vi "Omniax_mDrive_XYZR_MM_BR_RES_2_NC_GR_pxi_Acc3_preset.vi"() -> ()   [LabVIEW 2010]
uses:
  <vilib>/Utility/file.llb/Read From Spreadsheet File (I64).vi
  <vilib>/Utility/file.llb/Read From Spreadsheet File (string).vi
  <vilib>/Instr/_visa.llb/VISA Configure Serial Port (Instr).vi
  <vilib>/Utility/file.llb/Write To Spreadsheet File (I64).vi
  <vilib>/Utility/file.llb/Write To Spreadsheet File (string).vi
panel:
  out "R Velocity MVdeg/sec":dbl format="%.3f"
  out "R Position MV deg":dbl
  out "Z Velocity MV mm/sec":dbl format="%.3f"
  out "Z Position MV mm":dbl
  out "Y Velocity MV mm/sec":dbl format="%.3f"
  out "Y Position MV mm":dbl
  out "X Velocity MV mm/sec":dbl format="%.3f"
  out "X Position MV mm":dbl
  out "Presets":i32[][](array[numeric])
  in  "stop":bool
  in  "Tab Control 3":enum32{"Status", "Reset"}(tab)
  out "Y in Range":bool
  out "Y Scan":bool
  out "Y in Motion":bool
  out "Y Backlash corr":bool
  out "X  in Range":bool
  out "X Scan":bool
  out "X  in Motion":bool
  out "X Backlash corr":bool
  out "Z in Range":bool
  out "Z Scan":bool
  out "Z in Motion":bool
  out "Z Backlash corr":bool
  out "R in Range":bool
  out "R Scan":bool
  out "R in Motion":bool
  out "R Backlash corr":bool
  out "X Ready":bool
  out "Y Ready":bool
  out "Z Ready":bool
  out "R Ready":bool
  in  "Reset Y Position mm":dbl
  out "Reset Y Motor Steps":i32
  in  "Reset X Position mm":dbl
  out "Reset X Motor Steps":i32
  in  "Reset Z Position mm":dbl
  out "Reset Z Motor Steps":i32
  in  "Reset R Position deg":dbl
  out "Reset R Motor Steps":i32
  in  "Reset":bool
  in  "Tab Control 2":enum32{"mm", "step"}(tab)
  in  "X Scan Length SP mm":dbl
  in  "X Scan Velocity SP mm/sec":dbl
  in  "X Scan set":bool
  in  "Y Scan Length SP mm":dbl
  in  "Y Scan Velocity SP mm/sec":dbl
  in  "Y Scan set":bool
  in  "Z Scan Length SP mm":dbl
  in  "Z Scan Velocity SP mm/sec":dbl
  in  "Z Scan set":bool
  in  "R Scan Length SP deg":dbl
  in  "R Scan Velocity SP deg/sec":dbl
  in  "R Scan set":bool
  in  "X Scan Velocity SP steps/sec":i32=1 min=1 max=102400 step=1
  in  "X Scan Length SP steps":i32 min=-2304000 max=2304000 step=100
  out "X Scan length MV mm":dbl
  out "X Scan velocity MV mm/sec":dbl format="%#_6f"
  in  "Y Scan Velocity SP steps/sec":i32=1 min=1 max=102400 step=1
  in  "Y Scan Length SP steps":i32 min=-2304000 max=2304000 step=100
  out "Y Scan length MV mm":dbl
  out "Y Scan velocity MV mm/sec":dbl format="%#_6f"
  in  "Z Scan Velocity SP steps/sec":i32=1 min=1 max=102400 step=1
  in  "Z Scan Length SP steps":i32 min=-5120000 max=97280000 step=100
  out "Z Scan length MV mm":dbl
  out "Z Scan velocity MV mm/sec":dbl format="%#_6f"
  in  "R Scan Velocity SP steps/sec":i32=1 min=1 max=102400 step=1
  in  "R Scan Length SP steps":i32 min=-6144000 max=0 step=100
  out "R Scan length MV deg":dbl
  out "R Scan velocity MV deg/sec":dbl format="%#_6f"
  out "atan Y/Z":dbl
  in  "Tab Control":enum32{"mm", "preset", "step"}(tab)
  in  "X Position SP mm":dbl
  in  "X Velocity SP mm/sec":dbl
  in  "X Move Set":bool
  in  "Y Move Set":bool
  in  "Y Position SP mm":dbl
  in  "Y Velocity SP mm/sec":dbl
  in  "Z Position SP mm":dbl
  in  "Z Velocity SP mm/sec":dbl
  in  "Z Move Set":bool
  in  "R Position SP deg":dbl
  in  "R Velocity SP deg/sec":dbl
  in  "R Move Set":bool
  in  "Add Button":bool
  in  "String":string
  in  "Delete Button":bool
  in  "Preset positions":i32(ring) items=["ZERO", "Default", "CDOSE", "QMS", "test", "test2", "test3", "yag position", "Sample Long Edge  ", "SPUTTER POS"]
  in  "Set Button":bool
  in  "X Velocity SP step/sec":i32 min=1 max=128000
  in  "Y Velocity SP step/sec":i32 min=1 max=128000
  in  "Z Velocity SP step/sec":i32 min=1 max=204800
  in  "R Velocity SP step/sec":i32 min=1 max=20000
  in  "Y Step SP":i32=-20000 min=-2304000 max=2304000 step=500
  in  "X Step SP":i32=-20000 min=-2304000 max=2304000 step=500
  in  "Z Step SP":i32=-20000 min=0 max=102400000 step=500
  in  "R Step SP":i32=-20000 min=-6144000 max=6144000 step=500
  out "X Step PV":i32 max=2000
  out "Y Step PV":i32 max=2000
  out "Z Step PV":i32 max=2000
  out "R Step PV":i32 max=2000
  in  "Clear ZY":bool
  out "ZY Graph":cluster{"Y":dbl[], "Y":dbl[]}[](graph)
  out "ZR Graph":cluster{"Y":dbl[], "Y":dbl[]}[](graph)
  out "XY Graph":cluster{"Y":dbl[], "Y":dbl[]}[](graph)
  out "X Scan Duration":dbl
  out "Y Scan Duration":dbl
  out "Z Scan Duration":dbl
  out "R Scan Duration":dbl
  out "R Backlash steps/sec":i32
  out "R Backlash":i32
  out "R Holding Current %":i32
  out "R Run Current %":i32
  out "R offset deg":dbl
  out "R deg/rev":dbl
  out "R steps/rev":u32
  out "R velocity PV step/sec":i32
  out "R MINPOS":i32=-94296
  out "R MAXPOS":i32=-34296
  out "R COM PORT":refnum<visa-resource-name>="COM5"
  in  "R Scan OK":bool
  in  "R Go":bool
  out "R Position deg PV":dbl
  out "Z COM PORT":refnum<visa-resource-name>="COM5"
  out "Z Backlash steps/sec":i32
  out "Z Backlash":i32
  out "Z Holding Current %":i32
  out "Z Run Current %":i32
  out "Z offset mm":dbl
  out "Z mm/rev":dbl
  out "Z steps/rev":u32
  out "Z  velocity PV step/sec":i32
  out "Z MINPOS":i32=-94296
  out "Z MAXPOS":i32=-34296
  in  "Z Scan OK":bool
  in  "Z Go":bool
  out "Z Position mm PV":dbl
  out "X Position mm PV":dbl
  out "X velocity PV step/sec":i32
  in  "X Scan OK":bool
  in  "X Go":bool
  out "X Backlash steps/sec":i32
  out "X Backlash":i32
  out "X Holding Current %":i32
  out "X Run Current %":i32
  out "X offset mm":dbl
  out "X mm/rev":dbl
  out "X steps/rev":u32
  out "X MAXPOS":i32=-34296
  out "X MINPOS":i32=-94296
  out "X COM PORT":refnum<visa-resource-name>="COM5"
  out "Y Backlash steps/sec":i32
  out "Y Backlash":i32
  out "Y Holding Current %":i32
  out "Y Run Current %":i32
  in  "Scan Cancel":bool
  out "Y Position mm PV":dbl
  out "Y offset mm":dbl
  out "Y mm/rev":dbl
  out "Y steps/rev":u32
  out "Y velocity PV step/sec":i32
  in  "Y Scan OK":bool
  in  "Scan Go":bool
  in  "Stop":bool
  in  "Y Go":bool
  out "Y MINPOS":i32=-94296
  out "Y MAXPOS":i32=-34296
  out "Y COM PORT":refnum<visa-resource-name>="COM5"
  # "Current position"
  # "Goto position"
  # "MX"
  # "MY"
  # "MZ"
  # "MR"
  # "L"
  # "M"
  # "B"
  # "S"
  # "R"
  # "Preset position"
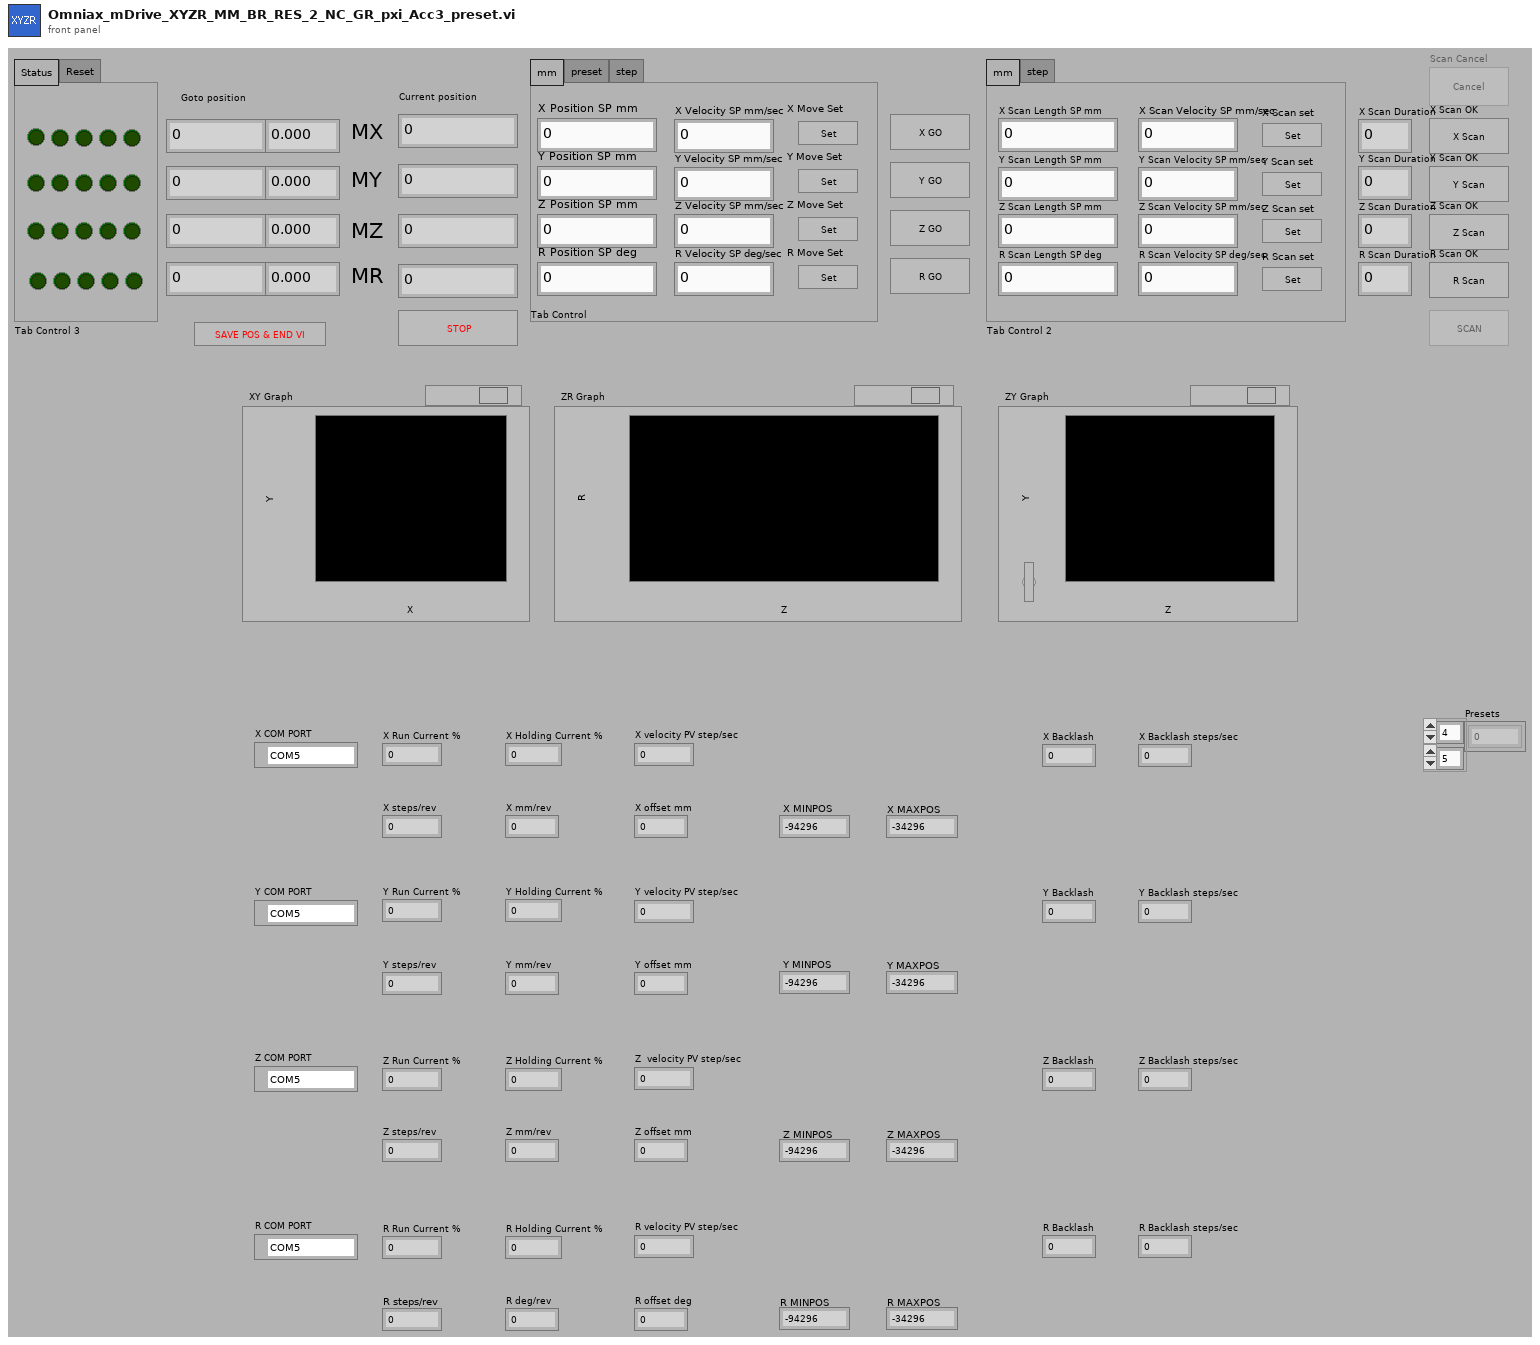
[diagram p1: front panel]
types:
  T1 = enum16{"Stop", "Reset", "Run Current", "Holding Current", "Accel Rate", "Decel Rate", "Move to Relative Position", "Move to Absolute Position", "Echo Mode", "Print Parameter", "Send String", "Microstep Resolution", "Set Current Position", "Max Velocity"}
  T2 = enum8{"Enabled", "Disabled", "Disabled and Grayed Out"}
  T3 = cluster{"first row[0]":i64, "first row[1]":i64, "first row[2]":i64, "first row[3]":i64, "first row[4]":i64, "first row[5]":i64, "first row[6]":i64, "first row[7]":i64, "first row[8]":i64}
  T4 = cluster{"Value[0]":i32, "Value[1]":i32, "Value[2]":i32, "Value[3]":i32, "Value[4]":i32, "Value[5]":i32, "Value[6]":i32, "Value[7]":i32, "Value[8]":i32}
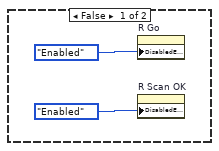
[diagram p5: hidden frame]
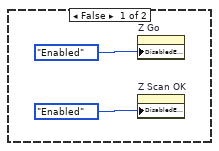
[diagram p8: hidden frame]
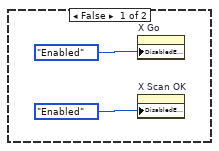
[diagram p11: hidden frame]
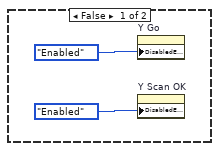
[diagram p14: hidden frame]
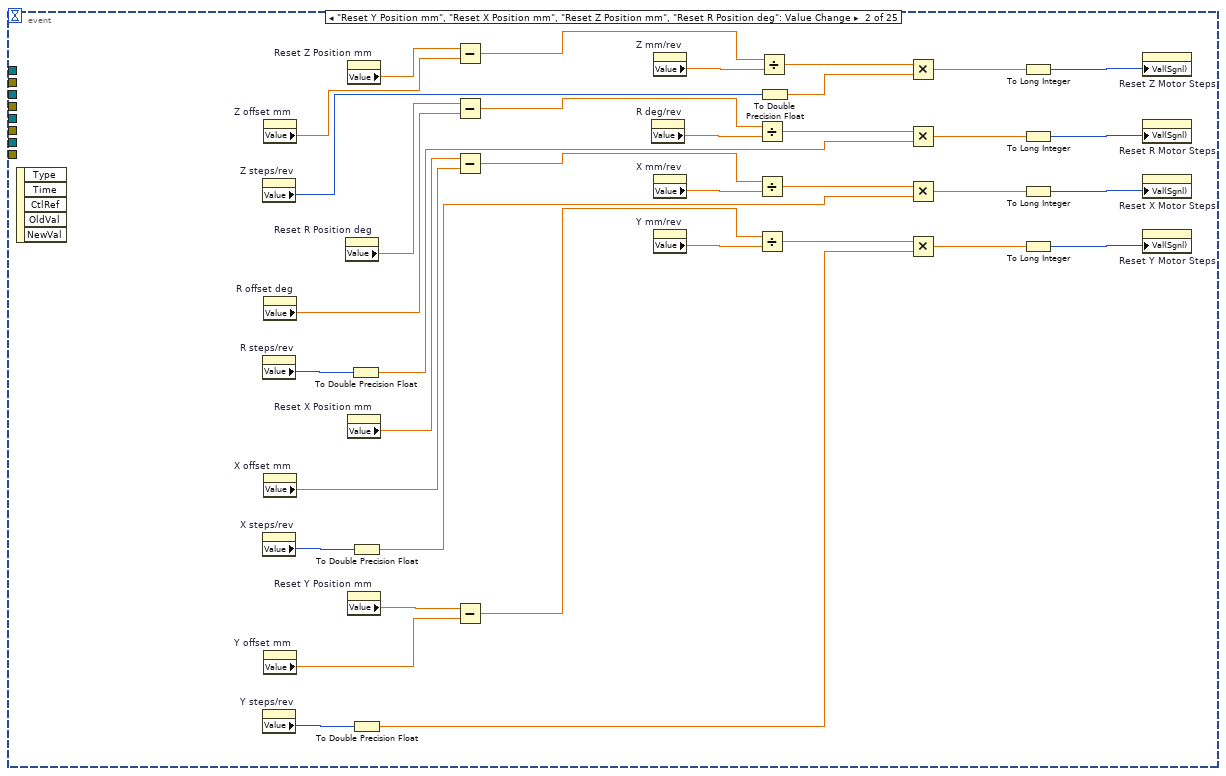
[diagram p17: hidden frame]
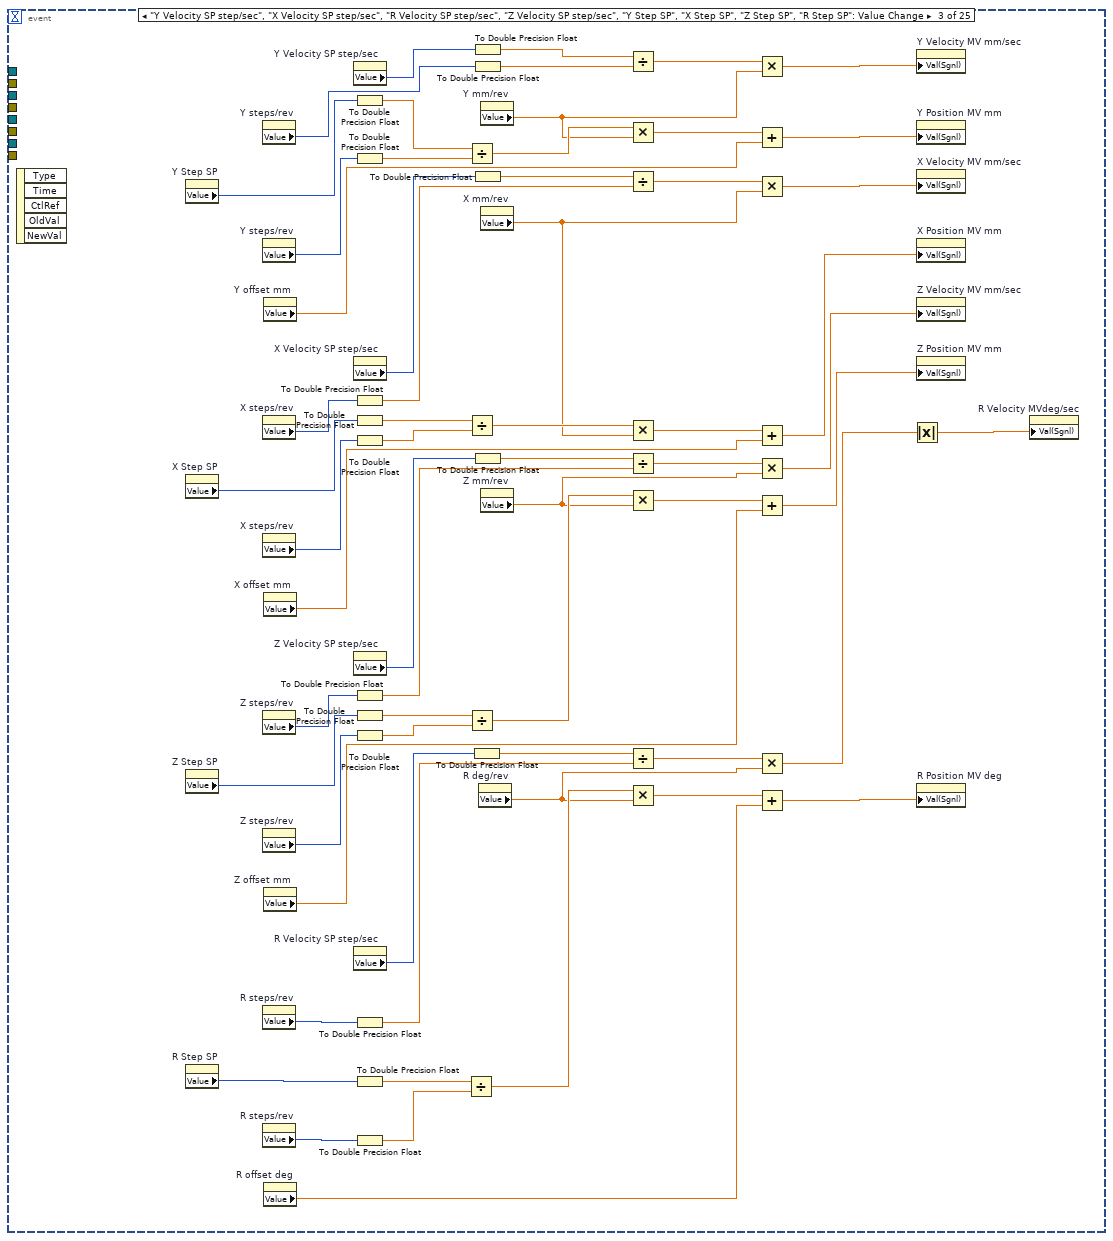
[diagram p18: hidden frame]
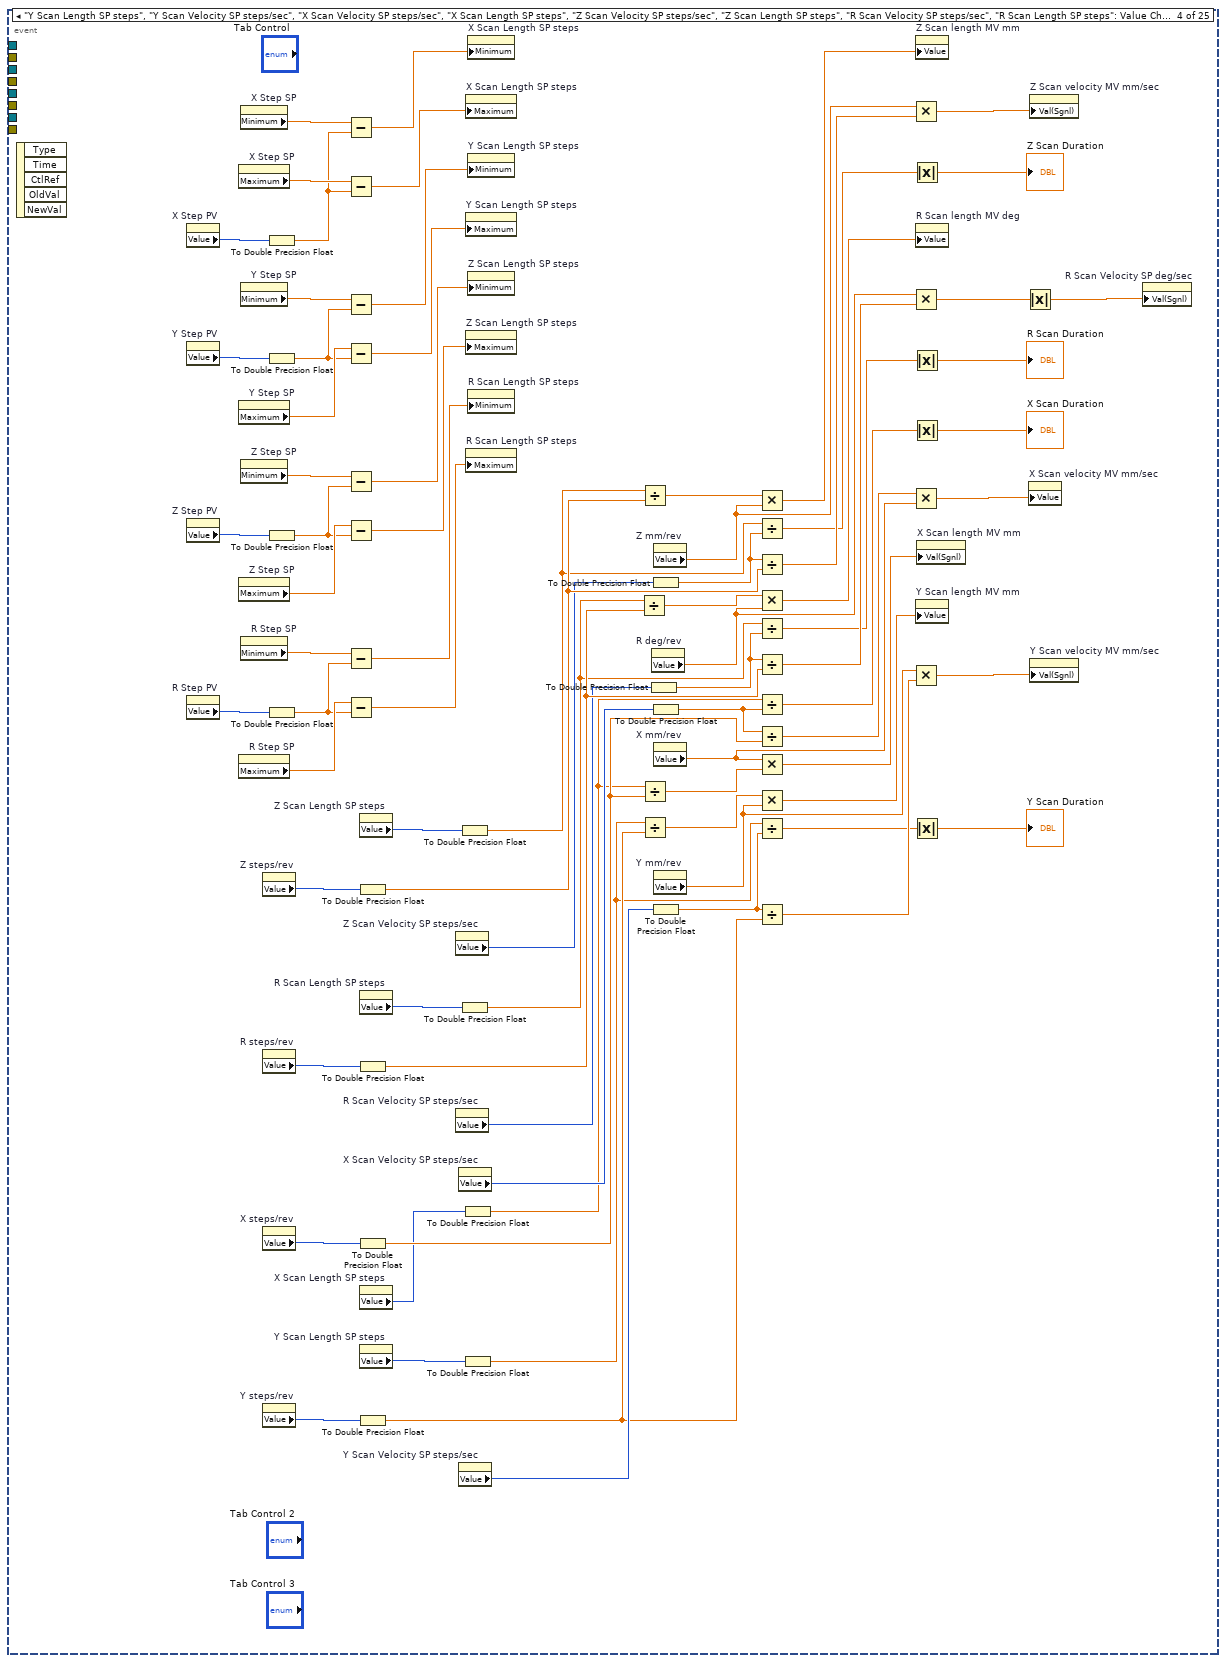
[diagram p19: hidden frame]
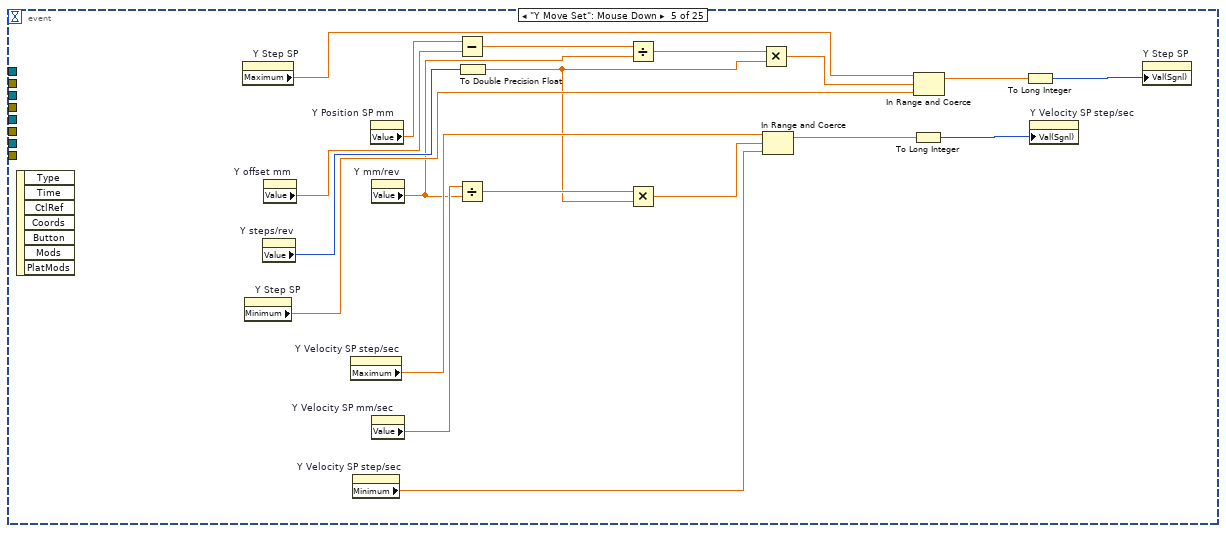
[diagram p20: hidden frame]
diagram:
  w1 = 0 ("dimension size")
  n1 = property on="R Step SP" class="DigNum (strict)"("Maximum"=6144000 ("upper limit")) -> ()  [unwired: 2 in, 2 out]
  n2 = property on="R Step SP" class="DigNum (strict)"("Minimum"=-6144000 ("lower limit")) -> ()  [unwired: 2 in, 2 out]
  n3 = flat-sequence {
    tunnel: [w105] -> w35
    tunnel: [w104] -> w34
    tunnel: [w113] -> w53
    tunnel: [w115] -> w51
    tunnel: w35 -> [w114]
    tunnel: w34 -> [w116]
    tunnel: w53 -> [w120]
    tunnel: [w121] -> w52
    tunnel: w51 -> [w119]
    tunnel: [w122] -> w50
    tunnel: [w133] -> w70
    tunnel: [w135] -> w69
    tunnel: w52 -> [w134]
    tunnel: w50 -> [w129]
    tunnel: w70 -> [w142]
    tunnel: [w141] -> w68
    tunnel: w69 -> [w139]
    tunnel: [w140] -> w67
    tunnel: [w152] -> w66
    tunnel: [w153] -> w65
    tunnel: w68 -> [w151]
    tunnel: w67 -> [w150]
    tunnel: w66 -> [w163]
    tunnel: w65 -> [w162]
    tunnel: [w165] -> w64
    tunnel: [w164] -> w63
    tunnel: [w159] -> w62
    tunnel: [w172] -> w58
    tunnel: [w173] -> w59
    tunnel: w64 -> [w173]
    tunnel: w63 -> [w172]
    tunnel: w62 -> [w170]
    frame #0 {
      w112 = refnum<visa-resource-name> "COM7" ("COM PORT")
      w110 = u16 0 items=["None", "XON/XOFF", "RTS/CTS", "XON/XOFF & RTS/CTS", "DTR/DSR", "XON/XOFF & DTR/DSR"] ("flow control (0:none)")
      w109 = u16 10 items=["1.0"=10, "1.5"=15, "2.0"=20] ("stop bits (10: 1 bit)")
      # "Stop bits"
      n4 = call-poly "VISA Configure Serial Port"("VISA resource name"=w112, "timeout (10sec)"=u32 10000, "baud rate (9600)"=u32 9600, "data bits (8)"=u16 8, "parity (0:none)"=enum16{"None", "Odd", "Even", "Mark", "Space"}."None", "stop bits (10: 1 bit)"=w109, "flow control (0:none)"=w110) -> ("VISA resource name out"=w105:refnum<visa-resource-name>, "error out"=w104:errorcluster)  [unwired: 7 in]
      "R COM PORT" <- w112
    }
    frame #1 {
      n5 = call "mDrive Send Command.vi"("error in (no error)"=w116, "Extra"="EM=2", "Command"=T1."Send String", "VISA resource name"=w114) -> ("error out"=w115:errorcluster, "VISA resource name out"=w113:refnum<visa-resource-name>)  [unwired: 3 in, 1 out]
    }
    frame #2 {
      # "pr=1000000"
      n6 = Number To Decimal String(number=100000) -> (decimal integer string=w124:string)  [unwired: 1 in]
      n7 = call "mDrive Send Command.vi"("error in (no error)"=w119, "Extra"=w124, "Command"=T1."Accel Rate", "VISA resource name"=w120) -> ("error out"=w123:errorcluster, "VISA resource name out"=w128:refnum<visa-resource-name>)  [unwired: 3 in, 1 out]
      n8 = call "mDrive Send Command.vi"("error in (no error)"=w123, "Extra"=w124, "Command"=T1."Decel Rate", "VISA resource name"=w128) -> ("error out"=w122:errorcluster, "VISA resource name out"=w121:refnum<visa-resource-name>)  [unwired: 3 in, 1 out]
    }
    frame #3 {
      # "Run Current %"
      n9 = property on="R Run Current %" class="DigNum (strict)"() -> ("Value"=w131:i32)  [unwired: 2 in, 2 out]
      n10 = Number To Decimal String(number=w131) -> (decimal integer string=w132:string)  [unwired: 1 in]
      n11 = call "mDrive Send Command.vi"("error in (no error)"=w129, "Extra"=w132, "Command"=T1."Run Current", "VISA resource name"=w134) -> ("error out"=w135:errorcluster, "VISA resource name out"=w133:refnum<visa-resource-name>)  [unwired: 3 in, 1 out]
    }
    frame #4 {
      # "Holding Current %"
      n12 = property on="R Holding Current %" class="DigNum (strict)"() -> ("Value"=w137:i32)  [unwired: 2 in, 2 out]
      n13 = Number To Decimal String(number=w137) -> (decimal integer string=w138:string)  [unwired: 1 in]
      n14 = call "mDrive Send Command.vi"("error in (no error)"=w139, "Extra"=w138, "Command"=T1."Holding Current", "VISA resource name"=w142) -> ("error out"=w140:errorcluster, "VISA resource name out"=w141:refnum<visa-resource-name>)  [unwired: 3 in, 1 out]
    }
    frame #5 {
      # "Print Velocity Max"
      # "Velocity Max"
      n15 = property on="R Velocity SP step/sec" class="DigNum (strict)"() -> ("Value"=w149:i32)  [unwired: 2 in, 2 out]
      n16 = Number To Decimal String(number=w149) -> (decimal integer string=w148:string)  [unwired: 1 in]
      n17 = call "mDrive Send Command.vi"("error in (no error)"=w150, "Extra"=w148, "Command"=T1."Max Velocity", "VISA resource name"=w151) -> ("error out"=w146:errorcluster, "VISA resource name out"=w156:refnum<visa-resource-name>)  [unwired: 3 in, 1 out]
      n18 = call "mDrive Send Command.vi"("error in (no error)"=w146, "Extra"="VM", "Command"=T1."Print Parameter", "VISA resource name"=w156) -> ("error out"=w153:errorcluster, "read buffer"=w154:string, "VISA resource name out"=w152:refnum<visa-resource-name>)  [unwired: 3 in]
      n19 = Decimal String To Number(string=w154, offset=0) -> (number=w147:i32)  [unwired: 1 in, 1 out]
      n20 = property on="R velocity PV step/sec" class="DigNum (strict)"("Val(Sgnl)"=w147) -> ()  [unwired: 2 in, 2 out]
    }
    frame #6 {
      # "PRINT POSITION"
      n21 = call "mDrive Send Command.vi"("error in (no error)"=w162, "Extra"="P", "Command"=T1."Print Parameter", "VISA resource name"=w163) -> ("error out"=w164:errorcluster, "read buffer"=w161:string, "VISA resource name out"=w165:refnum<visa-resource-name>)  [unwired: 3 in]
      n22 = Decimal String To Number(string=w161, offset=0) -> (number=w159:i32)  [unwired: 1 in, 1 out]
    }
    frame #7 {
      n23 = property on="R Step SP" class="DigNum (strict)"("Val(Sgnl)"=w170) -> ()  [unwired: 2 in, 2 out]
      n24 = property on="R Step SP" class="DigNum (strict)"() -> ("Maximum"=w169:dbl)  [unwired: 2 in, 2 out]
      n25 = property on="R Step SP" class="DigNum (strict)"() -> ("Minimum"=w168:dbl)  [unwired: 2 in, 2 out]
      n26 = To Long Integer(number=w169) -> (32bit integer=w166:i32)
      "R MAXPOS" <- w166
      n27 = To Long Integer(number=w168) -> (32bit integer=w167:i32)
      "R MINPOS" <- w167
      n28 = In Range and Coerce(upper limit=w166, x=w170, lower limit=w167) -> (In Range?=w171:bool)  [unwired: 1 out]
      n29 = property on="R in Range" class="Bool (strict)"("Val(Sgnl)"=w171) -> ()  [unwired: 2 in, 2 out]
    }
  }
  n30 = flat-sequence {
    frame #0 {
      w179 = -3.0 ("R deg/rev")
      w177 = u32 51200 ("step/rev")
      w181 = 10000 ("Value (Signaling)")
      n31 = To Double Precision Float(number=w181) -> (double precision float=w183:dbl)
      n32 = To Double Precision Float(number=w177) -> (double precision float=w178:dbl)
      n33 = property on="R Velocity SP step/sec" class="DigNum (strict)"("Val(Sgnl)"=w181) -> ()  [unwired: 2 in, 2 out]
      n34 = property on="R Velocity SP step/sec" class="DigNum (strict)"("Minimum"=1.0 ("Data Entry Limits:Minimum")) -> ()  [unwired: 2 in, 2 out]
      n35 = Divide(x=w183, y=w178) -> (x/y=w182:dbl)
      n36 = property on="R Velocity SP step/sec" class="DigNum (strict)"("Maximum"=w183) -> ()  [unwired: 2 in, 2 out]
      n37 = Multiply(x=w182, y=w179) -> (x*y=w180:dbl)
      n38 = Absolute Value(x=w180) -> (abs(x)=w174:dbl)
      n39 = property on="R Velocity SP deg/sec" class="DigNum (strict)"("Val(Sgnl)"=w174) -> ()  [unwired: 2 in, 2 out]
      "R offset deg" <- 0.0 ("R offset deg")
      "R deg/rev" <- w179
      "R steps/rev" <- w177
    }
  }
  n40 = flat-sequence {
    frame #0 {
      w185 = 0.2 ("Z mm/rev")
      w184 = u32 51200 ("step/rev")
      w186 = 204800 ("Value (Signaling)")
      n41 = To Double Precision Float(number=w186) -> (double precision float=w190:dbl)
      n42 = To Double Precision Float(number=w184) -> (double precision float=w189:dbl)
      n43 = property on="Z Velocity SP step/sec" class="DigNum (strict)"("Val(Sgnl)"=w186) -> ()  [unwired: 2 in, 2 out]
      n44 = property on="Z Velocity SP step/sec" class="DigNum (strict)"("Minimum"=1.0 ("Data Entry Limits:Minimum")) -> ()  [unwired: 2 in, 2 out]
      n45 = Divide(x=w190, y=w189) -> (x/y=w187:dbl)
      n46 = property on="Z Velocity SP step/sec" class="DigNum (strict)"("Maximum"=w190) -> ()  [unwired: 2 in, 2 out]
      n47 = Multiply(x=w187, y=w185) -> (x*y=w188:dbl)
      n48 = property on="Z Velocity SP mm/sec" class="DigNum (strict)"("Val(Sgnl)"=w188) -> ()  [unwired: 2 in, 2 out]
      "Z offset mm" <- 0.0 ("Z offset mm")
      "Z mm/rev" <- w185
      "Z steps/rev" <- w184
    }
  }
  n49 = flat-sequence {
    frame #0 {
      n50 = property on="X Backlash corr" class="Bool (strict)"("Val(Sgnl)"=FALSE ("Value (Signaling)")) -> ()  [unwired: 2 in, 2 out]
      n51 = property on="Y Backlash corr" class="Bool (strict)"("Val(Sgnl)"=FALSE ("Value (Signaling)")) -> ()  [unwired: 2 in, 2 out]
      n52 = property on="R Backlash corr" class="Bool (strict)"("Val(Sgnl)"=FALSE ("Value (Signaling)")) -> ()  [unwired: 2 in, 2 out]
      n53 = property on="Z Backlash corr" class="Bool (strict)"("Val(Sgnl)"=FALSE ("Value (Signaling)")) -> ()  [unwired: 2 in, 2 out]
      "Z Backlash steps/sec" <- 25600 ("Z Backlash steps/sec")
      "Z Backlash" <- -12800 ("Z Backlash")
      "X Backlash steps/sec" <- 25600 ("Value (Signaling)")
      "X Backlash" <- 5120 ("Backlash2")
      "Y Backlash" <- -5120 ("Backlash2")
      "Y Backlash steps/sec" <- 25600 ("Value (Signaling)")
      "R Backlash steps/sec" <- 6400 ("R Backlash steps/sec")
      "R Backlash" <- -12800 ("R Backlash")
    }
  }
  n54 = flat-sequence {
    frame #0 {
      "Z Holding Current %" <- 20 ("Z Holding Current %")
      "Z Run Current %" <- 40 ("Z Run Current %")
      "X Run Current %" <- 40 ("Run Current %")
      "X Holding Current %" <- 20 ("Holding Current %")
      "Y Run Current %" <- 40 ("Run Current %")
      "Y Holding Current %" <- 20 ("Holding Current %")
      "R Holding Current %" <- 20 ("R Holding Current %")
      "R Run Current %" <- 75 ("R Run Current %")
    }
  }
  n55 = flat-sequence {
    frame #0 {
      n56 = property on="Y Scan" class="Bool (strict)"("Val(Sgnl)"=FALSE ("Value (Signaling)")) -> ()  [unwired: 2 in, 2 out]
      n57 = property on="X Scan Velocity SP mm/sec" class="DigNum (strict)"("Val(Sgnl)"=0.1 ("Value (Signaling)")) -> ()  [unwired: 2 in, 2 out]
      n58 = property on="Z Scan" class="Bool (strict)"("Val(Sgnl)"=FALSE ("Value (Signaling)")) -> ()  [unwired: 2 in, 2 out]
      n59 = property on="X Scan" class="Bool (strict)"("Val(Sgnl)"=FALSE ("Value (Signaling)")) -> ()  [unwired: 2 in, 2 out]
      n60 = property on="Z Scan Velocity SP mm/sec" class="DigNum (strict)"("Val(Sgnl)"=0.1 ("Value (Signaling)")) -> ()  [unwired: 2 in, 2 out]
      n61 = property on="R Velocity SP deg/sec" class="DigNum (strict)"("Val(Sgnl)"=0.1 ("Value (Signaling)")) -> ()  [unwired: 2 in, 2 out]
      n62 = property on="R Scan" class="Bool (strict)"("Val(Sgnl)"=FALSE ("Value (Signaling)")) -> ()  [unwired: 2 in, 2 out]
      n63 = property on="Y Scan Velocity SP mm/sec" class="DigNum (strict)"("Val(Sgnl)"=0.1 ("Value (Signaling)")) -> ()  [unwired: 2 in, 2 out]
      n64 = property on="Scan Go" class="Bool"("DisabledEnum"=T2."Disabled and Grayed Out" ("Disabled")) -> ()  [unwired: 2 in, 2 out]
      n65 = property on="Scan Cancel" class="Bool"("DisabledEnum"=T2."Disabled and Grayed Out" ("Disabled")) -> ()  [unwired: 2 in, 2 out]
    }
  }
  n66 = flat-sequence {
    frame #0 {
      w225 = 0.2 ("MM/rev")
      w228 = u32 51200 ("step/rev")
      w223 = 128000 ("Value (Signaling)")
      # "a=1000000"
      n67 = property on="X Velocity SP step/sec" class="DigNum (strict)"("Minimum"=1.0 ("Data Entry Limits:Minimum")) -> ()  [unwired: 2 in, 2 out]
      n68 = To Double Precision Float(number=w223) -> (double precision float=w229:dbl)
      n69 = To Double Precision Float(number=w228) -> (double precision float=w227:dbl)
      n70 = property on="X Velocity SP step/sec" class="DigNum (strict)"("Val(Sgnl)"=w223) -> ()  [unwired: 2 in, 2 out]
      n71 = Divide(x=w229, y=w227) -> (x/y=w224:dbl)
      n72 = property on="X Velocity SP step/sec" class="DigNum (strict)"("Maximum"=w229) -> ()  [unwired: 2 in, 2 out]
      n73 = Multiply(x=w224, y=w225) -> (x*y=w226:dbl)
      n74 = property on="X Velocity SP mm/sec" class="DigNum (strict)"("Val(Sgnl)"=w226) -> ()  [unwired: 2 in, 2 out]
      "X offset mm" <- 0.0 ("offset")
      "X steps/rev" <- w228
      "X mm/rev" <- w225
    }
  }
  n75 = flat-sequence {
    frame #0 {
      w234 = 0.2 ("MM/rev")
      w237 = u32 51200 ("step/rev")
      w232 = 128000 ("Value (Signaling)")
      n76 = To Double Precision Float(number=w232) -> (double precision float=w238:dbl)
      n77 = To Double Precision Float(number=w237) -> (double precision float=w236:dbl)
      n78 = property on="Y Velocity SP step/sec" class="DigNum (strict)"("Val(Sgnl)"=w232) -> ()  [unwired: 2 in, 2 out]
      n79 = property on="Y Velocity SP step/sec" class="DigNum (strict)"("Minimum"=1.0 ("Data Entry Limits:Minimum")) -> ()  [unwired: 2 in, 2 out]
      n80 = Divide(x=w238, y=w236) -> (x/y=w233:dbl)
      n81 = property on="Y Velocity SP step/sec" class="DigNum (strict)"("Maximum"=w238) -> ()  [unwired: 2 in, 2 out]
      n82 = Multiply(x=w233, y=w234) -> (x*y=w235:dbl)
      n83 = property on="Y Velocity SP mm/sec" class="DigNum (strict)"("Val(Sgnl)"=w235) -> ()  [unwired: 2 in, 2 out]
      "Y offset mm" <- 0.0 ("offset")
      "Y steps/rev" <- w237
      "Y mm/rev" <- w234
    }
  }
  n84 = flat-sequence {
    tunnel: [w241] -> w39
    tunnel: [w242] -> w38
    tunnel: [w252] -> w45
    tunnel: [w251] -> w43
    tunnel: w39 -> [w253]
    tunnel: w38 -> [w250]
    tunnel: w45 -> [w263]
    tunnel: [w258] -> w44
    tunnel: w43 -> [w262]
    tunnel: [w262] -> w42
    tunnel: [w267] -> w79
    tunnel: [w269] -> w78
    tunnel: w44 -> [w268]
    tunnel: w42 -> [w270]
    tunnel: w79 -> [w277]
    tunnel: [w276] -> w77
    tunnel: w78 -> [w274]
    tunnel: [w275] -> w76
    tunnel: [w287] -> w75
    tunnel: [w288] -> w74
    tunnel: w77 -> [w286]
    tunnel: w76 -> [w285]
    tunnel: w75 -> [w298]
    tunnel: w74 -> [w297]
    tunnel: [w300] -> w73
    tunnel: [w299] -> w72
    tunnel: [w294] -> w71
    tunnel: [w307] -> w60
    tunnel: [w308] -> w61
    tunnel: w73 -> [w308]
    tunnel: w72 -> [w307]
    tunnel: w71 -> [w305]
    frame #0 {
      w249 = refnum<visa-resource-name> "COM6" ("COM PORT")
      w247 = u16 0 items=["None", "XON/XOFF", "RTS/CTS", "XON/XOFF & RTS/CTS", "DTR/DSR", "XON/XOFF & DTR/DSR"] ("flow control (0:none)")
      w246 = u16 10 items=["1.0"=10, "1.5"=15, "2.0"=20] ("stop bits (10: 1 bit)")
      # "Stop bits"
      n85 = call-poly "VISA Configure Serial Port"("VISA resource name"=w249, "timeout (10sec)"=u32 10000, "baud rate (9600)"=u32 9600, "data bits (8)"=u16 8, "parity (0:none)"=enum16{"None", "Odd", "Even", "Mark", "Space"}."None", "stop bits (10: 1 bit)"=w246, "flow control (0:none)"=w247) -> ("VISA resource name out"=w241:refnum<visa-resource-name>, "error out"=w242:errorcluster)  [unwired: 7 in]
      "Z COM PORT" <- w249
    }
    frame #1 {
      n86 = call "mDrive Send Command.vi"("error in (no error)"=w250, "Extra"="EM=2", "Command"=T1."Send String", "VISA resource name"=w253) -> ("error out"=w251:errorcluster, "VISA resource name out"=w252:refnum<visa-resource-name>)  [unwired: 3 in, 1 out]
    }
    frame #2 {
      n87 = Number To Decimal String(number=1000000) -> (decimal integer string=w256:string)  [unwired: 1 in]
      n88 = call "mDrive Send Command.vi"("Extra"=w256, "Command"=T1."Accel Rate", "VISA resource name"=w263) -> ("VISA resource name out"=w261:refnum<visa-resource-name>)  [unwired: 4 in, 2 out]
      n89 = call "mDrive Send Command.vi"("Extra"=w256, "Command"=T1."Decel Rate", "VISA resource name"=w261) -> ("VISA resource name out"=w258:refnum<visa-resource-name>)  [unwired: 4 in, 2 out]
    }
    frame #3 {
      # "Run Current %"
      n90 = property on="Z Run Current %" class="DigNum (strict)"() -> ("Value"=w265:i32)  [unwired: 2 in, 2 out]
      n91 = Number To Decimal String(number=w265) -> (decimal integer string=w266:string)  [unwired: 1 in]
      n92 = call "mDrive Send Command.vi"("error in (no error)"=w270, "Extra"=w266, "Command"=T1."Run Current", "VISA resource name"=w268) -> ("error out"=w269:errorcluster, "VISA resource name out"=w267:refnum<visa-resource-name>)  [unwired: 3 in, 1 out]
    }
    frame #4 {
      # "Holding Current %"
      n93 = property on="Z Run Current %" class="DigNum (strict)"() -> ("Value"=w272:i32)  [unwired: 2 in, 2 out]
      n94 = Number To Decimal String(number=w272) -> (decimal integer string=w273:string)  [unwired: 1 in]
      n95 = call "mDrive Send Command.vi"("error in (no error)"=w274, "Extra"=w273, "Command"=T1."Holding Current", "VISA resource name"=w277) -> ("error out"=w275:errorcluster, "VISA resource name out"=w276:refnum<visa-resource-name>)  [unwired: 3 in, 1 out]
    }
    frame #5 {
      # "Velocity Max"
      n96 = property on="Z Velocity SP step/sec" class="DigNum (strict)"() -> ("Value"=w284:i32)  [unwired: 2 in, 2 out]
      n97 = Number To Decimal String(number=w284) -> (decimal integer string=w283:string)  [unwired: 1 in]
      n98 = call "mDrive Send Command.vi"("error in (no error)"=w285, "Extra"=w283, "Command"=T1."Max Velocity", "VISA resource name"=w286) -> ("error out"=w281:errorcluster, "VISA resource name out"=w291:refnum<visa-resource-name>)  [unwired: 3 in, 1 out]
      n99 = call "mDrive Send Command.vi"("error in (no error)"=w281, "Extra"="VM", "Command"=T1."Print Parameter", "VISA resource name"=w291) -> ("error out"=w288:errorcluster, "read buffer"=w289:string, "VISA resource name out"=w287:refnum<visa-resource-name>)  [unwired: 3 in]
      n100 = Decimal String To Number(string=w289, offset=0) -> (number=w282:i32)  [unwired: 1 in, 1 out]
      n101 = property on="Z  velocity PV step/sec" class="DigNum (strict)"("Val(Sgnl)"=w282) -> ()  [unwired: 2 in, 2 out]
    }
    frame #6 {
      # "PRINT POSITION"
      n102 = call "mDrive Send Command.vi"("error in (no error)"=w297, "Extra"="P", "Command"=T1."Print Parameter", "VISA resource name"=w298) -> ("error out"=w299:errorcluster, "read buffer"=w296:string, "VISA resource name out"=w300:refnum<visa-resource-name>)  [unwired: 3 in]
      n103 = Decimal String To Number(string=w296, offset=0) -> (number=w294:i32)  [unwired: 1 in, 1 out]
    }
    frame #7 {
      n104 = property on="Z Step SP" class="DigNum (strict)"("Val(Sgnl)"=w305) -> ()  [unwired: 2 in, 2 out]
      n105 = property on="Z Step SP" class="DigNum (strict)"() -> ("Maximum"=w302:dbl)  [unwired: 2 in, 2 out]
      n106 = property on="Z Step SP" class="DigNum (strict)"() -> ("Minimum"=w304:dbl)  [unwired: 2 in, 2 out]
      n107 = To Long Integer(number=w302) -> (32bit integer=w303:i32)
      "Z MAXPOS" <- w303
      n108 = To Long Integer(number=w304) -> (32bit integer=w301:i32)
      "Z MINPOS" <- w301
      n109 = In Range and Coerce(upper limit=w303, x=w305, lower limit=w301) -> (In Range?=w306:bool)  [unwired: 1 out]
      n110 = property on="Z in Range" class="Bool (strict)"("Val(Sgnl)"=w306) -> ()  [unwired: 2 in, 2 out]
    }
  }
  n111 = flat-sequence {
    tunnel: [w310] -> w33
    tunnel: [w309] -> w32
    tunnel: [w320] -> w49
    tunnel: [w318] -> w47
    tunnel: w33 -> [w321]
    tunnel: w32 -> [w319]
    tunnel: w49 -> [w327]
    tunnel: [w328] -> w48
    tunnel: w47 -> [w324]
    tunnel: [w326] -> w46
    tunnel: [w337] -> w99
    tunnel: [w339] -> w97
    tunnel: w48 -> [w338]
    tunnel: w46 -> [w340]
    tunnel: w99 -> [w347]
    tunnel: [w346] -> w98
    tunnel: w97 -> [w344]
    tunnel: [w345] -> w96
    tunnel: [w357] -> w101
    tunnel: [w358] -> w100
    tunnel: w98 -> [w356]
    tunnel: w96 -> [w355]
    tunnel: w101 -> [w368]
    tunnel: w100 -> [w367]
    tunnel: [w370] -> w85
    tunnel: [w369] -> w84
    tunnel: [w364] -> w83
    tunnel: [w375] -> w102
    tunnel: [w376] -> w103
    tunnel: w85 -> [w376]
    tunnel: w84 -> [w375]
    tunnel: w83 -> [w371]
    frame #0 {
      w317 = refnum<visa-resource-name> "COM5" ("COM PORT")
      w315 = u16 0 items=["None", "XON/XOFF", "RTS/CTS", "XON/XOFF & RTS/CTS", "DTR/DSR", "XON/XOFF & DTR/DSR"] ("flow control (0:none)")
      w314 = u16 10 items=["1.0"=10, "1.5"=15, "2.0"=20] ("stop bits (10: 1 bit)")
      # "Stop bits"
      n112 = call-poly "VISA Configure Serial Port"("VISA resource name"=w317, "timeout (10sec)"=u32 10000, "baud rate (9600)"=u32 9600, "data bits (8)"=u16 8, "parity (0:none)"=enum16{"None", "Odd", "Even", "Mark", "Space"}."None", "stop bits (10: 1 bit)"=w314, "flow control (0:none)"=w315) -> ("VISA resource name out"=w310:refnum<visa-resource-name>, "error out"=w309:errorcluster)  [unwired: 7 in]
      "Y COM PORT" <- w317
    }
    frame #1 {
      n113 = call "mDrive Send Command.vi"("error in (no error)"=w319, "Extra"="EM=2", "Command"=T1."Send String", "VISA resource name"=w321) -> ("error out"=w318:errorcluster, "VISA resource name out"=w320:refnum<visa-resource-name>)  [unwired: 3 in, 1 out]
    }
    frame #2 {
      n114 = Number To Decimal String(number=1000000) -> (decimal integer string=w329:string)  [unwired: 1 in]
      n115 = call "mDrive Send Command.vi"("error in (no error)"=w324, "Extra"=w329, "Command"=T1."Accel Rate", "VISA resource name"=w327) -> ("error out"=w325:errorcluster, "VISA resource name out"=w333:refnum<visa-resource-name>)  [unwired: 3 in, 1 out]
      n116 = call "mDrive Send Command.vi"("error in (no error)"=w325, "Extra"=w329, "Command"=T1."Decel Rate", "VISA resource name"=w333) -> ("error out"=w326:errorcluster, "VISA resource name out"=w328:refnum<visa-resource-name>)  [unwired: 3 in, 1 out]
    }
    frame #3 {
      # "Run Current %"
      n117 = property on="Y Run Current %" class="DigNum (strict)"() -> ("Value"=w335:i32)  [unwired: 2 in, 2 out]
      n118 = Number To Decimal String(number=w335) -> (decimal integer string=w336:string)  [unwired: 1 in]
      n119 = call "mDrive Send Command.vi"("error in (no error)"=w340, "Extra"=w336, "Command"=T1."Run Current", "VISA resource name"=w338) -> ("error out"=w339:errorcluster, "VISA resource name out"=w337:refnum<visa-resource-name>)  [unwired: 3 in, 1 out]
    }
    frame #4 {
      # "Holding Current %"
      n120 = property on="Y Holding Current %" class="DigNum (strict)"() -> ("Value"=w342:i32)  [unwired: 2 in, 2 out]
      n121 = Number To Decimal String(number=w342) -> (decimal integer string=w343:string)  [unwired: 1 in]
      n122 = call "mDrive Send Command.vi"("error in (no error)"=w344, "Extra"=w343, "Command"=T1."Holding Current", "VISA resource name"=w347) -> ("error out"=w345:errorcluster, "VISA resource name out"=w346:refnum<visa-resource-name>)  [unwired: 3 in, 1 out]
    }
    frame #5 {
      # "Velocity Max"
      n123 = property on="Y Velocity SP step/sec" class="DigNum (strict)"() -> ("Value"=w354:i32)  [unwired: 2 in, 2 out]
      n124 = Number To Decimal String(number=w354) -> (decimal integer string=w353:string)  [unwired: 1 in]
      n125 = call "mDrive Send Command.vi"("error in (no error)"=w355, "Extra"=w353, "Command"=T1."Max Velocity", "VISA resource name"=w356) -> ("error out"=w351:errorcluster, "VISA resource name out"=w361:refnum<visa-resource-name>)  [unwired: 3 in, 1 out]
      n126 = call "mDrive Send Command.vi"("error in (no error)"=w351, "Extra"="VM", "Command"=T1."Print Parameter", "VISA resource name"=w361) -> ("error out"=w358:errorcluster, "read buffer"=w359:string, "VISA resource name out"=w357:refnum<visa-resource-name>)  [unwired: 3 in]
      n127 = Decimal String To Number(string=w359, offset=0) -> (number=w352:i32)  [unwired: 1 in, 1 out]
      n128 = property on="Y scan velocity MV step/sec" class="DigNum (strict)"("Val(Sgnl)"=w352) -> ()  [unwired: 2 in, 2 out]
    }
    frame #6 {
      # "PRINT POSITION"
      n129 = call "mDrive Send Command.vi"("error in (no error)"=w367, "Extra"="P", "Command"=T1."Print Parameter", "VISA resource name"=w368) -> ("error out"=w369:errorcluster, "read buffer"=w366:string, "VISA resource name out"=w370:refnum<visa-resource-name>)  [unwired: 3 in]
      n130 = Decimal String To Number(string=w366, offset=0) -> (number=w364:i32)  [unwired: 1 in, 1 out]
    }
    frame #7 {
      w373 = -2304000 ("lower limit")
      w374 = 2304000 ("upper limit")
      n131 = property on="Y Step SP" class="DigNum (strict)"("Val(Sgnl)"=w371) -> ()  [unwired: 2 in, 2 out]
      n132 = In Range and Coerce(upper limit=w374, x=w371, lower limit=w373) -> (In Range?=w372:bool)  [unwired: 1 out]
      n133 = property on="Y Step SP" class="DigNum (strict)"("Maximum"=w374) -> ()  [unwired: 2 in, 2 out]
      n134 = property on="Y Step SP" class="DigNum (strict)"("Minimum"=w373) -> ()  [unwired: 2 in, 2 out]
      n135 = property on="Y in Range" class="Bool (strict)"("Val(Sgnl)"=w372) -> ()  [unwired: 2 in, 2 out]
      "Y MINPOS" <- w373
      "Y MAXPOS" <- w374
    }
  }
  n136 = property on="Z Step SP" class="DigNum (strict)"("Minimum"=0 ("lower limit")) -> ()  [unwired: 2 in, 2 out]
  n137 = flat-sequence {
    tunnel: [w378] -> w37
    tunnel: [w377] -> w36
    tunnel: [w388] -> w57
    tunnel: [w386] -> w55
    tunnel: w37 -> [w389]
    tunnel: w36 -> [w387]
    tunnel: w57 -> [w393]
    tunnel: [w392] -> w56
    tunnel: w55 -> [w394]
    tunnel: [w396] -> w54
    tunnel: [w405] -> w95
    tunnel: [w407] -> w94
    tunnel: w56 -> [w406]
    tunnel: w54 -> [w408]
    tunnel: w95 -> [w415]
    tunnel: [w414] -> w93
    tunnel: w94 -> [w412]
    tunnel: [w413] -> w92
    tunnel: [w425] -> w91
    tunnel: [w426] -> w90
    tunnel: w93 -> [w424]
    tunnel: w92 -> [w423]
    tunnel: w91 -> [w436]
    tunnel: w90 -> [w435]
    tunnel: [w438] -> w82
    tunnel: [w437] -> w81
    tunnel: [w432] -> w80
    tunnel: [w443] -> w88
    tunnel: [w444] -> w89
    tunnel: w82 -> [w444]
    tunnel: w81 -> [w443]
    tunnel: w80 -> [w439]
    frame #0 {
      w385 = refnum<visa-resource-name> "COM4" ("COM PORT")
      w383 = u16 0 items=["None", "XON/XOFF", "RTS/CTS", "XON/XOFF & RTS/CTS", "DTR/DSR", "XON/XOFF & DTR/DSR"] ("flow control (0:none)")
      w382 = u16 10 items=["1.0"=10, "1.5"=15, "2.0"=20] ("stop bits (10: 1 bit)")
      # "Stop bits"
      n138 = call-poly "VISA Configure Serial Port"("VISA resource name"=w385, "timeout (10sec)"=u32 10000, "baud rate (9600)"=u32 9600, "data bits (8)"=u16 8, "parity (0:none)"=enum16{"None", "Odd", "Even", "Mark", "Space"}."None", "stop bits (10: 1 bit)"=w382, "flow control (0:none)"=w383) -> ("VISA resource name out"=w378:refnum<visa-resource-name>, "error out"=w377:errorcluster)  [unwired: 7 in]
      "X COM PORT" <- w385
    }
    frame #1 {
      n139 = call "mDrive Send Command.vi"("error in (no error)"=w387, "Extra"="EM=2", "Command"=T1."Send String", "VISA resource name"=w389) -> ("error out"=w386:errorcluster, "VISA resource name out"=w388:refnum<visa-resource-name>)  [unwired: 3 in, 1 out]
    }
    frame #2 {
      n140 = Number To Decimal String(number=1000000) -> (decimal integer string=w397:string)  [unwired: 1 in]
      n141 = call "mDrive Send Command.vi"("error in (no error)"=w394, "Extra"=w397, "Command"=T1."Accel Rate", "VISA resource name"=w393) -> ("error out"=w395:errorcluster, "VISA resource name out"=w401:refnum<visa-resource-name>)  [unwired: 3 in, 1 out]
      n142 = call "mDrive Send Command.vi"("error in (no error)"=w395, "Extra"=w397, "Command"=T1."Decel Rate", "VISA resource name"=w401) -> ("error out"=w396:errorcluster, "VISA resource name out"=w392:refnum<visa-resource-name>)  [unwired: 3 in, 1 out]
    }
    frame #3 {
      # "Run Current %"
      n143 = property on="X Run Current %" class="DigNum (strict)"() -> ("Value"=w403:i32)  [unwired: 2 in, 2 out]
      n144 = Number To Decimal String(number=w403) -> (decimal integer string=w404:string)  [unwired: 1 in]
      n145 = call "mDrive Send Command.vi"("error in (no error)"=w408, "Extra"=w404, "Command"=T1."Run Current", "VISA resource name"=w406) -> ("error out"=w407:errorcluster, "VISA resource name out"=w405:refnum<visa-resource-name>)  [unwired: 3 in, 1 out]
    }
    frame #4 {
      # "Holding Current %"
      n146 = property on="X Holding Current %" class="DigNum (strict)"() -> ("Value"=w410:i32)  [unwired: 2 in, 2 out]
      n147 = Number To Decimal String(number=w410) -> (decimal integer string=w411:string)  [unwired: 1 in]
      n148 = call "mDrive Send Command.vi"("error in (no error)"=w412, "Extra"=w411, "Command"=T1."Holding Current", "VISA resource name"=w415) -> ("error out"=w413:errorcluster, "VISA resource name out"=w414:refnum<visa-resource-name>)  [unwired: 3 in, 1 out]
    }
    frame #5 {
      # "Velocity Max"
      n149 = property on="X Velocity SP step/sec" class="DigNum (strict)"() -> ("Value"=w422:i32)  [unwired: 2 in, 2 out]
      n150 = Number To Decimal String(number=w422) -> (decimal integer string=w421:string)  [unwired: 1 in]
      n151 = call "mDrive Send Command.vi"("error in (no error)"=w423, "Extra"=w421, "Command"=T1."Max Velocity", "VISA resource name"=w424) -> ("error out"=w419:errorcluster, "VISA resource name out"=w429:refnum<visa-resource-name>)  [unwired: 3 in, 1 out]
      n152 = call "mDrive Send Command.vi"("error in (no error)"=w419, "Extra"="VM", "Command"=T1."Print Parameter", "VISA resource name"=w429) -> ("error out"=w426:errorcluster, "read buffer"=w427:string, "VISA resource name out"=w425:refnum<visa-resource-name>)  [unwired: 3 in]
      n153 = Decimal String To Number(string=w427, offset=0) -> (number=w420:i32)  [unwired: 1 in, 1 out]
      n154 = property on="X velocity PV step/sec" class="DigNum (strict)"("Val(Sgnl)"=w420) -> ()  [unwired: 2 in, 2 out]
    }
    frame #6 {
      # "PRINT POSITION"
      n155 = call "mDrive Send Command.vi"("error in (no error)"=w435, "Extra"="P", "Command"=T1."Print Parameter", "VISA resource name"=w436) -> ("error out"=w437:errorcluster, "read buffer"=w434:string, "VISA resource name out"=w438:refnum<visa-resource-name>)  [unwired: 3 in]
      n156 = Decimal String To Number(string=w434, offset=0) -> (number=w432:i32)  [unwired: 1 in, 1 out]
    }
    frame #7 {
      w441 = -2304000 ("lower limit")
      w442 = 2304000 ("upper limit")
      n157 = property on="X Step SP" class="DigNum (strict)"("Val(Sgnl)"=w439) -> ()  [unwired: 2 in, 2 out]
      n158 = In Range and Coerce(upper limit=w442, x=w439, lower limit=w441) -> (In Range?=w440:bool)  [unwired: 1 out]
      n159 = property on="X Step SP" class="DigNum (strict)"("Maximum"=w442) -> ()  [unwired: 2 in, 2 out]
      n160 = property on="X Step SP" class="DigNum (strict)"("Minimum"=w441) -> ()  [unwired: 2 in, 2 out]
      n161 = property on="X  in Range" class="Bool (strict)"("Val(Sgnl)"=w440) -> ()  [unwired: 2 in, 2 out]
      "X MINPOS" <- w441
      "X MAXPOS" <- w442
    }
  }
  n162 = property on="Z Step SP" class="DigNum (strict)"("Maximum"=102400000 ("upper limit")) -> ()  [unwired: 2 in, 2 out]
  n163 = call-poly <vilib>:"Read From Spreadsheet File.vi"("file path (dialog if empty)"=path "C:/Documents and Settings/b_ogasawara/Desktop/lv1/LV codes/IMS/POS.TXT") -> ("first row"=w19:i64[])  [unwired: 6 in, 4 out]
  n164 = call-poly <vilib>:"Read From Spreadsheet File.vi"("file path (dialog if empty)"=path "C:/Documents and Settings/b_ogasawara/Desktop/lv1/LV codes/IMS/PRESET.TXT") -> ("all rows"=w7:string[][])  [unwired: 6 in, 4 out]
  n165 = Array To Cluster(array=w19) -> (cluster=w18:T3)
  n166 = Transpose 2D Array(2D array=w7) -> (transposed array=w8:string[][])
  n167 = Unbundle(w18) -> ("first row[0]"=w16:i64, "first row[1]"=w15:i64, "first row[2]"=w14:i64, "first row[3]"=w13:i64)  [unwired: 5 out]
  n168 = Delete From Array(array=w8, index (row)=0) -> (deleted portion=w9:string[], array with subset deleted=w11:string[][])  [unwired: 2 in]
  n169 = property on="Reset X Motor Steps" class="DigNum (strict)"("Val(Sgnl)"=w16) -> ()  [unwired: 2 in, 2 out]
  n170 = property on="Reset Y Motor Steps" class="DigNum (strict)"("Val(Sgnl)"=w15) -> ()  [unwired: 2 in, 2 out]
  n171 = property on="Reset Z Motor Steps" class="DigNum (strict)"("Val(Sgnl)"=w14) -> ()  [unwired: 2 in, 2 out]
  n172 = property on="Reset R Motor Steps" class="DigNum (strict)"("Val(Sgnl)"=w13) -> ()  [unwired: 2 in, 2 out]
  n173 = Transpose 2D Array(2D array=w11) -> (transposed array=w12:string[][])
  n174 = property on="Preset positions" class="Ring (strict)"("Strings []"=w9) -> ()  [unwired: 2 in, 2 out]
  n175 = Decimal String To Number(string=w12) -> (number=w10:i32[][])  [unwired: 2 in, 1 out]
  n176 = Initialize Array(w1, w1, 4 ("dimension size")) -> (w4:i32[][])
  n177 = Build Array (concatenate)(w4, w10) -> (→"Presets":i32[][])
  n178 = while {
    tunnel: w103 -> [w463]
    tunnel: w102 -> [w466]
    tunnel: [w467] -> w26
    tunnel: [w465] -> w27
    tunnel: w89 -> [w462]
    tunnel: w88 -> [w461]
    tunnel: [w460] -> w87
    tunnel: [w459] -> w86
    tunnel: w61 -> [w458]
    tunnel: w60 -> [w457]
    tunnel: [w456] -> w29
    tunnel: [w455] -> w28
    tunnel: w59 -> [w454]
    tunnel: w58 -> [w453]
    tunnel: [w452] -> w25
    tunnel: [w451] -> w24
    stop <- "stop" stop-if-true
    n179 = property on="Preset positions" class="Ring (strict)"() -> ("Strings []"=w447:string[])  [unwired: 2 in, 2 out]
    n180 = event shown="[0] Timeout" {
      selector: _ -> [_ _ _ _ _ _ _ _ _ _ _ _ _ _ _ _ _ _ _ _ _ _ _ _ _]
      dyn-events: _ -> [_ _ _ _ _ _ _ _ _ _ _ _ _ _ _ _ _ _ _ _ _ _ _ _ _]
      timeout: 100 -> [_ _ _ _ _ _ _ _ _ _ _ _ _ _ _ _ _ _ _ _ _ _ _ _ _]
      tunnel: w466 -> [w568 _ _ _ _ _ _ _ _ _ _ _ w1409 _ _ _ _ w1658 _ _ w1753 w1769 w1813 w1890 w2134]
      tunnel: [w567 _ _ _ _ _ _ _ _ _ _ _ w1415 _ _ _ _ w1656 _ _ w1753 w1767 w1815 w1879 w2132] -> w467
      tunnel: w463 -> [w506 _ _ _ _ _ _ _ _ _ _ _ w1410 _ _ _ _ w1657 _ _ w1754 w1770 w1814 w1892 w2135]
      tunnel: [w566 _ _ _ _ _ _ _ _ _ _ _ w1416 _ _ _ _ w1653 _ _ w1754 w1768 w1816 w1880 w2133] -> w465
      tunnel: w462 -> [w505 _ _ _ _ _ _ _ _ _ _ _ _ _ _ w1567 w1622 _ _ _ _ w1764 w1806 w1896 w2131]
      tunnel: w461 -> [w543 _ _ _ _ _ _ _ _ _ _ _ _ _ _ w1566 w1621 _ _ _ _ w1763 w1805 w1894 w2130]
      tunnel: [w542 _ _ _ _ _ _ _ _ _ _ _ _ _ _ w1565 w1620 _ _ _ _ w1766 w1804 w1872 w2129] -> w460
      tunnel: [w541 _ _ _ _ _ _ _ _ _ _ _ _ _ _ w1564 w1619 _ _ _ _ w1765 w1803 w1870 w2128] -> w459
      tunnel: w458 -> [w515 _ _ _ _ _ _ _ _ _ _ _ _ w1461 _ _ _ _ w1688 _ _ w1762 w1800 w1888 w2127]
      tunnel: w457 -> [w518 _ _ _ _ _ _ _ _ _ _ _ _ w1460 _ _ _ _ w1687 _ _ w1761 w1799 w1886 w2126]
      tunnel: [w517 _ _ _ _ _ _ _ _ _ _ _ _ w1458 _ _ _ _ w1685 _ _ w1760 w1798 w1878 w2123] -> w456
      tunnel: [w516 _ _ _ _ _ _ _ _ _ _ _ _ w1459 _ _ _ _ w1686 _ _ w1759 w1797 w1877 w2122] -> w455
      tunnel: w454 -> [w514 _ _ _ _ _ _ _ _ _ _ _ _ _ w1514 _ _ _ _ w1722 _ w1758 w1794 w1883 w2125]
      tunnel: w453 -> [w513 _ _ _ _ _ _ _ _ _ _ _ _ _ w1513 _ _ _ _ w1721 _ w1757 w1793 w1881 w2124]
      tunnel: [w512 _ _ _ _ _ _ _ _ _ _ _ _ _ w1511 _ _ _ _ w1720 _ w1756 w1792 w1875 w2121] -> w452
      tunnel: [w511 _ _ _ _ _ _ _ _ _ _ _ _ _ w1512 _ _ _ _ w1719 _ w1755 w1791 w1874 w2120] -> w451
      event Timeout {
        n181 = event-data() -> ()  [unwired: 1 in, 2 out]
        n182 = flat-sequence {
          tunnel: [w864] -> w554
          tunnel: [w841] -> w553
          tunnel: [w853] -> w552
          tunnel: [w832] -> w551
          tunnel: w505 -> [w831]
          tunnel: w543 -> [w830]
          tunnel: w554 -> [w870]
          tunnel: [w870] -> w550
          tunnel: w553 -> [w869]
          tunnel: [w869] -> w549
          tunnel: w552 -> [w868]
          tunnel: [w868] -> w548
          tunnel: w551 -> [w865]
          tunnel: [w865] -> w547
          tunnel: w550 -> [w877]
          tunnel: [w878] -> w546
          tunnel: w549 -> [w880]
          tunnel: [w879] -> w545
          tunnel: w548 -> [w876]
          tunnel: [w875] -> w544
          tunnel: w547 -> [w875]
          tunnel: w546 -> [w890]
          tunnel: w545 -> [w891]
          tunnel: w544 -> [w893]
          tunnel: [w889] -> w541
          tunnel: [w888] -> w542
          frame #0 {
            w836 = 0.05 ("Delay Time (s)")
            n183 = property on="X Step SP" class="DigNum (strict)"() -> ("Maximum"=w855:dbl)  [unwired: 2 in, 2 out]
            n184 = property on="X Step SP" class="DigNum (strict)"() -> ("Minimum"=w857:dbl)  [unwired: 2 in, 2 out]
            n185 = property on="X steps/rev" class="DigNum (strict)"() -> ("Value"=w851:u32)  [unwired: 2 in, 2 out]
            n186 = property on="X offset mm" class="DigNum (strict)"() -> ("Value"=w847:dbl)  [unwired: 2 in, 2 out]
            n187 = To Long Integer(number=w855) -> (32bit integer=w854:i32)
            n188 = To Long Integer(number=w857) -> (32bit integer=w856:i32)
            n189 = To Double Precision Float(number=w851) -> (double precision float=w852:dbl)
            n190 = call "mDrive Send Command.vi"("error in (no error)"=w830, "Extra"="P", "Command"=T1."Print Parameter", "VISA resource name"=w831) -> ("error out"=w859:errorcluster, "read buffer"=w863:string, "VISA resource name out"=w861:refnum<visa-resource-name>)  [unwired: 3 in]
            n191 = call "Time Delay12"("error in (no error)"=w859, "Delay Time (s)"=w836) -> ("error out"=w858:errorcluster)  [unwired: 9 in]
            n192 = Decimal String To Number(string=w863, offset=0) -> (number=w843:i32)  [unwired: 1 in, 1 out]
            n193 = To Long Integer(number=w843) -> (32bit integer=w845:i32)
            n194 = property on="X Step PV" class="DigNum (strict)"("Val(Sgnl)"=w845) -> ()  [unwired: 2 in, 2 out]
            n195 = call "mDrive Send Command.vi"("error in (no error)"=w858, "Extra"="MV", "Command"=T1."Print Parameter", "VISA resource name"=w861) -> ("error out"=w860:errorcluster, "read buffer"=w829:string, "VISA resource name out"=w864:refnum<visa-resource-name>)  [unwired: 3 in]
            n196 = call "Time Delay11"("error in (no error)"=w860, "Delay Time (s)"=w836) -> ("error out"=w841:errorcluster)  [unwired: 9 in]
            n197 = In Range and Coerce(upper limit=w854, x=w845, lower limit=w856) -> (In Range?=w853:bool)  [unwired: 1 out]
            n198 = To Double Precision Float(number=w845) -> (double precision float=w846:dbl)
            n199 = Decimal String To Number(string=w829, offset=0 ("offset (0)")) -> (number=w835:i32)  [unwired: 1 in, 1 out]
            n200 = Not Equal?(x=w829, y="") -> (x != y?=w827:bool)
            n201 = property on="X  in Range" class="Bool (strict)"("Val(Sgnl)"=w853) -> ()  [unwired: 2 in, 2 out]
            n202 = property on="X Ready" class="Bool (strict)"("Val(Sgnl)"=w827) -> ()  [unwired: 2 in, 2 out]
            n203 = Divide(x=w846, y=w852) -> (x/y=w850:dbl)
            n204 = Number To Boolean Array(number=w835) -> (Boolean array=w834:bool[])
            n205 = property on="X mm/rev" class="DigNum (strict)"() -> ("Value"=w849:dbl)  [unwired: 2 in, 2 out]
            n206 = Index Array(array=w834, index=0) -> (element=w832:bool)
            n207 = Multiply(x=w850, y=w849) -> (x*y=w848:dbl)
            n208 = property on="X  in Motion" class="Bool (strict)"("Val(Sgnl)"=w832) -> ()  [unwired: 2 in, 2 out]
            n209 = Add(x=w848, y=w847) -> (x+y=w844:dbl)
            n210 = property on="X Position mm PV" class="DigNum (strict)"("Val(Sgnl)"=w844) -> ()  [unwired: 2 in, 2 out]
          }
          frame #1 {
            n211 = property on="X Scan" class="Bool (strict)"() -> ("Value"=w866:bool)  [unwired: 2 in, 2 out]
            n212 = Or(x=w865, y=w866) -> (x .or. y?=w867:bool)
            n213 = case shown="True" w867 {
              frame False {
                n214 = property on="X Go" class="Bool"("DisabledEnum"=T2."Enabled" ("Disabled")) -> ()  [unwired: 2 in, 2 out]
                n215 = property on="X Scan OK" class="Bool"("DisabledEnum"=T2."Enabled" ("Disabled")) -> ()  [unwired: 2 in, 2 out]
              }
              frame True {
                n216 = property on="X Go" class="Bool"("DisabledEnum"=T2."Disabled and Grayed Out" ("Disabled")) -> ()  [unwired: 2 in, 2 out]
                n217 = property on="X Scan OK" class="Bool"("DisabledEnum"=T2."Disabled and Grayed Out" ("Disabled")) -> ()  [unwired: 2 in, 2 out]
              }
            }
          }
          frame #2 {
            n218 = case shown="False" w876 {
              tunnel: w877 -> [w883 w887]
              tunnel: [w884 w887] -> w878
              tunnel: [w885 w886] -> w879
              tunnel: w880 -> [w882 w886]
              frame False {
                n219 = call "mDrive Send Command.vi"("error in (no error)"=w882, "Command"=T1."Stop", "VISA resource name"=w883) -> ("error out"=w885:errorcluster, "VISA resource name out"=w884:refnum<visa-resource-name>)  [unwired: 4 in, 1 out]
              }
              frame True {
              }
            }
          }
          frame #3 {
            n220 = property on="X Backlash corr" class="Bool (strict)"() -> ("Value"=w894:bool)  [unwired: 2 in, 2 out]
            n221 = Implies(1:w893, 2:w894) -> (0:w892:bool)
            n222 = case shown="False" w892 {
              tunnel: w891 -> [w901 w954]
              tunnel: w890 -> [w900 w955]
              tunnel: [w899 w954] -> w889
              tunnel: [w898 w955] -> w888
              frame False {
                # "Backlash"
                n223 = flat-sequence {
                  tunnel: [w916] -> w913
                  tunnel: [w918] -> w912
                  tunnel: [w917] -> w911
                  tunnel: w901 -> [w915]
                  tunnel: w900 -> [w914]
                  tunnel: w913 -> [w926]
                  tunnel: [w926] -> w910
                  tunnel: w912 -> [w925]
                  tunnel: w911 -> [w924]
                  tunnel: [w923] -> w909
                  tunnel: [w922] -> w908
                  tunnel: [w921] -> w897
                  tunnel: w910 -> [w936]
                  tunnel: w909 -> [w935]
                  tunnel: w908 -> [w933]
                  tunnel: [w934] -> w907
                  tunnel: [w933] -> w906
                  tunnel: [w932] -> w903
                  tunnel: [w931] -> w902
                  tunnel: w897 -> [w931]
                  tunnel: w907 -> [w947]
                  tunnel: w906 -> [w940]
                  tunnel: [w947] -> w905
                  tunnel: [w946] -> w904
                  tunnel: w903 -> [w946]
                  tunnel: w902 -> [w942]
                  tunnel: [w941] -> w895
                  tunnel: w905 -> [w951]
                  tunnel: w904 -> [w950]
                  tunnel: [w949] -> w899
                  tunnel: [w948] -> w896
                  tunnel: w895 -> [w948]
                  tunnel: [w953] -> w898
                  tunnel: w896 -> [w953]
                  frame #0 {
                    n224 = property on="X Backlash steps/sec" class="DigNum (strict)"() -> ("Value"=w916:i32)  [unwired: 2 in, 2 out]
                    n225 = Number To Decimal String(number=w916) -> (decimal integer string=w919:string)  [unwired: 1 in]
                    n226 = call "mDrive Send Command.vi"("error in (no error)"=w915, "Extra"=w919, "Command"=T1."Max Velocity", "VISA resource name"=w914) -> ("error out"=w917:errorcluster, "VISA resource name out"=w918:refnum<visa-resource-name>)  [unwired: 3 in, 1 out]
                  }
                  frame #1 {
                    n227 = property on="X Backlash" class="DigNum (strict)"() -> ("Value"=w921:i32)  [unwired: 2 in, 2 out]
                    n228 = Number To Decimal String(number=w921) -> (decimal integer string=w927:string)  [unwired: 1 in]
                    n229 = call "mDrive Send Command.vi"("error in (no error)"=w924, "Extra"=w927, "Command"=T1."Move to Relative Position", "VISA resource name"=w925) -> ("error out"=w923:errorcluster, "VISA resource name out"=w922:refnum<visa-resource-name>)  [unwired: 3 in, 1 out]
                  }
                  frame #2 {
                    n230 = To Double Precision Float(number=w931) -> (double precision float=w929:dbl)
                    n231 = To Double Precision Float(number=w936) -> (double precision float=w938:dbl)
                    n232 = Absolute Value(x=w929) -> (abs(x)=w930:dbl)
                    n233 = Divide(x=w930, y=w938) -> (x/y=w939:dbl)
                    n234 = Add(x=w939, y=0.3) -> (x+y=w932:dbl)
                    n235 = call "Time Delay13"("error in (no error)"=w935, "Delay Time (s)"=w932) -> ("error out"=w934:errorcluster)  [unwired: 9 in]
                  }
                  frame #3 {
                    n236 = Negate(x=w942) -> (-x=w943:i32)
                    n237 = Number To Decimal String(number=w943) -> (decimal integer string=w944:string)  [unwired: 1 in]
                    n238 = call "mDrive Send Command.vi"("Extra"=w944, "Command"=T1."Move to Relative Position", "VISA resource name"=w940) -> ("VISA resource name out"=w941:refnum<visa-resource-name>)  [unwired: 4 in, 2 out]
                  }
                  frame #4 {
                    n239 = call "Time Delay14"("error in (no error)"=w951, "Delay Time (s)"=w950) -> ("error out"=w949:errorcluster)  [unwired: 9 in]
                  }
                  frame #5 {
                    n240 = property on="X Backlash corr" class="Bool (strict)"("Val(Sgnl)"=FALSE ("Value (Signaling)")) -> ()  [unwired: 2 in, 2 out]
                  }
                }
              }
              frame True {
              }
            }
          }
        }
        n241 = flat-sequence {
          tunnel: w568 -> [w988]
          tunnel: w506 -> [w987]
          tunnel: [w993] -> w565
          tunnel: [w968] -> w563
          tunnel: [w980] -> w561
          tunnel: [w959] -> w559
          tunnel: w565 -> [w999]
          tunnel: [w999] -> w564
          tunnel: w563 -> [w998]
          tunnel: [w998] -> w562
          tunnel: w561 -> [w997]
          tunnel: [w997] -> w560
          tunnel: w559 -> [w994]
          tunnel: [w994] -> w555
          tunnel: w564 -> [w1006]
          tunnel: [w1007] -> w558
          tunnel: w562 -> [w1009]
          tunnel: [w1008] -> w557
          tunnel: w560 -> [w1005]
          tunnel: [w1004] -> w556
          tunnel: w555 -> [w1004]
          tunnel: w558 -> [w1019]
          tunnel: w557 -> [w1020]
          tunnel: w556 -> [w1022]
          tunnel: [w1018] -> w567
          tunnel: [w1017] -> w566
          frame #0 {
            w963 = 0.05 ("Delay Time (s)")
            n242 = property on="Y Step SP" class="DigNum (strict)"() -> ("Maximum"=w982:dbl)  [unwired: 2 in, 2 out]
            n243 = property on="Y Step SP" class="DigNum (strict)"() -> ("Minimum"=w984:dbl)  [unwired: 2 in, 2 out]
            n244 = property on="Y steps/rev" class="DigNum (strict)"() -> ("Value"=w978:u32)  [unwired: 2 in, 2 out]
            n245 = property on="Y offset mm" class="DigNum (strict)"() -> ("Value"=w974:dbl)  [unwired: 2 in, 2 out]
            n246 = To Long Integer(number=w982) -> (32bit integer=w981:i32)
            n247 = To Long Integer(number=w984) -> (32bit integer=w983:i32)
            n248 = To Double Precision Float(number=w978) -> (double precision float=w979:dbl)
            n249 = call "mDrive Send Command.vi"("error in (no error)"=w988, "Extra"="P", "Command"=T1."Print Parameter", "VISA resource name"=w987) -> ("error out"=w986:errorcluster, "read buffer"=w992:string, "VISA resource name out"=w990:refnum<visa-resource-name>)  [unwired: 3 in]
            n250 = call "Time Delay4"("error in (no error)"=w986, "Delay Time (s)"=w963) -> ("error out"=w985:errorcluster)  [unwired: 9 in]
            n251 = Decimal String To Number(string=w992, offset=0) -> (number=w970:i32)  [unwired: 1 in, 1 out]
            n252 = To Long Integer(number=w970) -> (32bit integer=w972:i32)
            n253 = property on="Y Step PV" class="DigNum (strict)"("Val(Sgnl)"=w972) -> ()  [unwired: 2 in, 2 out]
            n254 = call "mDrive Send Command.vi"("error in (no error)"=w985, "Extra"="MV", "Command"=T1."Print Parameter", "VISA resource name"=w990) -> ("error out"=w989:errorcluster, "read buffer"=w956:string, "VISA resource name out"=w993:refnum<visa-resource-name>)  [unwired: 3 in]
            n255 = call "Time Delay3"("error in (no error)"=w989, "Delay Time (s)"=w963) -> ("error out"=w968:errorcluster)  [unwired: 9 in]
            n256 = In Range and Coerce(upper limit=w981, x=w972, lower limit=w983) -> (In Range?=w980:bool)  [unwired: 1 out]
            n257 = To Double Precision Float(number=w972) -> (double precision float=w973:dbl)
            n258 = Decimal String To Number(string=w956, offset=0 ("offset (0)")) -> (number=w962:i32)  [unwired: 1 in, 1 out]
            n259 = Not Equal?(x=w956, y="") -> (x != y?=w957:bool)
            n260 = property on="Y in Range" class="Bool (strict)"("Val(Sgnl)"=w980) -> ()  [unwired: 2 in, 2 out]
            n261 = property on="Y Ready" class="Bool (strict)"("Val(Sgnl)"=w957) -> ()  [unwired: 2 in, 2 out]
            n262 = Divide(x=w973, y=w979) -> (x/y=w977:dbl)
            n263 = Number To Boolean Array(number=w962) -> (Boolean array=w961:bool[])
            n264 = property on="Y mm/rev" class="DigNum (strict)"() -> ("Value"=w976:dbl)  [unwired: 2 in, 2 out]
            n265 = Index Array(array=w961, index=0) -> (element=w959:bool)
            n266 = Multiply(x=w977, y=w976) -> (x*y=w975:dbl)
            n267 = property on="Y in Motion" class="Bool (strict)"("Val(Sgnl)"=w959) -> ()  [unwired: 2 in, 2 out]
            n268 = Add(x=w975, y=w974) -> (x+y=w971:dbl)
            n269 = property on="Y Position mm PV" class="DigNum (strict)"("Val(Sgnl)"=w971) -> ()  [unwired: 2 in, 2 out]
          }
          frame #1 {
            n270 = property on="Y Scan" class="Bool (strict)"() -> ("Value"=w995:bool)  [unwired: 2 in, 2 out]
            n271 = Or(x=w994, y=w995) -> (x .or. y?=w996:bool)
            n272 = case shown="True" w996 {
              frame False {
                n273 = property on="Y Go" class="Bool"("DisabledEnum"=T2."Enabled" ("Disabled")) -> ()  [unwired: 2 in, 2 out]
                n274 = property on="Y Scan OK" class="Bool"("DisabledEnum"=T2."Enabled" ("Disabled")) -> ()  [unwired: 2 in, 2 out]
              }
              frame True {
                n275 = property on="Y Go" class="Bool"("DisabledEnum"=T2."Disabled and Grayed Out" ("Disabled")) -> ()  [unwired: 2 in, 2 out]
                n276 = property on="Y Scan OK" class="Bool"("DisabledEnum"=T2."Disabled and Grayed Out" ("Disabled")) -> ()  [unwired: 2 in, 2 out]
              }
            }
          }
          frame #2 {
            n277 = case shown="False" w1005 {
              tunnel: w1006 -> [w1012 w1016]
              tunnel: [w1013 w1016] -> w1007
              tunnel: [w1014 w1015] -> w1008
              tunnel: w1009 -> [w1011 w1015]
              frame False {
                n278 = call "mDrive Send Command.vi"("error in (no error)"=w1011, "Command"=T1."Stop", "VISA resource name"=w1012) -> ("error out"=w1014:errorcluster, "VISA resource name out"=w1013:refnum<visa-resource-name>)  [unwired: 4 in, 1 out]
              }
              frame True {
              }
            }
          }
          frame #3 {
            n279 = property on="Y Backlash corr" class="Bool (strict)"() -> ("Value"=w1023:bool)  [unwired: 2 in, 2 out]
            n280 = Implies(1:w1022, 2:w1023) -> (0:w1021:bool)
            n281 = case shown="False" w1021 {
              tunnel: w1020 -> [w1030 w1083]
              tunnel: w1019 -> [w1029 w1084]
              tunnel: [w1028 w1083] -> w1018
              tunnel: [w1027 w1084] -> w1017
              frame False {
                # "Backlash"
                n282 = flat-sequence {
                  tunnel: [w1045] -> w1042
                  tunnel: [w1047] -> w1041
                  tunnel: [w1046] -> w1040
                  tunnel: w1030 -> [w1044]
                  tunnel: w1029 -> [w1043]
                  tunnel: w1042 -> [w1055]
                  tunnel: [w1055] -> w1039
                  tunnel: w1041 -> [w1054]
                  tunnel: w1040 -> [w1053]
                  tunnel: [w1052] -> w1038
                  tunnel: [w1051] -> w1037
                  tunnel: [w1050] -> w1026
                  tunnel: w1039 -> [w1065]
                  tunnel: w1038 -> [w1064]
                  tunnel: w1037 -> [w1062]
                  tunnel: [w1063] -> w1036
                  tunnel: [w1062] -> w1035
                  tunnel: [w1061] -> w1032
                  tunnel: [w1060] -> w1031
                  tunnel: w1026 -> [w1060]
                  tunnel: w1036 -> [w1076]
                  tunnel: w1035 -> [w1069]
                  tunnel: [w1076] -> w1034
                  tunnel: [w1075] -> w1033
                  tunnel: w1032 -> [w1075]
                  tunnel: w1031 -> [w1071]
                  tunnel: [w1070] -> w1024
                  tunnel: w1034 -> [w1080]
                  tunnel: w1033 -> [w1079]
                  tunnel: [w1078] -> w1028
                  tunnel: [w1077] -> w1025
                  tunnel: w1024 -> [w1077]
                  tunnel: [w1082] -> w1027
                  tunnel: w1025 -> [w1082]
                  frame #0 {
                    n283 = property on="Y Backlash steps/sec" class="DigNum (strict)"() -> ("Value"=w1045:i32)  [unwired: 2 in, 2 out]
                    n284 = Number To Decimal String(number=w1045) -> (decimal integer string=w1048:string)  [unwired: 1 in]
                    n285 = call "mDrive Send Command.vi"("error in (no error)"=w1044, "Extra"=w1048, "Command"=T1."Max Velocity", "VISA resource name"=w1043) -> ("error out"=w1046:errorcluster, "VISA resource name out"=w1047:refnum<visa-resource-name>)  [unwired: 3 in, 1 out]
                  }
                  frame #1 {
                    n286 = property on="Y Backlash" class="DigNum (strict)"() -> ("Value"=w1050:i32)  [unwired: 2 in, 2 out]
                    n287 = Number To Decimal String(number=w1050) -> (decimal integer string=w1056:string)  [unwired: 1 in]
                    n288 = call "mDrive Send Command.vi"("error in (no error)"=w1053, "Extra"=w1056, "Command"=T1."Move to Relative Position", "VISA resource name"=w1054) -> ("error out"=w1052:errorcluster, "VISA resource name out"=w1051:refnum<visa-resource-name>)  [unwired: 3 in, 1 out]
                  }
                  frame #2 {
                    n289 = To Double Precision Float(number=w1060) -> (double precision float=w1058:dbl)
                    n290 = To Double Precision Float(number=w1065) -> (double precision float=w1067:dbl)
                    n291 = Absolute Value(x=w1058) -> (abs(x)=w1059:dbl)
                    n292 = Divide(x=w1059, y=w1067) -> (x/y=w1068:dbl)
                    n293 = Add(x=w1068, y=0.3) -> (x+y=w1061:dbl)
                    n294 = call "Time Delay8"("error in (no error)"=w1064, "Delay Time (s)"=w1061) -> ("error out"=w1063:errorcluster)  [unwired: 9 in]
                  }
                  frame #3 {
                    n295 = Negate(x=w1071) -> (-x=w1072:i32)
                    n296 = Number To Decimal String(number=w1072) -> (decimal integer string=w1073:string)  [unwired: 1 in]
                    n297 = call "mDrive Send Command.vi"("Extra"=w1073, "Command"=T1."Move to Relative Position", "VISA resource name"=w1069) -> ("VISA resource name out"=w1070:refnum<visa-resource-name>)  [unwired: 4 in, 2 out]
                  }
                  frame #4 {
                    n298 = call "Time Delay2"("error in (no error)"=w1080, "Delay Time (s)"=w1079) -> ("error out"=w1078:errorcluster)  [unwired: 9 in]
                  }
                  frame #5 {
                    n299 = property on="Y Backlash corr" class="Bool (strict)"("Val(Sgnl)"=FALSE ("Value (Signaling)")) -> ()  [unwired: 2 in, 2 out]
                  }
                }
              }
              frame True {
              }
            }
          }
        }
        n300 = flat-sequence {
          tunnel: [w735] -> w540
          tunnel: [w712] -> w539
          tunnel: [w724] -> w538
          tunnel: [w703] -> w537
          tunnel: w515 -> [w702]
          tunnel: w518 -> [w701]
          tunnel: w540 -> [w741]
          tunnel: [w741] -> w536
          tunnel: w539 -> [w740]
          tunnel: [w740] -> w535
          tunnel: w538 -> [w739]
          tunnel: [w739] -> w534
          tunnel: w537 -> [w736]
          tunnel: [w736] -> w533
          tunnel: w536 -> [w748]
          tunnel: [w749] -> w532
          tunnel: w535 -> [w751]
          tunnel: [w750] -> w531
          tunnel: w534 -> [w747]
          tunnel: [w746] -> w530
          tunnel: w533 -> [w746]
          tunnel: w532 -> [w761]
          tunnel: w531 -> [w762]
          tunnel: w530 -> [w764]
          tunnel: [w760] -> w516
          tunnel: [w759] -> w517
          frame #0 {
            w707 = 0.05 ("Delay Time (s)")
            n301 = property on="Z Step SP" class="DigNum (strict)"() -> ("Maximum"=w726:dbl)  [unwired: 2 in, 2 out]
            n302 = property on="Z Step SP" class="DigNum (strict)"() -> ("Minimum"=w728:dbl)  [unwired: 2 in, 2 out]
            n303 = property on="Z steps/rev" class="DigNum (strict)"() -> ("Value"=w722:u32)  [unwired: 2 in, 2 out]
            n304 = property on="Z offset mm" class="DigNum (strict)"() -> ("Value"=w718:dbl)  [unwired: 2 in, 2 out]
            n305 = To Long Integer(number=w726) -> (32bit integer=w725:i32)
            n306 = To Long Integer(number=w728) -> (32bit integer=w727:i32)
            n307 = To Double Precision Float(number=w722) -> (double precision float=w723:dbl)
            n308 = call "mDrive Send Command.vi"("error in (no error)"=w701, "Extra"="P", "Command"=T1."Print Parameter", "VISA resource name"=w702) -> ("error out"=w730:errorcluster, "read buffer"=w734:string, "VISA resource name out"=w732:refnum<visa-resource-name>)  [unwired: 3 in]
            n309 = call "Time Delay17"("error in (no error)"=w730, "Delay Time (s)"=w707) -> ("error out"=w729:errorcluster)  [unwired: 9 in]
            n310 = Decimal String To Number(string=w734, offset=0) -> (number=w714:i32)  [unwired: 1 in, 1 out]
            n311 = To Long Integer(number=w714) -> (32bit integer=w716:i32)
            n312 = property on="Z Step PV" class="DigNum (strict)"("Val(Sgnl)"=w716) -> ()  [unwired: 2 in, 2 out]
            n313 = call "mDrive Send Command.vi"("error in (no error)"=w729, "Extra"="MV", "Command"=T1."Print Parameter", "VISA resource name"=w732) -> ("error out"=w731:errorcluster, "read buffer"=w698:string, "VISA resource name out"=w735:refnum<visa-resource-name>)  [unwired: 3 in]
            n314 = call "Time Delay16"("error in (no error)"=w731, "Delay Time (s)"=w707) -> ("error out"=w712:errorcluster)  [unwired: 9 in]
            n315 = In Range and Coerce(upper limit=w725, x=w716, lower limit=w727) -> (In Range?=w724:bool)  [unwired: 1 out]
            n316 = To Double Precision Float(number=w716) -> (double precision float=w717:dbl)
            n317 = Decimal String To Number(string=w698, offset=0 ("offset (0)")) -> (number=w706:i32)  [unwired: 1 in, 1 out]
            n318 = Not Equal?(x=w698, y="") -> (x != y?=w699:bool)
            n319 = property on="Z in Range" class="Bool (strict)"("Val(Sgnl)"=w724) -> ()  [unwired: 2 in, 2 out]
            n320 = property on="Z Ready" class="Bool (strict)"("Val(Sgnl)"=w699) -> ()  [unwired: 2 in, 2 out]
            n321 = Divide(x=w717, y=w723) -> (x/y=w721:dbl)
            n322 = Number To Boolean Array(number=w706) -> (Boolean array=w705:bool[])
            n323 = property on="Z mm/rev" class="DigNum (strict)"() -> ("Value"=w720:dbl)  [unwired: 2 in, 2 out]
            n324 = Index Array(array=w705, index=0) -> (element=w703:bool)
            n325 = Multiply(x=w721, y=w720) -> (x*y=w719:dbl)
            n326 = property on="Z in Motion" class="Bool (strict)"("Val(Sgnl)"=w703) -> ()  [unwired: 2 in, 2 out]
            n327 = Add(x=w719, y=w718) -> (x+y=w715:dbl)
            n328 = property on="Z Position mm PV" class="DigNum (strict)"("Val(Sgnl)"=w715) -> ()  [unwired: 2 in, 2 out]
          }
          frame #1 {
            n329 = property on="Z Scan" class="Bool (strict)"() -> ("Value"=w737:bool)  [unwired: 2 in, 2 out]
            n330 = Or(x=w736, y=w737) -> (x .or. y?=w738:bool)
            n331 = case shown="True" w738 {
              frame False {
                n332 = property on="Z Go" class="Bool"("DisabledEnum"=T2."Enabled" ("Disabled")) -> ()  [unwired: 2 in, 2 out]
                n333 = property on="Z Scan OK" class="Bool"("DisabledEnum"=T2."Enabled" ("Disabled")) -> ()  [unwired: 2 in, 2 out]
              }
              frame True {
                n334 = property on="Z Go" class="Bool"("DisabledEnum"=T2."Disabled and Grayed Out" ("Disabled")) -> ()  [unwired: 2 in, 2 out]
                n335 = property on="Z Scan OK" class="Bool"("DisabledEnum"=T2."Disabled and Grayed Out" ("Disabled")) -> ()  [unwired: 2 in, 2 out]
              }
            }
          }
          frame #2 {
            n336 = case shown="False" w747 {
              tunnel: w748 -> [w754 w758]
              tunnel: [w755 w758] -> w749
              tunnel: [w756 w757] -> w750
              tunnel: w751 -> [w753 w757]
              frame False {
                n337 = call "mDrive Send Command.vi"("error in (no error)"=w753, "Command"=T1."Stop", "VISA resource name"=w754) -> ("error out"=w756:errorcluster, "VISA resource name out"=w755:refnum<visa-resource-name>)  [unwired: 4 in, 1 out]
              }
              frame True {
              }
            }
          }
          frame #3 {
            n338 = property on="Z Backlash corr" class="Bool (strict)"() -> ("Value"=w765:bool)  [unwired: 2 in, 2 out]
            n339 = Implies(1:w764, 2:w765) -> (0:w763:bool)
            n340 = case shown="False" w763 {
              tunnel: w762 -> [w772 w825]
              tunnel: w761 -> [w771 w826]
              tunnel: [w770 w825] -> w760
              tunnel: [w769 w826] -> w759
              frame False {
                # "Backlash"
                n341 = flat-sequence {
                  tunnel: [w787] -> w784
                  tunnel: [w789] -> w783
                  tunnel: [w788] -> w782
                  tunnel: w772 -> [w786]
                  tunnel: w771 -> [w785]
                  tunnel: w784 -> [w797]
                  tunnel: [w797] -> w781
                  tunnel: w783 -> [w796]
                  tunnel: w782 -> [w795]
                  tunnel: [w794] -> w780
                  tunnel: [w793] -> w779
                  tunnel: [w792] -> w768
                  tunnel: w781 -> [w807]
                  tunnel: w780 -> [w806]
                  tunnel: w779 -> [w804]
                  tunnel: [w805] -> w778
                  tunnel: [w804] -> w777
                  tunnel: [w803] -> w774
                  tunnel: [w802] -> w773
                  tunnel: w768 -> [w802]
                  tunnel: w778 -> [w818]
                  tunnel: w777 -> [w811]
                  tunnel: [w818] -> w776
                  tunnel: [w817] -> w775
                  tunnel: w774 -> [w817]
                  tunnel: w773 -> [w813]
                  tunnel: [w812] -> w766
                  tunnel: w776 -> [w822]
                  tunnel: w775 -> [w821]
                  tunnel: [w820] -> w770
                  tunnel: [w819] -> w767
                  tunnel: w766 -> [w819]
                  tunnel: [w824] -> w769
                  tunnel: w767 -> [w824]
                  frame #0 {
                    n342 = property on="Z Backlash steps/sec" class="DigNum (strict)"() -> ("Value"=w787:i32)  [unwired: 2 in, 2 out]
                    n343 = Number To Decimal String(number=w787) -> (decimal integer string=w790:string)  [unwired: 1 in]
                    n344 = call "mDrive Send Command.vi"("error in (no error)"=w786, "Extra"=w790, "Command"=T1."Max Velocity", "VISA resource name"=w785) -> ("error out"=w788:errorcluster, "VISA resource name out"=w789:refnum<visa-resource-name>)  [unwired: 3 in, 1 out]
                  }
                  frame #1 {
                    n345 = property on="Z Backlash" class="DigNum (strict)"() -> ("Value"=w792:i32)  [unwired: 2 in, 2 out]
                    n346 = Number To Decimal String(number=w792) -> (decimal integer string=w798:string)  [unwired: 1 in]
                    n347 = call "mDrive Send Command.vi"("error in (no error)"=w795, "Extra"=w798, "Command"=T1."Move to Relative Position", "VISA resource name"=w796) -> ("error out"=w794:errorcluster, "VISA resource name out"=w793:refnum<visa-resource-name>)  [unwired: 3 in, 1 out]
                  }
                  frame #2 {
                    n348 = To Double Precision Float(number=w802) -> (double precision float=w800:dbl)
                    n349 = To Double Precision Float(number=w807) -> (double precision float=w809:dbl)
                    n350 = Absolute Value(x=w800) -> (abs(x)=w801:dbl)
                    n351 = Divide(x=w801, y=w809) -> (x/y=w810:dbl)
                    n352 = Add(x=w810, y=0.5) -> (x+y=w803:dbl)
                    n353 = call "Time Delay18"("error in (no error)"=w806, "Delay Time (s)"=w803) -> ("error out"=w805:errorcluster)  [unwired: 9 in]
                  }
                  frame #3 {
                    n354 = Negate(x=w813) -> (-x=w814:i32)
                    n355 = Number To Decimal String(number=w814) -> (decimal integer string=w815:string)  [unwired: 1 in]
                    n356 = call "mDrive Send Command.vi"("Extra"=w815, "Command"=T1."Move to Relative Position", "VISA resource name"=w811) -> ("VISA resource name out"=w812:refnum<visa-resource-name>)  [unwired: 4 in, 2 out]
                  }
                  frame #4 {
                    n357 = call "Time Delay19"("error in (no error)"=w822, "Delay Time (s)"=w821) -> ("error out"=w820:errorcluster)  [unwired: 9 in]
                  }
                  frame #5 {
                    n358 = property on="Z Backlash corr" class="Bool (strict)"("Val(Sgnl)"=FALSE ("Value (Signaling)")) -> ()  [unwired: 2 in, 2 out]
                  }
                }
              }
              frame True {
              }
            }
          }
        }
        n359 = flat-sequence {
          tunnel: [w606] -> w529
          tunnel: [w583] -> w528
          tunnel: [w595] -> w527
          tunnel: [w574] -> w526
          tunnel: w514 -> [w573]
          tunnel: w513 -> [w572]
          tunnel: w529 -> [w612]
          tunnel: [w612] -> w525
          tunnel: w528 -> [w611]
          tunnel: [w611] -> w524
          tunnel: w527 -> [w610]
          tunnel: [w610] -> w523
          tunnel: w526 -> [w607]
          tunnel: [w607] -> w522
          tunnel: w525 -> [w619]
          tunnel: [w620] -> w521
          tunnel: w524 -> [w622]
          tunnel: [w621] -> w520
          tunnel: w523 -> [w618]
          tunnel: [w617] -> w519
          tunnel: w522 -> [w617]
          tunnel: w521 -> [w632]
          tunnel: w520 -> [w633]
          tunnel: w519 -> [w635]
          tunnel: [w631] -> w511
          tunnel: [w630] -> w512
          frame #0 {
            w578 = 0.05 ("Delay Time (s)")
            n360 = property on="R Step SP" class="DigNum (strict)"() -> ("Maximum"=w597:dbl)  [unwired: 2 in, 2 out]
            n361 = property on="R Step SP" class="DigNum (strict)"() -> ("Minimum"=w599:dbl)  [unwired: 2 in, 2 out]
            n362 = property on="R steps/rev" class="DigNum (strict)"() -> ("Value"=w593:u32)  [unwired: 2 in, 2 out]
            n363 = property on="R offset deg" class="DigNum (strict)"() -> ("Value"=w589:dbl)  [unwired: 2 in, 2 out]
            n364 = To Long Integer(number=w597) -> (32bit integer=w596:i32)
            n365 = To Long Integer(number=w599) -> (32bit integer=w598:i32)
            n366 = To Double Precision Float(number=w593) -> (double precision float=w594:dbl)
            n367 = call "mDrive Send Command.vi"("error in (no error)"=w572, "Extra"="P", "Command"=T1."Print Parameter", "VISA resource name"=w573) -> ("error out"=w601:errorcluster, "read buffer"=w605:string, "VISA resource name out"=w603:refnum<visa-resource-name>)  [unwired: 3 in]
            n368 = call "Time Delay21"("error in (no error)"=w601, "Delay Time (s)"=w578) -> ("error out"=w600:errorcluster)  [unwired: 9 in]
            n369 = Decimal String To Number(string=w605, offset=0) -> (number=w585:i32)  [unwired: 1 in, 1 out]
            n370 = To Long Integer(number=w585) -> (32bit integer=w587:i32)
            n371 = property on="R Step PV" class="DigNum (strict)"("Val(Sgnl)"=w587) -> ()  [unwired: 2 in, 2 out]
            n372 = call "mDrive Send Command.vi"("error in (no error)"=w600, "Extra"="MV", "Command"=T1."Print Parameter", "VISA resource name"=w603) -> ("error out"=w602:errorcluster, "read buffer"=w569:string, "VISA resource name out"=w606:refnum<visa-resource-name>)  [unwired: 3 in]
            n373 = call "Time Delay20"("error in (no error)"=w602, "Delay Time (s)"=w578) -> ("error out"=w583:errorcluster)  [unwired: 9 in]
            n374 = In Range and Coerce(upper limit=w596, x=w587, lower limit=w598) -> (In Range?=w595:bool)  [unwired: 1 out]
            n375 = To Double Precision Float(number=w587) -> (double precision float=w588:dbl)
            n376 = Decimal String To Number(string=w569, offset=0 ("offset (0)")) -> (number=w577:i32)  [unwired: 1 in, 1 out]
            n377 = Not Equal?(x=w569, y="") -> (x != y?=w570:bool)
            n378 = property on="R in Range" class="Bool (strict)"("Val(Sgnl)"=w595) -> ()  [unwired: 2 in, 2 out]
            n379 = property on="R Ready" class="Bool (strict)"("Val(Sgnl)"=w570) -> ()  [unwired: 2 in, 2 out]
            n380 = Divide(x=w588, y=w594) -> (x/y=w592:dbl)
            n381 = Number To Boolean Array(number=w577) -> (Boolean array=w576:bool[])
            n382 = property on="R deg/rev" class="DigNum (strict)"() -> ("Value"=w591:dbl)  [unwired: 2 in, 2 out]
            n383 = Index Array(array=w576, index=0) -> (element=w574:bool)
            n384 = Multiply(x=w592, y=w591) -> (x*y=w590:dbl)
            n385 = property on="R in Motion" class="Bool (strict)"("Val(Sgnl)"=w574) -> ()  [unwired: 2 in, 2 out]
            n386 = Add(x=w590, y=w589) -> (x+y=w586:dbl)
            n387 = property on="R Position deg PV" class="DigNum (strict)"("Val(Sgnl)"=w586) -> ()  [unwired: 2 in, 2 out]
          }
          frame #1 {
            n388 = property on="R Scan" class="Bool (strict)"() -> ("Value"=w608:bool)  [unwired: 2 in, 2 out]
            n389 = Or(x=w607, y=w608) -> (x .or. y?=w609:bool)
            n390 = case shown="True" w609 {
              frame False {
                n391 = property on="R Go" class="Bool"("DisabledEnum"=T2."Enabled" ("Disabled")) -> ()  [unwired: 2 in, 2 out]
                n392 = property on="R Scan OK" class="Bool"("DisabledEnum"=T2."Enabled" ("Disabled")) -> ()  [unwired: 2 in, 2 out]
              }
              frame True {
                n393 = property on="R Go" class="Bool"("DisabledEnum"=T2."Disabled and Grayed Out" ("Disabled")) -> ()  [unwired: 2 in, 2 out]
                n394 = property on="R Scan OK" class="Bool"("DisabledEnum"=T2."Disabled and Grayed Out" ("Disabled")) -> ()  [unwired: 2 in, 2 out]
              }
            }
          }
          frame #2 {
            n395 = case shown="False" w618 {
              tunnel: w619 -> [w625 w629]
              tunnel: [w626 w629] -> w620
              tunnel: [w627 w628] -> w621
              tunnel: w622 -> [w624 w628]
              frame False {
                n396 = call "mDrive Send Command.vi"("error in (no error)"=w624, "Command"=T1."Stop", "VISA resource name"=w625) -> ("error out"=w627:errorcluster, "VISA resource name out"=w626:refnum<visa-resource-name>)  [unwired: 4 in, 1 out]
              }
              frame True {
              }
            }
          }
          frame #3 {
            n397 = property on="R Backlash corr" class="Bool (strict)"() -> ("Value"=w636:bool)  [unwired: 2 in, 2 out]
            n398 = Implies(1:w635, 2:w636) -> (0:w634:bool)
            n399 = case shown="False" w634 {
              tunnel: w633 -> [w643 w696]
              tunnel: w632 -> [w642 w697]
              tunnel: [w641 w696] -> w631
              tunnel: [w640 w697] -> w630
              frame False {
                # "Backlash"
                n400 = flat-sequence {
                  tunnel: [w658] -> w655
                  tunnel: [w660] -> w654
                  tunnel: [w659] -> w653
                  tunnel: w643 -> [w657]
                  tunnel: w642 -> [w656]
                  tunnel: w655 -> [w668]
                  tunnel: [w668] -> w652
                  tunnel: w654 -> [w667]
                  tunnel: w653 -> [w666]
                  tunnel: [w665] -> w651
                  tunnel: [w664] -> w650
                  tunnel: [w663] -> w639
                  tunnel: w652 -> [w678]
                  tunnel: w651 -> [w677]
                  tunnel: w650 -> [w675]
                  tunnel: [w676] -> w649
                  tunnel: [w675] -> w648
                  tunnel: [w674] -> w645
                  tunnel: [w673] -> w644
                  tunnel: w639 -> [w673]
                  tunnel: w649 -> [w689]
                  tunnel: w648 -> [w682]
                  tunnel: [w689] -> w647
                  tunnel: [w688] -> w646
                  tunnel: w645 -> [w688]
                  tunnel: w644 -> [w684]
                  tunnel: [w683] -> w637
                  tunnel: w647 -> [w693]
                  tunnel: w646 -> [w692]
                  tunnel: [w691] -> w641
                  tunnel: [w690] -> w638
                  tunnel: w637 -> [w690]
                  tunnel: [w695] -> w640
                  tunnel: w638 -> [w695]
                  frame #0 {
                    n401 = property on="R Backlash steps/sec" class="DigNum (strict)"() -> ("Value"=w658:i32)  [unwired: 2 in, 2 out]
                    n402 = Number To Decimal String(number=w658) -> (decimal integer string=w661:string)  [unwired: 1 in]
                    n403 = call "mDrive Send Command.vi"("error in (no error)"=w657, "Extra"=w661, "Command"=T1."Max Velocity", "VISA resource name"=w656) -> ("error out"=w659:errorcluster, "VISA resource name out"=w660:refnum<visa-resource-name>)  [unwired: 3 in, 1 out]
                  }
                  frame #1 {
                    n404 = property on="R Backlash" class="DigNum (strict)"() -> ("Value"=w663:i32)  [unwired: 2 in, 2 out]
                    n405 = Number To Decimal String(number=w663) -> (decimal integer string=w669:string)  [unwired: 1 in]
                    n406 = call "mDrive Send Command.vi"("error in (no error)"=w666, "Extra"=w669, "Command"=T1."Move to Relative Position", "VISA resource name"=w667) -> ("error out"=w665:errorcluster, "VISA resource name out"=w664:refnum<visa-resource-name>)  [unwired: 3 in, 1 out]
                  }
                  frame #2 {
                    n407 = To Double Precision Float(number=w673) -> (double precision float=w671:dbl)
                    n408 = To Double Precision Float(number=w678) -> (double precision float=w680:dbl)
                    n409 = Absolute Value(x=w671) -> (abs(x)=w672:dbl)
                    n410 = Divide(x=w672, y=w680) -> (x/y=w681:dbl)
                    n411 = Add(x=w681, y=0.3) -> (x+y=w674:dbl)
                    n412 = call "Time Delay22"("error in (no error)"=w677, "Delay Time (s)"=w674) -> ("error out"=w676:errorcluster)  [unwired: 9 in]
                  }
                  frame #3 {
                    n413 = Negate(x=w684) -> (-x=w685:i32)
                    n414 = Number To Decimal String(number=w685) -> (decimal integer string=w686:string)  [unwired: 1 in]
                    n415 = call "mDrive Send Command.vi"("Extra"=w686, "Command"=T1."Move to Relative Position", "VISA resource name"=w682) -> ("VISA resource name out"=w683:refnum<visa-resource-name>)  [unwired: 4 in, 2 out]
                  }
                  frame #4 {
                    n416 = call "Time Delay23"("error in (no error)"=w693, "Delay Time (s)"=w692) -> ("error out"=w691:errorcluster)  [unwired: 9 in]
                  }
                  frame #5 {
                    n417 = property on="R Backlash corr" class="Bool (strict)"("Val(Sgnl)"=FALSE ("Value (Signaling)")) -> ()  [unwired: 2 in, 2 out]
                  }
                }
              }
              frame True {
              }
            }
          }
        }
        n418 = property on="X Position mm PV" class="DigNum (strict)"() -> ("Value"=w507:dbl)  [unwired: 2 in, 2 out]
        n419 = property on="Y Position mm PV" class="DigNum (strict)"() -> ("Value"=w500:dbl)  [unwired: 2 in, 2 out]
        n420 = property on="Z Position mm PV" class="DigNum (strict)"() -> ("Value"=w501:dbl)  [unwired: 2 in, 2 out]
        n421 = property on="R Position deg PV" class="DigNum (strict)"() -> ("Value"=w508:dbl)  [unwired: 2 in, 2 out]
        n422 = property on="Y Scan Length SP steps" class="DigNum (strict)"() -> ("Value"=w492:i32)  [unwired: 2 in, 2 out]
        n423 = property on="Z Scan Length SP steps" class="DigNum (strict)"() -> ("Value"=w493:i32)  [unwired: 2 in, 2 out]
        n424 = Divide(x=w492, y=w493) -> (x/y=w494:dbl)
        n425 = call "Build XY Graph"("Reset"=TRUE, "Y Input"=w500, "X Input"=w507) -> ("XY Graph"=→"XY Graph":cluster{"Y":dbl[], "Y":dbl[]}[])  [unwired: 7 in, 1 out]
        n426 = call "Build XY Graph2"("Reset"=TRUE, "Y Input"=w508, "X Input"=w501) -> ("XY Graph"=→"ZR Graph":cluster{"Y":dbl[], "Y":dbl[]}[])  [unwired: 7 in, 1 out]
        n427 = property on="Clear ZY" class="Bool (strict)"() -> ("Value"=w491:bool)  [unwired: 2 in, 2 out]
        n428 = call "Build XY Graph3"("Reset"=w491, "Y Input"=w500, "X Input"=w501) -> ("XY Graph"=→"ZY Graph":cluster{"Y":dbl[], "Y":dbl[]}[])  [unwired: 7 in, 1 out]
        n429 = Inverse Tangent(1:w494) -> (0:w495:dbl)
        n430 = Divide(x=w495, y=6.283185307179586) -> (x/y=w496:dbl)
        n431 = Multiply(x=360.0, y=w496) -> (x*y=w499:dbl)
        n432 = property on="atan Y/Z" class="DigNum (strict)"("Val(Sgnl)"=w499) -> ()  [unwired: 2 in, 2 out]
      }
      event "Reset Y Position mm", "Reset X Position mm", "Reset Z Position mm", "Reset R Position deg": Value Change {
        n433 = event-data() -> ()  [unwired: 1 in, 5 out]
        n434 = property on="Z steps/rev" class="DigNum (strict)"() -> ("Value"=w1096:u32)  [unwired: 2 in, 2 out]
        n435 = property on="R steps/rev" class="DigNum (strict)"() -> ("Value"=w1087:u32)  [unwired: 2 in, 2 out]
        n436 = property on="X steps/rev" class="DigNum (strict)"() -> ("Value"=w1105:u32)  [unwired: 2 in, 2 out]
        n437 = property on="Y steps/rev" class="DigNum (strict)"() -> ("Value"=w1114:u32)  [unwired: 2 in, 2 out]
        n438 = property on="Z offset mm" class="DigNum (strict)"() -> ("Value"=w1094:dbl)  [unwired: 2 in, 2 out]
        n439 = property on="R offset deg" class="DigNum (strict)"() -> ("Value"=w1085:dbl)  [unwired: 2 in, 2 out]
        n440 = property on="X offset mm" class="DigNum (strict)"() -> ("Value"=w1103:dbl)  [unwired: 2 in, 2 out]
        n441 = property on="Y offset mm" class="DigNum (strict)"() -> ("Value"=w1112:dbl)  [unwired: 2 in, 2 out]
        n442 = property on="Reset R Position deg" class="DigNum (strict)"() -> ("Value"=w1093:dbl)  [unwired: 2 in, 2 out]
        n443 = property on="Reset Z Position mm" class="DigNum (strict)"() -> ("Value"=w1102:dbl)  [unwired: 2 in, 2 out]
        n444 = property on="Reset X Position mm" class="DigNum (strict)"() -> ("Value"=w1111:dbl)  [unwired: 2 in, 2 out]
        n445 = property on="Reset Y Position mm" class="DigNum (strict)"() -> ("Value"=w1120:dbl)  [unwired: 2 in, 2 out]
        n446 = To Double Precision Float(number=w1087) -> (double precision float=w1090:dbl)
        n447 = To Double Precision Float(number=w1105) -> (double precision float=w1108:dbl)
        n448 = To Double Precision Float(number=w1114) -> (double precision float=w1117:dbl)
        n449 = Subtract(x=w1102, y=w1094) -> (x-y=w1101:dbl)
        n450 = Subtract(x=w1093, y=w1085) -> (x-y=w1092:dbl)
        n451 = Subtract(x=w1111, y=w1103) -> (x-y=w1110:dbl)
        n452 = Subtract(x=w1120, y=w1112) -> (x-y=w1119:dbl)
        n453 = property on="R deg/rev" class="DigNum (strict)"() -> ("Value"=w1086:dbl)  [unwired: 2 in, 2 out]
        n454 = property on="Z mm/rev" class="DigNum (strict)"() -> ("Value"=w1095:dbl)  [unwired: 2 in, 2 out]
        n455 = property on="X mm/rev" class="DigNum (strict)"() -> ("Value"=w1104:dbl)  [unwired: 2 in, 2 out]
        n456 = property on="Y mm/rev" class="DigNum (strict)"() -> ("Value"=w1113:dbl)  [unwired: 2 in, 2 out]
        n457 = Divide(x=w1092, y=w1086) -> (x/y=w1091:dbl)
        n458 = Divide(x=w1110, y=w1104) -> (x/y=w1109:dbl)
        n459 = Divide(x=w1119, y=w1113) -> (x/y=w1118:dbl)
        n460 = Divide(x=w1101, y=w1095) -> (x/y=w1100:dbl)
        n461 = To Double Precision Float(number=w1096) -> (double precision float=w1099:dbl)
        n462 = Multiply(x=w1100, y=w1099) -> (x*y=w1098:dbl)
        n463 = Multiply(x=w1091, y=w1090) -> (x*y=w1089:dbl)
        n464 = Multiply(x=w1109, y=w1108) -> (x*y=w1107:dbl)
        n465 = Multiply(x=w1118, y=w1117) -> (x*y=w1116:dbl)
        n466 = To Long Integer(number=w1098) -> (32bit integer=w1097:i32)
        n467 = To Long Integer(number=w1089) -> (32bit integer=w1088:i32)
        n468 = To Long Integer(number=w1107) -> (32bit integer=w1106:i32)
        n469 = To Long Integer(number=w1116) -> (32bit integer=w1115:i32)
        n470 = property on="Reset Z Motor Steps" class="DigNum (strict)"("Val(Sgnl)"=w1097) -> ()  [unwired: 2 in, 2 out]
        n471 = property on="Reset R Motor Steps" class="DigNum (strict)"("Val(Sgnl)"=w1088) -> ()  [unwired: 2 in, 2 out]
        n472 = property on="Reset X Motor Steps" class="DigNum (strict)"("Val(Sgnl)"=w1106) -> ()  [unwired: 2 in, 2 out]
        n473 = property on="Reset Y Motor Steps" class="DigNum (strict)"("Val(Sgnl)"=w1115) -> ()  [unwired: 2 in, 2 out]
      }
      event "Y Velocity SP step/sec", "X Velocity SP step/sec", "R Velocity SP step/sec", "Z Velocity SP step/sec", "Y Step SP", "X Step SP", "Z Step SP", "R Step SP": Value Change {
        n474 = event-data() -> ()  [unwired: 1 in, 5 out]
        n475 = property on="Y Step SP" class="DigNum (strict)"() -> ("Value"=w1153:i32)  [unwired: 2 in, 2 out]
        n476 = property on="X Step SP" class="DigNum (strict)"() -> ("Value"=w1145:i32)  [unwired: 2 in, 2 out]
        n477 = property on="Z Step SP" class="DigNum (strict)"() -> ("Value"=w1137:i32)  [unwired: 2 in, 2 out]
        n478 = property on="R Step SP" class="DigNum (strict)"() -> ("Value"=w1129:i32)  [unwired: 2 in, 2 out]
        n479 = property on="Y steps/rev" class="DigNum (strict)"() -> ("Value"=w1176:u32)  [unwired: 2 in, 2 out]
        n480 = property on="Y steps/rev" class="DigNum (strict)"() -> ("Value"=w1151:u32)  [unwired: 2 in, 2 out]
        n481 = property on="X steps/rev" class="DigNum (strict)"() -> ("Value"=w1170:u32)  [unwired: 2 in, 2 out]
        n482 = property on="X steps/rev" class="DigNum (strict)"() -> ("Value"=w1143:u32)  [unwired: 2 in, 2 out]
        n483 = property on="Z steps/rev" class="DigNum (strict)"() -> ("Value"=w1164:u32)  [unwired: 2 in, 2 out]
        n484 = property on="Z steps/rev" class="DigNum (strict)"() -> ("Value"=w1135:u32)  [unwired: 2 in, 2 out]
        n485 = property on="R steps/rev" class="DigNum (strict)"() -> ("Value"=w1158:u32)  [unwired: 2 in, 2 out]
        n486 = property on="R steps/rev" class="DigNum (strict)"() -> ("Value"=w1127:u32)  [unwired: 2 in, 2 out]
        n487 = property on="Y offset mm" class="DigNum (strict)"() -> ("Value"=w1150:dbl)  [unwired: 2 in, 2 out]
        n488 = property on="X offset mm" class="DigNum (strict)"() -> ("Value"=w1142:dbl)  [unwired: 2 in, 2 out]
        n489 = property on="Z offset mm" class="DigNum (strict)"() -> ("Value"=w1134:dbl)  [unwired: 2 in, 2 out]
        n490 = property on="R offset deg" class="DigNum (strict)"() -> ("Value"=w1126:dbl)  [unwired: 2 in, 2 out]
        n491 = property on="Y Velocity SP step/sec" class="DigNum (strict)"() -> ("Value"=w1178:i32)  [unwired: 2 in, 2 out]
        n492 = property on="X Velocity SP step/sec" class="DigNum (strict)"() -> ("Value"=w1172:i32)  [unwired: 2 in, 2 out]
        n493 = property on="Z Velocity SP step/sec" class="DigNum (strict)"() -> ("Value"=w1166:i32)  [unwired: 2 in, 2 out]
        n494 = property on="R Velocity SP step/sec" class="DigNum (strict)"() -> ("Value"=w1160:i32)  [unwired: 2 in, 2 out]
        n495 = To Double Precision Float(number=w1153) -> (double precision float=w1154:dbl)
        n496 = To Double Precision Float(number=w1151) -> (double precision float=w1157:dbl)
        n497 = To Double Precision Float(number=w1170) -> (double precision float=w1175:dbl)
        n498 = To Double Precision Float(number=w1145) -> (double precision float=w1146:dbl)
        n499 = To Double Precision Float(number=w1143) -> (double precision float=w1149:dbl)
        n500 = To Double Precision Float(number=w1164) -> (double precision float=w1169:dbl)
        n501 = To Double Precision Float(number=w1137) -> (double precision float=w1138:dbl)
        n502 = To Double Precision Float(number=w1135) -> (double precision float=w1141:dbl)
        n503 = To Double Precision Float(number=w1158) -> (double precision float=w1163:dbl)
        n504 = To Double Precision Float(number=w1129) -> (double precision float=w1130:dbl)
        n505 = To Double Precision Float(number=w1127) -> (double precision float=w1133:dbl)
        n506 = Divide(x=w1130, y=w1133) -> (x/y=w1132:dbl)
        n507 = Divide(x=w1154, y=w1157) -> (x/y=w1156:dbl)
        n508 = Divide(x=w1146, y=w1149) -> (x/y=w1148:dbl)
        n509 = Divide(x=w1138, y=w1141) -> (x/y=w1140:dbl)
        n510 = To Double Precision Float(number=w1160) -> (double precision float=w1161:dbl)
        n511 = To Double Precision Float(number=w1178) -> (double precision float=w1179:dbl)
        n512 = To Double Precision Float(number=w1176) -> (double precision float=w1181:dbl)
        n513 = To Double Precision Float(number=w1172) -> (double precision float=w1173:dbl)
        n514 = To Double Precision Float(number=w1166) -> (double precision float=w1167:dbl)
        n515 = property on="R deg/rev" class="DigNum (strict)"() -> ("Value"=w1125:dbl)  [unwired: 2 in, 2 out]
        n516 = property on="Y mm/rev" class="DigNum (strict)"() -> ("Value"=w1122:dbl)  [unwired: 2 in, 2 out]
        n517 = property on="X mm/rev" class="DigNum (strict)"() -> ("Value"=w1123:dbl)  [unwired: 2 in, 2 out]
        n518 = property on="Z mm/rev" class="DigNum (strict)"() -> ("Value"=w1124:dbl)  [unwired: 2 in, 2 out]
        n519 = Divide(x=w1179, y=w1181) -> (x/y=w1180:dbl)
        n520 = Multiply(x=w1156, y=w1122) -> (x*y=w1155:dbl)
        n521 = Divide(x=w1173, y=w1175) -> (x/y=w1174:dbl)
        n522 = Multiply(x=w1148, y=w1123) -> (x*y=w1147:dbl)
        n523 = Divide(x=w1167, y=w1169) -> (x/y=w1168:dbl)
        n524 = Multiply(x=w1140, y=w1124) -> (x*y=w1139:dbl)
        n525 = Divide(x=w1161, y=w1163) -> (x/y=w1162:dbl)
        n526 = Multiply(x=w1132, y=w1125) -> (x*y=w1131:dbl)
        n527 = Multiply(x=w1180, y=w1122) -> (x*y=w1177:dbl)
        n528 = Add(x=w1155, y=w1150) -> (x+y=w1152:dbl)
        n529 = Multiply(x=w1174, y=w1123) -> (x*y=w1171:dbl)
        n530 = Add(x=w1147, y=w1142) -> (x+y=w1144:dbl)
        n531 = Multiply(x=w1168, y=w1124) -> (x*y=w1165:dbl)
        n532 = Add(x=w1139, y=w1134) -> (x+y=w1136:dbl)
        n533 = Multiply(x=w1162, y=w1125) -> (x*y=w1159:dbl)
        n534 = Add(x=w1131, y=w1126) -> (x+y=w1128:dbl)
        n535 = Absolute Value(x=w1159) -> (abs(x)=w1121:dbl)
        n536 = property on="Y Velocity MV mm/sec" class="DigNum (strict)"("Val(Sgnl)"=w1177) -> ()  [unwired: 2 in, 2 out]
        n537 = property on="Y Position MV mm" class="DigNum (strict)"("Val(Sgnl)"=w1152) -> ()  [unwired: 2 in, 2 out]
        n538 = property on="X Velocity MV mm/sec" class="DigNum (strict)"("Val(Sgnl)"=w1171) -> ()  [unwired: 2 in, 2 out]
        n539 = property on="X Position MV mm" class="DigNum (strict)"("Val(Sgnl)"=w1144) -> ()  [unwired: 2 in, 2 out]
        n540 = property on="Z Velocity MV mm/sec" class="DigNum (strict)"("Val(Sgnl)"=w1165) -> ()  [unwired: 2 in, 2 out]
        n541 = property on="Z Position MV mm" class="DigNum (strict)"("Val(Sgnl)"=w1136) -> ()  [unwired: 2 in, 2 out]
        n542 = property on="R Position MV deg" class="DigNum (strict)"("Val(Sgnl)"=w1128) -> ()  [unwired: 2 in, 2 out]
        n543 = property on="R Velocity MVdeg/sec" class="DigNum (strict)"("Val(Sgnl)"=w1121) -> ()  [unwired: 2 in, 2 out]
      }
      event "Y Scan Length SP steps", "Y Scan Velocity SP steps/sec", "X Scan Velocity SP steps/sec", "X Scan Length SP steps", "Z Scan Velocity SP steps/sec", "Z Scan Length SP steps", "R Scan Velocity SP steps/sec", "R Scan Length SP steps": Value Change {
        n544 = event-data() -> ()  [unwired: 1 in, 5 out]
        n545 = property on="X Step PV" class="DigNum (strict)"() -> ("Value"=w1250:i32)  [unwired: 2 in, 2 out]
        n546 = property on="Y Step PV" class="DigNum (strict)"() -> ("Value"=w1236:i32)  [unwired: 2 in, 2 out]
        n547 = property on="Z Step PV" class="DigNum (strict)"() -> ("Value"=w1223:i32)  [unwired: 2 in, 2 out]
        n548 = property on="R Step PV" class="DigNum (strict)"() -> ("Value"=w1209:i32)  [unwired: 2 in, 2 out]
        n549 = property on="X Step SP" class="DigNum (strict)"() -> ("Maximum"=w1256:dbl)  [unwired: 2 in, 2 out]
        n550 = property on="Y Step SP" class="DigNum (strict)"() -> ("Maximum"=w1242:dbl)  [unwired: 2 in, 2 out]
        n551 = property on="Z Step SP" class="DigNum (strict)"() -> ("Maximum"=w1229:dbl)  [unwired: 2 in, 2 out]
        n552 = property on="R Step SP" class="DigNum (strict)"() -> ("Maximum"=w1217:dbl)  [unwired: 2 in, 2 out]
        n553 = property on="X Step SP" class="DigNum (strict)"() -> ("Minimum"=w1257:dbl)  [unwired: 2 in, 2 out]
        n554 = property on="Y Step SP" class="DigNum (strict)"() -> ("Minimum"=w1243:dbl)  [unwired: 2 in, 2 out]
        n555 = property on="Z Step SP" class="DigNum (strict)"() -> ("Minimum"=w1230:dbl)  [unwired: 2 in, 2 out]
        n556 = property on="R Step SP" class="DigNum (strict)"() -> ("Minimum"=w1214:dbl)  [unwired: 2 in, 2 out]
        n557 = property on="Z steps/rev" class="DigNum (strict)"() -> ("Value"=w1225:u32)  [unwired: 2 in, 2 out]
        n558 = property on="R steps/rev" class="DigNum (strict)"() -> ("Value"=w1211:u32)  [unwired: 2 in, 2 out]
        n559 = property on="X steps/rev" class="DigNum (strict)"() -> ("Value"=w1252:u32)  [unwired: 2 in, 2 out]
        n560 = property on="Y steps/rev" class="DigNum (strict)"() -> ("Value"=w1238:u32)  [unwired: 2 in, 2 out]
        n561 = To Double Precision Float(number=w1250) -> (double precision float=w1203:dbl)
        n562 = To Double Precision Float(number=w1236) -> (double precision float=w1202:dbl)
        n563 = To Double Precision Float(number=w1223) -> (double precision float=w1201:dbl)
        n564 = To Double Precision Float(number=w1209) -> (double precision float=w1200:dbl)
        n565 = Subtract(x=w1257, y=w1203) -> (x-y=w1258:dbl)
        n566 = Subtract(x=w1256, y=w1203) -> (x-y=w1255:dbl)
        n567 = Subtract(x=w1243, y=w1202) -> (x-y=w1244:dbl)
        n568 = Subtract(x=w1242, y=w1202) -> (x-y=w1241:dbl)
        n569 = Subtract(x=w1230, y=w1201) -> (x-y=w1231:dbl)
        n570 = Subtract(x=w1229, y=w1201) -> (x-y=w1228:dbl)
        n571 = Subtract(x=w1214, y=w1200) -> (x-y=w1215:dbl)
        n572 = Subtract(x=w1217, y=w1200) -> (x-y=w1216:dbl)
        n573 = To Double Precision Float(number=w1225) -> (double precision float=w1222:dbl)
        n574 = To Double Precision Float(number=w1211) -> (double precision float=w1208:dbl)
        n575 = To Double Precision Float(number=w1252) -> (double precision float=w1249:dbl)
        n576 = To Double Precision Float(number=w1238) -> (double precision float=w1193:dbl)
        n577 = property on="Z Scan Length SP steps" class="DigNum (strict)"() -> ("Value"=w1226:i32)  [unwired: 2 in, 2 out]
        n578 = property on="R Scan Length SP steps" class="DigNum (strict)"() -> ("Value"=w1212:i32)  [unwired: 2 in, 2 out]
        n579 = property on="X Scan Length SP steps" class="DigNum (strict)"() -> ("Value"=w1248:i32)  [unwired: 2 in, 2 out]
        n580 = property on="Y Scan Length SP steps" class="DigNum (strict)"() -> ("Value"=w1239:i32)  [unwired: 2 in, 2 out]
        n581 = property on="Z Scan Velocity SP steps/sec" class="DigNum (strict)"() -> ("Value"=w1221:i32)  [unwired: 2 in, 2 out]
        n582 = property on="R Scan Velocity SP steps/sec" class="DigNum (strict)"() -> ("Value"=w1207:i32)  [unwired: 2 in, 2 out]
        n583 = property on="X Scan Velocity SP steps/sec" class="DigNum (strict)"() -> ("Value"=w1253:i32)  [unwired: 2 in, 2 out]
        n584 = property on="Y Scan Velocity SP steps/sec" class="DigNum (strict)"() -> ("Value"=w1235:i32)  [unwired: 2 in, 2 out]
        n585 = To Double Precision Float(number=w1226) -> (double precision float=w1199:dbl)
        n586 = To Double Precision Float(number=w1212) -> (double precision float=w1197:dbl)
        n587 = To Double Precision Float(number=w1248) -> (double precision float=w1188:dbl)
        n588 = To Double Precision Float(number=w1239) -> (double precision float=w1192:dbl)
        n589 = property on="X Scan Length SP steps" class="DigNum (strict)"("Maximum"=w1255) -> ()  [unwired: 2 in, 2 out]
        n590 = property on="Y Scan Length SP steps" class="DigNum (strict)"("Maximum"=w1241) -> ()  [unwired: 2 in, 2 out]
        n591 = property on="Z Scan Length SP steps" class="DigNum (strict)"("Maximum"=w1228) -> ()  [unwired: 2 in, 2 out]
        n592 = property on="R Scan Length SP steps" class="DigNum (strict)"("Maximum"=w1216) -> ()  [unwired: 2 in, 2 out]
        n593 = property on="X Scan Length SP steps" class="DigNum (strict)"("Minimum"=w1258) -> ()  [unwired: 2 in, 2 out]
        n594 = property on="Y Scan Length SP steps" class="DigNum (strict)"("Minimum"=w1244) -> ()  [unwired: 2 in, 2 out]
        n595 = property on="Z Scan Length SP steps" class="DigNum (strict)"("Minimum"=w1231) -> ()  [unwired: 2 in, 2 out]
        n596 = property on="R Scan Length SP steps" class="DigNum (strict)"("Minimum"=w1215) -> ()  [unwired: 2 in, 2 out]
        n597 = Divide(x=w1197, y=w1208) -> (x/y=w1213:dbl)
        n598 = Divide(x=w1199, y=w1222) -> (x/y=w1227:dbl)
        n599 = Divide(x=w1188, y=w1249) -> (x/y=w1247:dbl)
        n600 = Divide(x=w1192, y=w1193) -> (x/y=w1240:dbl)
        n601 = To Double Precision Float(number=w1207) -> (double precision float=w1196:dbl)
        n602 = To Double Precision Float(number=w1221) -> (double precision float=w1198:dbl)
        n603 = To Double Precision Float(number=w1253) -> (double precision float=w1187:dbl)
        n604 = To Double Precision Float(number=w1235) -> (double precision float=w1191:dbl)
        n605 = property on="R deg/rev" class="DigNum (strict)"() -> ("Value"=w1210:dbl)  [unwired: 2 in, 2 out]
        n606 = property on="Z mm/rev" class="DigNum (strict)"() -> ("Value"=w1224:dbl)  [unwired: 2 in, 2 out]
        n607 = property on="X mm/rev" class="DigNum (strict)"() -> ("Value"=w1251:dbl)  [unwired: 2 in, 2 out]
        n608 = property on="Y mm/rev" class="DigNum (strict)"() -> ("Value"=w1237:dbl)  [unwired: 2 in, 2 out]
        n609 = Multiply(x=w1227, y=w1224) -> (x*y=w1219:dbl)
        n610 = Divide(x=w1199, y=w1198) -> (x/y=w1194:dbl)
        n611 = Divide(x=w1198, y=w1222) -> (x/y=w1220:dbl)
        n612 = Multiply(x=w1213, y=w1210) -> (x*y=w1205:dbl)
        n613 = Divide(x=w1197, y=w1196) -> (x/y=w1195:dbl)
        n614 = Divide(x=w1196, y=w1208) -> (x/y=w1206:dbl)
        n615 = Divide(x=w1188, y=w1187) -> (x/y=w1189:dbl)
        n616 = Divide(x=w1187, y=w1249) -> (x/y=w1254:dbl)
        n617 = Multiply(x=w1251, y=w1247) -> (x*y=w1245:dbl)
        n618 = Multiply(x=w1240, y=w1237) -> (x*y=w1233:dbl)
        n619 = Divide(x=w1192, y=w1191) -> (x/y=w1190:dbl)
        n620 = Divide(x=w1191, y=w1193) -> (x/y=w1234:dbl)
        n621 = Multiply(x=w1224, y=w1220) -> (x*y=w1218:dbl)
        n622 = Multiply(x=w1210, y=w1206) -> (x*y=w1204:dbl)
        n623 = Multiply(x=w1254, y=w1251) -> (x*y=w1246:dbl)
        n624 = Multiply(x=w1237, y=w1234) -> (x*y=w1232:dbl)
        n625 = Absolute Value(x=w1194) -> (abs(x)=→"Z Scan Duration":dbl)
        n626 = Absolute Value(x=w1195) -> (abs(x)=→"R Scan Duration":dbl)
        n627 = Absolute Value(x=w1189) -> (abs(x)=→"X Scan Duration":dbl)
        n628 = Absolute Value(x=w1190) -> (abs(x)=→"Y Scan Duration":dbl)
        n629 = property on="Z Scan length MV mm" class="DigNum (strict)"("Value"=w1219) -> ()  [unwired: 2 in, 2 out]
        n630 = property on="R Scan length MV deg" class="DigNum (strict)"("Value"=w1205) -> ()  [unwired: 2 in, 2 out]
        n631 = property on="Y Scan length MV mm" class="DigNum (strict)"("Value"=w1233) -> ()  [unwired: 2 in, 2 out]
        n632 = property on="X Scan length MV mm" class="DigNum (strict)"("Val(Sgnl)"=w1245) -> ()  [unwired: 2 in, 2 out]
        n633 = Absolute Value(x=w1204) -> (abs(x)=w1186:dbl)
        n634 = property on="X Scan velocity MV mm/sec" class="DigNum (strict)"("Value"=w1246) -> ()  [unwired: 2 in, 2 out]
        n635 = property on="Z Scan velocity MV mm/sec" class="DigNum (strict)"("Val(Sgnl)"=w1218) -> ()  [unwired: 2 in, 2 out]
        n636 = property on="Y Scan velocity MV mm/sec" class="DigNum (strict)"("Val(Sgnl)"=w1232) -> ()  [unwired: 2 in, 2 out]
        n637 = property on="R Scan Velocity SP deg/sec" class="DigNum (strict)"("Val(Sgnl)"=w1186) -> ()  [unwired: 2 in, 2 out]
      }
      event "Y Move Set": Mouse Down {
        n638 = event-data() -> ()  [unwired: 1 in, 7 out]
        n639 = property on="Y Step SP" class="DigNum (strict)"() -> ("Maximum"=w1269:dbl)  [unwired: 2 in, 2 out]
        n640 = property on="Y Step SP" class="DigNum (strict)"() -> ("Minimum"=w1268:dbl)  [unwired: 2 in, 2 out]
        n641 = property on="Y steps/rev" class="DigNum (strict)"() -> ("Value"=w1275:u32)  [unwired: 2 in, 2 out]
        n642 = property on="Y offset mm" class="DigNum (strict)"() -> ("Value"=w1273:dbl)  [unwired: 2 in, 2 out]
        n643 = property on="Y Velocity SP step/sec" class="DigNum (strict)"() -> ("Maximum"=w1262:dbl)  [unwired: 2 in, 2 out]
        n644 = property on="Y Velocity SP step/sec" class="DigNum (strict)"() -> ("Minimum"=w1261:dbl)  [unwired: 2 in, 2 out]
        n645 = property on="Y Position SP mm" class="DigNum (strict)"() -> ("Value"=w1272:dbl)  [unwired: 2 in, 2 out]
        n646 = property on="Y mm/rev" class="DigNum (strict)"() -> ("Value"=w1259:dbl)  [unwired: 2 in, 2 out]
        n647 = property on="Y Velocity SP mm/sec" class="DigNum (strict)"() -> ("Value"=w1266:dbl)  [unwired: 2 in, 2 out]
        n648 = Subtract(x=w1272, y=w1273) -> (x-y=w1276:dbl)
        n649 = Divide(x=w1266, y=w1259) -> (x/y=w1267:dbl)
        n650 = To Double Precision Float(number=w1275) -> (double precision float=w1260:dbl)
        n651 = Divide(x=w1276, y=w1259) -> (x/y=w1277:dbl)
        n652 = Multiply(x=w1267, y=w1260) -> (x*y=w1264:dbl)
        n653 = Multiply(x=w1277, y=w1260) -> (x*y=w1271:dbl)
        n654 = In Range and Coerce(upper limit=w1262, x=w1264, lower limit=w1261) -> (coerced(x)=w1263:dbl)  [unwired: 1 out]
        n655 = To Long Integer(number=w1263) -> (32bit integer=w1265:i32)
        n656 = In Range and Coerce(upper limit=w1269, x=w1271, lower limit=w1268) -> (coerced(x)=w1270:dbl)  [unwired: 1 out]
        n657 = To Long Integer(number=w1270) -> (32bit integer=w1274:i32)
        n658 = property on="Y Velocity SP step/sec" class="DigNum (strict)"("Val(Sgnl)"=w1265) -> ()  [unwired: 2 in, 2 out]
        n659 = property on="Y Step SP" class="DigNum (strict)"("Val(Sgnl)"=w1274) -> ()  [unwired: 2 in, 2 out]
      }
      event "X Move Set": Mouse Down {
        n660 = event-data() -> ()  [unwired: 1 in, 7 out]
        n661 = property on="X Step SP" class="DigNum (strict)"() -> ("Maximum"=w1288:dbl)  [unwired: 2 in, 2 out]
        n662 = property on="X Step SP" class="DigNum (strict)"() -> ("Minimum"=w1287:dbl)  [unwired: 2 in, 2 out]
        n663 = property on="X steps/rev" class="DigNum (strict)"() -> ("Value"=w1294:u32)  [unwired: 2 in, 2 out]
        n664 = property on="X offset mm" class="DigNum (strict)"() -> ("Value"=w1292:dbl)  [unwired: 2 in, 2 out]
        n665 = property on="X Velocity SP step/sec" class="DigNum (strict)"() -> ("Maximum"=w1281:dbl)  [unwired: 2 in, 2 out]
        n666 = property on="X Velocity SP step/sec" class="DigNum (strict)"() -> ("Minimum"=w1280:dbl)  [unwired: 2 in, 2 out]
        n667 = property on="X Position SP mm" class="DigNum (strict)"() -> ("Value"=w1291:dbl)  [unwired: 2 in, 2 out]
        n668 = property on="X mm/rev" class="DigNum (strict)"() -> ("Value"=w1278:dbl)  [unwired: 2 in, 2 out]
        n669 = property on="X Velocity SP mm/sec" class="DigNum (strict)"() -> ("Value"=w1285:dbl)  [unwired: 2 in, 2 out]
        n670 = Subtract(x=w1291, y=w1292) -> (x-y=w1295:dbl)
        n671 = Divide(x=w1285, y=w1278) -> (x/y=w1286:dbl)
        n672 = To Double Precision Float(number=w1294) -> (double precision float=w1279:dbl)
        n673 = Divide(x=w1295, y=w1278) -> (x/y=w1296:dbl)
        n674 = Multiply(x=w1286, y=w1279) -> (x*y=w1283:dbl)
        n675 = Multiply(x=w1296, y=w1279) -> (x*y=w1290:dbl)
        n676 = In Range and Coerce(upper limit=w1281, x=w1283, lower limit=w1280) -> (coerced(x)=w1282:dbl)  [unwired: 1 out]
        n677 = To Long Integer(number=w1282) -> (32bit integer=w1284:i32)
        n678 = In Range and Coerce(upper limit=w1288, x=w1290, lower limit=w1287) -> (coerced(x)=w1289:dbl)  [unwired: 1 out]
        n679 = To Long Integer(number=w1289) -> (32bit integer=w1293:i32)
        n680 = property on="X Velocity SP step/sec" class="DigNum (strict)"("Val(Sgnl)"=w1284) -> ()  [unwired: 2 in, 2 out]
        n681 = property on="X Step SP" class="DigNum (strict)"("Val(Sgnl)"=w1293) -> ()  [unwired: 2 in, 2 out]
      }
      event "Z Move Set": Mouse Down {
        n682 = event-data() -> ()  [unwired: 1 in, 7 out]
        n683 = property on="Z Step SP" class="DigNum (strict)"() -> ("Maximum"=w1305:dbl)  [unwired: 2 in, 2 out]
        n684 = property on="Z Step SP" class="DigNum (strict)"() -> ("Minimum"=w1304:dbl)  [unwired: 2 in, 2 out]
        n685 = property on="Z steps/rev" class="DigNum (strict)"() -> ("Value"=w1311:u32)  [unwired: 2 in, 2 out]
        n686 = property on="Z offset mm" class="DigNum (strict)"() -> ("Value"=w1309:dbl)  [unwired: 2 in, 2 out]
        n687 = property on="Z Velocity SP step/sec" class="DigNum (strict)"() -> ("Maximum"=w1298:dbl)  [unwired: 2 in, 2 out]
        n688 = property on="Z Velocity SP step/sec" class="DigNum (strict)"() -> ("Minimum"=w1297:dbl)  [unwired: 2 in, 2 out]
        n689 = property on="Z Position SP mm" class="DigNum (strict)"() -> ("Value"=w1308:dbl)  [unwired: 2 in, 2 out]
        n690 = property on="Z mm/rev" class="DigNum (strict)"() -> ("Value"=w1314:dbl)  [unwired: 2 in, 2 out]
        n691 = property on="Z Velocity SP mm/sec" class="DigNum (strict)"() -> ("Value"=w1302:dbl)  [unwired: 2 in, 2 out]
        n692 = Subtract(x=w1308, y=w1309) -> (x-y=w1312:dbl)
        n693 = Divide(x=w1302, y=w1314) -> (x/y=w1303:dbl)
        n694 = To Double Precision Float(number=w1311) -> (double precision float=w1315:dbl)
        n695 = Divide(x=w1312, y=w1314) -> (x/y=w1313:dbl)
        n696 = Multiply(x=w1303, y=w1315) -> (x*y=w1300:dbl)
        n697 = Multiply(x=w1313, y=w1315) -> (x*y=w1307:dbl)
        n698 = In Range and Coerce(upper limit=w1298, x=w1300, lower limit=w1297) -> (coerced(x)=w1299:dbl)  [unwired: 1 out]
        n699 = To Long Integer(number=w1299) -> (32bit integer=w1301:i32)
        n700 = In Range and Coerce(upper limit=w1305, x=w1307, lower limit=w1304) -> (coerced(x)=w1306:dbl)  [unwired: 1 out]
        n701 = To Long Integer(number=w1306) -> (32bit integer=w1310:i32)
        n702 = property on="Z Velocity SP step/sec" class="DigNum (strict)"("Val(Sgnl)"=w1301) -> ()  [unwired: 2 in, 2 out]
        n703 = property on="Z Step SP" class="DigNum (strict)"("Val(Sgnl)"=w1310) -> ()  [unwired: 2 in, 2 out]
      }
      event "R Move Set": Mouse Down {
        n704 = event-data() -> ()  [unwired: 1 in, 7 out]
        n705 = property on="R Step SP" class="DigNum (strict)"() -> ("Maximum"=w1327:dbl)  [unwired: 2 in, 2 out]
        n706 = property on="R Step SP" class="DigNum (strict)"() -> ("Minimum"=w1326:dbl)  [unwired: 2 in, 2 out]
        n707 = property on="R steps/rev" class="DigNum (strict)"() -> ("Value"=w1333:u32)  [unwired: 2 in, 2 out]
        n708 = property on="R offset deg" class="DigNum (strict)"() -> ("Value"=w1331:dbl)  [unwired: 2 in, 2 out]
        n709 = property on="R Velocity SP step/sec" class="DigNum (strict)"() -> ("Maximum"=w1320:dbl)  [unwired: 2 in, 2 out]
        n710 = property on="R Velocity SP step/sec" class="DigNum (strict)"() -> ("Minimum"=w1319:dbl)  [unwired: 2 in, 2 out]
        n711 = To Double Precision Float(number=w1333) -> (double precision float=w1318:dbl)
        n712 = property on="R Position SP deg" class="DigNum (strict)"() -> ("Value"=w1330:dbl)  [unwired: 2 in, 2 out]
        n713 = property on="R deg/rev" class="DigNum (strict)"() -> ("Value"=w1317:dbl)  [unwired: 2 in, 2 out]
        n714 = property on="R Velocity SP deg/sec" class="DigNum (strict)"() -> ("Value"=w1324:dbl)  [unwired: 2 in, 2 out]
        n715 = Subtract(x=w1330, y=w1331) -> (x-y=w1334:dbl)
        n716 = Divide(x=w1324, y=w1317) -> (x/y=w1325:dbl)
        n717 = Divide(x=w1334, y=w1317) -> (x/y=w1335:dbl)
        n718 = Multiply(x=w1325, y=w1318) -> (x*y=w1322:dbl)
        n719 = Multiply(x=w1335, y=w1318) -> (x*y=w1329:dbl)
        n720 = Absolute Value(x=w1322) -> (abs(x)=w1316:dbl)
        n721 = In Range and Coerce(upper limit=w1327, x=w1329, lower limit=w1326) -> (coerced(x)=w1328:dbl)  [unwired: 1 out]
        n722 = In Range and Coerce(upper limit=w1320, x=w1316, lower limit=w1319) -> (coerced(x)=w1321:dbl)  [unwired: 1 out]
        n723 = To Long Integer(number=w1328) -> (32bit integer=w1332:i32)
        n724 = To Long Integer(number=w1321) -> (32bit integer=w1323:i32)
        n725 = property on="R Step SP" class="DigNum (strict)"("Val(Sgnl)"=w1332) -> ()  [unwired: 2 in, 2 out]
        n726 = property on="R Velocity SP step/sec" class="DigNum (strict)"("Val(Sgnl)"=w1323) -> ()  [unwired: 2 in, 2 out]
      }
      event "Y Scan set": Mouse Down {
        n727 = event-data() -> ()  [unwired: 1 in, 7 out]
        n728 = property on="Y Step SP" class="DigNum (strict)"() -> ("Maximum"=w1345:dbl)  [unwired: 2 in, 2 out]
        n729 = property on="Y Step SP" class="DigNum (strict)"() -> ("Minimum"=w1346:dbl)  [unwired: 2 in, 2 out]
        n730 = property on="Y steps/rev" class="DigNum (strict)"() -> ("Value"=w1351:u32)  [unwired: 2 in, 2 out]
        n731 = To Double Precision Float(number=w1351) -> (double precision float=w1337:dbl)
        n732 = property on="Y Scan Length SP mm" class="DigNum (strict)"() -> ("Value"=w1349:dbl)  [unwired: 2 in, 2 out]
        n733 = property on="Y mm/rev" class="DigNum (strict)"() -> ("Value"=w1336:dbl)  [unwired: 2 in, 2 out]
        n734 = property on="Y Scan Velocity SP steps/sec" class="DigNum (strict)"() -> ("Maximum"=w1339:dbl)  [unwired: 2 in, 2 out]
        n735 = property on="Y Scan Velocity SP steps/sec" class="DigNum (strict)"() -> ("Minimum"=w1338:dbl)  [unwired: 2 in, 2 out]
        n736 = Divide(x=w1349, y=w1336) -> (x/y=w1352:dbl)
        n737 = property on="Y Scan Velocity SP mm/sec" class="DigNum (strict)"() -> ("Value"=w1343:dbl)  [unwired: 2 in, 2 out]
        n738 = Multiply(x=w1352, y=w1337) -> (x*y=w1348:dbl)
        n739 = Divide(x=w1343, y=w1336) -> (x/y=w1344:dbl)
        n740 = Multiply(x=w1344, y=w1337) -> (x*y=w1341:dbl)
        n741 = In Range and Coerce(upper limit=w1345, x=w1348, lower limit=w1346) -> (coerced(x)=w1347:dbl)  [unwired: 1 out]
        n742 = To Long Integer(number=w1347) -> (32bit integer=w1350:i32)
        n743 = In Range and Coerce(upper limit=w1339, x=w1341, lower limit=w1338) -> (coerced(x)=w1340:dbl)  [unwired: 1 out]
        n744 = To Long Integer(number=w1340) -> (32bit integer=w1342:i32)
        n745 = property on="Y Scan Length SP steps" class="DigNum (strict)"("Val(Sgnl)"=w1350) -> ()  [unwired: 2 in, 2 out]
        n746 = property on="Y Scan Velocity SP steps/sec" class="DigNum (strict)"("Val(Sgnl)"=w1342) -> ()  [unwired: 2 in, 2 out]
      }
      event "X Scan set": Mouse Down {
        n747 = event-data() -> ()  [unwired: 1 in, 7 out]
        n748 = property on="X Step SP" class="DigNum (strict)"() -> ("Maximum"=w1362:dbl)  [unwired: 2 in, 2 out]
        n749 = property on="X Step SP" class="DigNum (strict)"() -> ("Minimum"=w1363:dbl)  [unwired: 2 in, 2 out]
        n750 = property on="X steps/rev" class="DigNum (strict)"() -> ("Value"=w1368:u32)  [unwired: 2 in, 2 out]
        n751 = To Double Precision Float(number=w1368) -> (double precision float=w1354:dbl)
        n752 = property on="X Scan Length SP mm" class="DigNum (strict)"() -> ("Value"=w1366:dbl)  [unwired: 2 in, 2 out]
        n753 = property on="X mm/rev" class="DigNum (strict)"() -> ("Value"=w1353:dbl)  [unwired: 2 in, 2 out]
        n754 = property on="X Scan Velocity SP steps/sec" class="DigNum (strict)"() -> ("Maximum"=w1356:dbl)  [unwired: 2 in, 2 out]
        n755 = property on="X Scan Velocity SP steps/sec" class="DigNum (strict)"() -> ("Minimum"=w1355:dbl)  [unwired: 2 in, 2 out]
        n756 = Divide(x=w1366, y=w1353) -> (x/y=w1369:dbl)
        n757 = property on="X Scan Velocity SP mm/sec" class="DigNum (strict)"() -> ("Value"=w1360:dbl)  [unwired: 2 in, 2 out]
        n758 = Multiply(x=w1369, y=w1354) -> (x*y=w1365:dbl)
        n759 = Divide(x=w1360, y=w1353) -> (x/y=w1361:dbl)
        n760 = Multiply(x=w1361, y=w1354) -> (x*y=w1358:dbl)
        n761 = In Range and Coerce(upper limit=w1362, x=w1365, lower limit=w1363) -> (coerced(x)=w1364:dbl)  [unwired: 1 out]
        n762 = To Long Integer(number=w1364) -> (32bit integer=w1367:i32)
        n763 = In Range and Coerce(upper limit=w1356, x=w1358, lower limit=w1355) -> (coerced(x)=w1357:dbl)  [unwired: 1 out]
        n764 = To Long Integer(number=w1357) -> (32bit integer=w1359:i32)
        n765 = property on="X Scan Length SP steps" class="DigNum (strict)"("Val(Sgnl)"=w1367) -> ()  [unwired: 2 in, 2 out]
        n766 = property on="X Scan Velocity SP steps/sec" class="DigNum (strict)"("Val(Sgnl)"=w1359) -> ()  [unwired: 2 in, 2 out]
      }
      event "Z Scan set": Mouse Down {
        n767 = event-data() -> ()  [unwired: 1 in, 7 out]
        n768 = property on="Z Step SP" class="DigNum (strict)"() -> ("Maximum"=w1379:dbl)  [unwired: 2 in, 2 out]
        n769 = property on="Z Step SP" class="DigNum (strict)"() -> ("Minimum"=w1380:dbl)  [unwired: 2 in, 2 out]
        n770 = property on="Z steps/rev" class="DigNum (strict)"() -> ("Value"=w1385:u32)  [unwired: 2 in, 2 out]
        n771 = To Double Precision Float(number=w1385) -> (double precision float=w1371:dbl)
        n772 = property on="Z Scan Length SP mm" class="DigNum (strict)"() -> ("Value"=w1383:dbl)  [unwired: 2 in, 2 out]
        n773 = property on="Z mm/rev" class="DigNum (strict)"() -> ("Value"=w1370:dbl)  [unwired: 2 in, 2 out]
        n774 = property on="Z Scan Velocity SP steps/sec" class="DigNum (strict)"() -> ("Maximum"=w1373:dbl)  [unwired: 2 in, 2 out]
        n775 = property on="Z Scan Velocity SP steps/sec" class="DigNum (strict)"() -> ("Minimum"=w1372:dbl)  [unwired: 2 in, 2 out]
        n776 = property on="Z Scan Velocity SP mm/sec" class="DigNum (strict)"() -> ("Value"=w1377:dbl)  [unwired: 2 in, 2 out]
        n777 = Divide(x=w1383, y=w1370) -> (x/y=w1386:dbl)
        n778 = Multiply(x=w1386, y=w1371) -> (x*y=w1382:dbl)
        n779 = Divide(x=w1377, y=w1370) -> (x/y=w1378:dbl)
        n780 = Multiply(x=w1378, y=w1371) -> (x*y=w1375:dbl)
        n781 = In Range and Coerce(upper limit=w1379, x=w1382, lower limit=w1380) -> (coerced(x)=w1381:dbl)  [unwired: 1 out]
        n782 = To Long Integer(number=w1381) -> (32bit integer=w1384:i32)
        n783 = In Range and Coerce(upper limit=w1373, x=w1375, lower limit=w1372) -> (coerced(x)=w1374:dbl)  [unwired: 1 out]
        n784 = To Long Integer(number=w1374) -> (32bit integer=w1376:i32)
        n785 = property on="Z Scan Length SP steps" class="DigNum (strict)"("Val(Sgnl)"=w1384) -> ()  [unwired: 2 in, 2 out]
        n786 = property on="Z Scan Velocity SP steps/sec" class="DigNum (strict)"("Val(Sgnl)"=w1376) -> ()  [unwired: 2 in, 2 out]
      }
      event "R Scan set": Mouse Down {
        n787 = event-data() -> ()  [unwired: 1 in, 7 out]
        n788 = property on="R Step SP" class="DigNum (strict)"() -> ("Maximum"=w1397:dbl)  [unwired: 2 in, 2 out]
        n789 = property on="R Step SP" class="DigNum (strict)"() -> ("Minimum"=w1398:dbl)  [unwired: 2 in, 2 out]
        n790 = property on="R steps/rev" class="DigNum (strict)"() -> ("Value"=w1403:u32)  [unwired: 2 in, 2 out]
        n791 = property on="R Velocity SP step/sec" class="DigNum (strict)"() -> ("Maximum"=w1391:dbl)  [unwired: 2 in, 2 out]
        n792 = To Double Precision Float(number=w1403) -> (double precision float=w1389:dbl)
        n793 = property on="R Scan Length SP deg" class="DigNum (strict)"() -> ("Value"=w1401:dbl)  [unwired: 2 in, 2 out]
        n794 = property on="R deg/rev" class="DigNum (strict)"() -> ("Value"=w1388:dbl)  [unwired: 2 in, 2 out]
        n795 = property on="R Scan Velocity SP steps/sec" class="DigNum (strict)"() -> ("Minimum"=w1390:dbl)  [unwired: 2 in, 2 out]
        n796 = property on="R Scan Velocity SP deg/sec" class="DigNum (strict)"() -> ("Value"=w1395:dbl)  [unwired: 2 in, 2 out]
        n797 = Divide(x=w1401, y=w1388) -> (x/y=w1404:dbl)
        n798 = Multiply(x=w1404, y=w1389) -> (x*y=w1400:dbl)
        n799 = Divide(x=w1395, y=w1388) -> (x/y=w1396:dbl)
        n800 = Multiply(x=w1396, y=w1389) -> (x*y=w1393:dbl)
        n801 = In Range and Coerce(upper limit=w1397, x=w1400, lower limit=w1398) -> (coerced(x)=w1399:dbl)  [unwired: 1 out]
        n802 = To Long Integer(number=w1399) -> (32bit integer=w1402:i32)
        n803 = Absolute Value(x=w1393) -> (abs(x)=w1387:dbl)
        n804 = In Range and Coerce(upper limit=w1391, x=w1387, lower limit=w1390) -> (coerced(x)=w1392:dbl)  [unwired: 1 out]
        n805 = property on="R Scan Length SP steps" class="DigNum (strict)"("Val(Sgnl)"=w1402) -> ()  [unwired: 2 in, 2 out]
        n806 = To Long Integer(number=w1392) -> (32bit integer=w1394:i32)
        n807 = property on="R Scan Velocity SP steps/sec" class="DigNum (strict)"("Val(Sgnl)"=w1394) -> ()  [unwired: 2 in, 2 out]
      }
      event "Y Go": Mouse Up {
        n808 = event-data() -> ()  [unwired: 1 in, 7 out]
        n809 = flat-sequence {
          tunnel: w1409 -> [w1419]
          tunnel: w1410 -> [w1420]
          tunnel: [w1420] -> w1406
          tunnel: [w1419] -> w1405
          tunnel: [w1423] -> w1408
          tunnel: [w1422] -> w1407
          tunnel: w1406 -> [w1425]
          tunnel: w1405 -> [w1424]
          tunnel: [w1443] -> w1412
          tunnel: [w1442] -> w1411
          tunnel: w1408 -> [w1441]
          tunnel: w1407 -> [w1440]
          tunnel: [w1450] -> w1414
          tunnel: [w1449] -> w1413
          tunnel: w1412 -> [w1448]
          tunnel: w1411 -> [w1447]
          tunnel: [w1456] -> w1415
          tunnel: [w1457] -> w1416
          tunnel: w1414 -> [w1457]
          tunnel: w1413 -> [w1455]
          frame #0 {
            n810 = property on="Scan Go" class="Bool"("DisabledEnum"=T2."Disabled and Grayed Out" ("Disabled")) -> ()  [unwired: 2 in, 2 out]
            n811 = property on="Y Go" class="Bool"("DisabledEnum"=T2."Disabled and Grayed Out" ("Disabled")) -> ()  [unwired: 2 in, 2 out]
          }
          frame #1 {
            n812 = property on="Y Step SP" class="DigNum (strict)"() -> ("Value"=w1433:i32)  [unwired: 2 in, 2 out]
            n813 = property on="Y Step PV" class="DigNum (strict)"() -> ("Value"=w1432:i32)  [unwired: 2 in, 2 out]
            n814 = property on="Y Backlash" class="DigNum (strict)"() -> ("Value"=w1421:i32)  [unwired: 2 in, 2 out]
            n815 = Subtract(x=w1433, y=w1432) -> (x-y=w1431:i32)
            n816 = Sign(1:w1421) -> (0:w1429:i32)
            n817 = Sign(1:w1431) -> (0:w1430:i32)
            n818 = Multiply(x=w1430, y=w1429) -> (x*y=w1428:i32)
            n819 = Equal?(x=w1428, y=1) -> (x = y?=w1426:bool)
            n820 = case shown="False" w1426 {
              tunnel: w1425 -> [w1436 w1438]
              tunnel: w1424 -> [w1435 w1437]
              tunnel: [w1435 w1437] -> w1423
              tunnel: [w1436 w1438] -> w1422
              frame False {
                n821 = property on="Y Backlash corr" class="Bool (strict)"("Val(Sgnl)"=FALSE ("Value (Signaling)")) -> ()  [unwired: 2 in, 2 out]
              }
              frame True {
                n822 = property on="Y Backlash corr" class="Bool (strict)"("Val(Sgnl)"=TRUE ("Value (Signaling)")) -> ()  [unwired: 2 in, 2 out]
              }
            }
          }
          frame #2 {
            # "Velocity Setting"
            n823 = property on="Y Velocity SP step/sec" class="DigNum (strict)"() -> ("Value"=w1444:i32)  [unwired: 2 in, 2 out]
            n824 = Number To Decimal String(number=w1444) -> (decimal integer string=w1445:string)  [unwired: 1 in]
            n825 = call "mDrive Send Command.vi"("error in (no error)"=w1441, "Extra"=w1445, "Command"=T1."Max Velocity", "VISA resource name"=w1440) -> ("error out"=w1442:errorcluster, "VISA resource name out"=w1443:refnum<visa-resource-name>)  [unwired: 3 in, 1 out]
          }
          frame #3 {
            # "Move to Abs Position"
            n826 = property on="Y Step SP" class="DigNum (strict)"() -> ("Value"=w1453:i32)  [unwired: 2 in, 2 out]
            n827 = Number To Decimal String(number=w1453) -> (decimal integer string=w1452:string)  [unwired: 1 in]
            n828 = call "mDrive Send Command.vi"("error in (no error)"=w1447, "Extra"=w1452, "Command"=T1."Move to Absolute Position", "VISA resource name"=w1448) -> ("error out"=w1449:errorcluster, "VISA resource name out"=w1450:refnum<visa-resource-name>)  [unwired: 3 in, 1 out]
          }
          frame #4 {
            n829 = call "Time Delay"("error in (no error)"=w1455, "Delay Time (s)"=0.1) -> ("error out"=w1456:errorcluster)  [unwired: 9 in]
          }
        }
      }
      event "Z Go": Mouse Up {
        n830 = event-data() -> ()  [unwired: 1 in, 7 out]
        n831 = flat-sequence {
          tunnel: w1460 -> [w1472]
          tunnel: w1461 -> [w1473]
          tunnel: [w1473] -> w1463
          tunnel: [w1472] -> w1462
          tunnel: [w1476] -> w1465
          tunnel: [w1475] -> w1464
          tunnel: w1463 -> [w1478]
          tunnel: w1462 -> [w1477]
          tunnel: [w1496] -> w1467
          tunnel: [w1495] -> w1466
          tunnel: w1465 -> [w1494]
          tunnel: w1464 -> [w1493]
          tunnel: [w1503] -> w1469
          tunnel: [w1502] -> w1468
          tunnel: w1467 -> [w1501]
          tunnel: w1466 -> [w1500]
          tunnel: [w1509] -> w1459
          tunnel: [w1510] -> w1458
          tunnel: w1469 -> [w1510]
          tunnel: w1468 -> [w1508]
          frame #0 {
            n832 = property on="Scan Go" class="Bool"("DisabledEnum"=T2."Disabled and Grayed Out" ("Disabled")) -> ()  [unwired: 2 in, 2 out]
            n833 = property on="Z Go" class="Bool"("DisabledEnum"=T2."Disabled and Grayed Out" ("Disabled")) -> ()  [unwired: 2 in, 2 out]
          }
          frame #1 {
            n834 = property on="Z Step SP" class="DigNum (strict)"() -> ("Value"=w1486:i32)  [unwired: 2 in, 2 out]
            n835 = property on="Z Step PV" class="DigNum (strict)"() -> ("Value"=w1485:i32)  [unwired: 2 in, 2 out]
            n836 = property on="Z Backlash" class="DigNum (strict)"() -> ("Value"=w1474:i32)  [unwired: 2 in, 2 out]
            n837 = Subtract(x=w1486, y=w1485) -> (x-y=w1484:i32)
            n838 = Sign(1:w1474) -> (0:w1482:i32)
            n839 = Sign(1:w1484) -> (0:w1483:i32)
            n840 = Multiply(x=w1483, y=w1482) -> (x*y=w1481:i32)
            n841 = Equal?(x=w1481, y=1) -> (x = y?=w1479:bool)
            n842 = case shown="True" w1479 {
              tunnel: w1478 -> [w1489 w1491]
              tunnel: w1477 -> [w1488 w1490]
              tunnel: [w1488 w1490] -> w1476
              tunnel: [w1489 w1491] -> w1475
              frame False {
                n843 = property on="Z Backlash corr" class="Bool (strict)"("Val(Sgnl)"=FALSE ("Value (Signaling)")) -> ()  [unwired: 2 in, 2 out]
              }
              frame True {
                n844 = property on="Z Backlash corr" class="Bool (strict)"("Val(Sgnl)"=TRUE ("Value (Signaling)")) -> ()  [unwired: 2 in, 2 out]
              }
            }
          }
          frame #2 {
            # "Velocity Setting"
            n845 = property on="Z Velocity SP step/sec" class="DigNum (strict)"() -> ("Value"=w1497:i32)  [unwired: 2 in, 2 out]
            n846 = Number To Decimal String(number=w1497) -> (decimal integer string=w1498:string)  [unwired: 1 in]
            n847 = call "mDrive Send Command.vi"("error in (no error)"=w1494, "Extra"=w1498, "Command"=T1."Max Velocity", "VISA resource name"=w1493) -> ("error out"=w1495:errorcluster, "VISA resource name out"=w1496:refnum<visa-resource-name>)  [unwired: 3 in, 1 out]
          }
          frame #3 {
            # "Move to Abs Position"
            n848 = property on="Z Step SP" class="DigNum (strict)"() -> ("Value"=w1506:i32)  [unwired: 2 in, 2 out]
            n849 = Number To Decimal String(number=w1506) -> (decimal integer string=w1505:string)  [unwired: 1 in]
            n850 = call "mDrive Send Command.vi"("error in (no error)"=w1500, "Extra"=w1505, "Command"=T1."Move to Absolute Position", "VISA resource name"=w1501) -> ("error out"=w1502:errorcluster, "VISA resource name out"=w1503:refnum<visa-resource-name>)  [unwired: 3 in, 1 out]
          }
          frame #4 {
            n851 = call "Time Delay28"("error in (no error)"=w1508, "Delay Time (s)"=0.1) -> ("error out"=w1509:errorcluster)  [unwired: 9 in]
          }
        }
      }
      event "R Go": Mouse Up {
        n852 = event-data() -> ()  [unwired: 1 in, 7 out]
        n853 = flat-sequence {
          tunnel: w1513 -> [w1525]
          tunnel: w1514 -> [w1526]
          tunnel: [w1526] -> w1516
          tunnel: [w1525] -> w1515
          tunnel: [w1529] -> w1518
          tunnel: [w1528] -> w1517
          tunnel: w1516 -> [w1531]
          tunnel: w1515 -> [w1530]
          tunnel: [w1549] -> w1520
          tunnel: [w1548] -> w1519
          tunnel: w1518 -> [w1547]
          tunnel: w1517 -> [w1546]
          tunnel: [w1556] -> w1522
          tunnel: [w1555] -> w1521
          tunnel: w1520 -> [w1554]
          tunnel: w1519 -> [w1553]
          tunnel: [w1562] -> w1512
          tunnel: [w1563] -> w1511
          tunnel: w1522 -> [w1563]
          tunnel: w1521 -> [w1561]
          frame #0 {
            n854 = property on="Scan Go" class="Bool"("DisabledEnum"=T2."Disabled and Grayed Out" ("Disabled")) -> ()  [unwired: 2 in, 2 out]
            n855 = property on="R Go" class="Bool"("DisabledEnum"=T2."Disabled and Grayed Out" ("Disabled")) -> ()  [unwired: 2 in, 2 out]
          }
          frame #1 {
            n856 = property on="R Step SP" class="DigNum (strict)"() -> ("Value"=w1539:i32)  [unwired: 2 in, 2 out]
            n857 = property on="R Step PV" class="DigNum (strict)"() -> ("Value"=w1538:i32)  [unwired: 2 in, 2 out]
            n858 = property on="R Backlash" class="DigNum (strict)"() -> ("Value"=w1527:i32)  [unwired: 2 in, 2 out]
            n859 = Subtract(x=w1539, y=w1538) -> (x-y=w1537:i32)
            n860 = Sign(1:w1527) -> (0:w1535:i32)
            n861 = Sign(1:w1537) -> (0:w1536:i32)
            n862 = Multiply(x=w1536, y=w1535) -> (x*y=w1534:i32)
            n863 = Equal?(x=w1534, y=1) -> (x = y?=w1532:bool)
            n864 = case shown="True" w1532 {
              tunnel: w1531 -> [w1542 w1544]
              tunnel: w1530 -> [w1541 w1543]
              tunnel: [w1541 w1543] -> w1529
              tunnel: [w1542 w1544] -> w1528
              frame False {
                n865 = property on="R Backlash corr" class="Bool (strict)"("Val(Sgnl)"=FALSE ("Value (Signaling)")) -> ()  [unwired: 2 in, 2 out]
              }
              frame True {
                n866 = property on="R Backlash corr" class="Bool (strict)"("Val(Sgnl)"=TRUE ("Value (Signaling)")) -> ()  [unwired: 2 in, 2 out]
              }
            }
          }
          frame #2 {
            # "Velocity Setting"
            n867 = property on="R Velocity SP step/sec" class="DigNum (strict)"() -> ("Value"=w1550:i32)  [unwired: 2 in, 2 out]
            n868 = Number To Decimal String(number=w1550) -> (decimal integer string=w1551:string)  [unwired: 1 in]
            n869 = call "mDrive Send Command.vi"("error in (no error)"=w1547, "Extra"=w1551, "Command"=T1."Max Velocity", "VISA resource name"=w1546) -> ("error out"=w1548:errorcluster, "VISA resource name out"=w1549:refnum<visa-resource-name>)  [unwired: 3 in, 1 out]
          }
          frame #3 {
            # "Move to Abs Position"
            n870 = property on="R Step SP" class="DigNum (strict)"() -> ("Value"=w1559:i32)  [unwired: 2 in, 2 out]
            n871 = Number To Decimal String(number=w1559) -> (decimal integer string=w1558:string)  [unwired: 1 in]
            n872 = call "mDrive Send Command.vi"("error in (no error)"=w1553, "Extra"=w1558, "Command"=T1."Move to Absolute Position", "VISA resource name"=w1554) -> ("error out"=w1555:errorcluster, "VISA resource name out"=w1556:refnum<visa-resource-name>)  [unwired: 3 in, 1 out]
          }
          frame #4 {
            n873 = call "Time Delay29"("error in (no error)"=w1561, "Delay Time (s)"=0.1) -> ("error out"=w1562:errorcluster)  [unwired: 9 in]
          }
        }
      }
      event "X Go": Mouse Up {
        n874 = event-data() -> ()  [unwired: 1 in, 7 out]
        n875 = flat-sequence {
          tunnel: [w1577] -> w1569
          tunnel: [w1576] -> w1568
          tunnel: w1567 -> [w1577]
          tunnel: w1566 -> [w1576]
          tunnel: [w1582] -> w1571
          tunnel: [w1581] -> w1570
          tunnel: w1569 -> [w1584]
          tunnel: w1568 -> [w1583]
          tunnel: [w1602] -> w1573
          tunnel: [w1601] -> w1572
          tunnel: w1571 -> [w1600]
          tunnel: w1570 -> [w1599]
          tunnel: [w1609] -> w1575
          tunnel: [w1608] -> w1574
          tunnel: w1573 -> [w1607]
          tunnel: w1572 -> [w1606]
          tunnel: [w1615] -> w1564
          tunnel: [w1616] -> w1565
          tunnel: w1575 -> [w1616]
          tunnel: w1574 -> [w1614]
          frame #0 {
            n876 = property on="Scan Go" class="Bool"("DisabledEnum"=T2."Disabled and Grayed Out" ("Disabled")) -> ()  [unwired: 2 in, 2 out]
            n877 = property on="X Go" class="Bool"("DisabledEnum"=T2."Disabled and Grayed Out" ("Disabled")) -> ()  [unwired: 2 in, 2 out]
          }
          frame #1 {
            n878 = property on="X Step SP" class="DigNum (strict)"() -> ("Value"=w1592:i32)  [unwired: 2 in, 2 out]
            n879 = property on="X Step PV" class="DigNum (strict)"() -> ("Value"=w1591:i32)  [unwired: 2 in, 2 out]
            n880 = property on="X Backlash" class="DigNum (strict)"() -> ("Value"=w1580:i32)  [unwired: 2 in, 2 out]
            n881 = Subtract(x=w1592, y=w1591) -> (x-y=w1590:i32)
            n882 = Sign(1:w1580) -> (0:w1588:i32)
            n883 = Sign(1:w1590) -> (0:w1589:i32)
            n884 = Multiply(x=w1589, y=w1588) -> (x*y=w1587:i32)
            n885 = Equal?(x=w1587, y=1) -> (x = y?=w1585:bool)
            n886 = case shown="True" w1585 {
              tunnel: w1584 -> [w1595 w1597]
              tunnel: w1583 -> [w1594 w1596]
              tunnel: [w1594 w1596] -> w1582
              tunnel: [w1595 w1597] -> w1581
              frame False {
                n887 = property on="X Backlash corr" class="Bool (strict)"("Val(Sgnl)"=FALSE ("Value (Signaling)")) -> ()  [unwired: 2 in, 2 out]
              }
              frame True {
                n888 = property on="X Backlash corr" class="Bool (strict)"("Val(Sgnl)"=TRUE ("Value (Signaling)")) -> ()  [unwired: 2 in, 2 out]
              }
            }
          }
          frame #2 {
            # "Velocity Setting"
            n889 = property on="X Velocity SP step/sec" class="DigNum (strict)"() -> ("Value"=w1603:i32)  [unwired: 2 in, 2 out]
            n890 = Number To Decimal String(number=w1603) -> (decimal integer string=w1604:string)  [unwired: 1 in]
            n891 = call "mDrive Send Command.vi"("error in (no error)"=w1600, "Extra"=w1604, "Command"=T1."Max Velocity", "VISA resource name"=w1599) -> ("error out"=w1601:errorcluster, "VISA resource name out"=w1602:refnum<visa-resource-name>)  [unwired: 3 in, 1 out]
          }
          frame #3 {
            # "Move to Abs Position"
            n892 = property on="X Step SP" class="DigNum (strict)"() -> ("Value"=w1612:i32)  [unwired: 2 in, 2 out]
            n893 = Number To Decimal String(number=w1612) -> (decimal integer string=w1611:string)  [unwired: 1 in]
            n894 = call "mDrive Send Command.vi"("error in (no error)"=w1606, "Extra"=w1611, "Command"=T1."Move to Absolute Position", "VISA resource name"=w1607) -> ("error out"=w1608:errorcluster, "VISA resource name out"=w1609:refnum<visa-resource-name>)  [unwired: 3 in, 1 out]
          }
          frame #4 {
            n895 = call "Time Delay15"("error in (no error)"=w1614, "Delay Time (s)"=0.1) -> ("error out"=w1615:errorcluster)  [unwired: 9 in]
          }
        }
      }
      event "X Scan OK": Mouse Up {
        n896 = event-data() -> ()  [unwired: 1 in, 7 out]
        n897 = flat-sequence {
          tunnel: [w1632] -> w1624
          tunnel: [w1630] -> w1623
          tunnel: w1622 -> [w1626]
          tunnel: w1621 -> [w1625]
          tunnel: w1624 -> [w1647]
          tunnel: w1623 -> [w1646]
          tunnel: [w1647] -> w1618
          tunnel: [w1646] -> w1617
          tunnel: [w1649] -> w1619
          tunnel: [w1650] -> w1620
          tunnel: w1618 -> [w1650]
          tunnel: w1617 -> [w1649]
          frame #0 {
            # "VELOCITY"
            n898 = property on="X Scan Velocity SP steps/sec" class="DigNum (strict)"() -> ("Value"=w1633:i32)  [unwired: 2 in, 2 out]
            n899 = Number To Decimal String(number=w1633) -> (decimal integer string=w1634:string)  [unwired: 1 in]
            n900 = call "mDrive Send Command.vi"("error in (no error)"=w1625, "Extra"=w1634, "Command"=T1."Max Velocity", "VISA resource name"=w1626) -> ("error out"=w1635:errorcluster, "VISA resource name out"=w1640:refnum<visa-resource-name>)  [unwired: 3 in, 1 out]
            n901 = call "Time Delay9"("error in (no error)"=w1635) -> ("error out"=w1638:errorcluster)  [unwired: 10 in]
            n902 = call "mDrive Send Command.vi"("error in (no error)"=w1638, "Extra"="VM", "Command"=T1."Print Parameter", "VISA resource name"=w1640) -> ("error out"=w1631:errorcluster, "read buffer"=w1636:string, "VISA resource name out"=w1632:refnum<visa-resource-name>)  [unwired: 3 in]
            n903 = call "Time Delay10"("error in (no error)"=w1631) -> ("error out"=w1630:errorcluster)  [unwired: 10 in]
            n904 = Decimal String To Number(string=w1636, offset=0) -> (number=w1639:i32)  [unwired: 1 in, 1 out]
            n905 = property on="X velocity PV step/sec" class="DigNum (strict)"("Val(Sgnl)"=w1639) -> ()  [unwired: 2 in, 2 out]
          }
          frame #1 {
            n906 = property on="X Scan" class="Bool (strict)"("Val(Sgnl)"=TRUE ("Slew Ready 2")) -> ()  [unwired: 2 in, 2 out]
            n907 = property on="Scan Cancel" class="Bool"("DisabledEnum"=T2."Enabled" ("Disabled")) -> ()  [unwired: 2 in, 2 out]
            n908 = property on="Scan Go" class="Bool"("DisabledEnum"=T2."Enabled" ("Disabled")) -> ()  [unwired: 2 in, 2 out]
            n909 = property on="X Scan Length SP steps" class="DigNum (strict)"("DisabledEnum"=T2."Disabled and Grayed Out" ("Disabled")) -> ()  [unwired: 2 in, 2 out]
            n910 = property on="X Scan Velocity SP steps/sec" class="DigNum (strict)"("DisabledEnum"=T2."Disabled and Grayed Out" ("Disabled")) -> ()  [unwired: 2 in, 2 out]
          }
          frame #2 {
            n911 = property on="X Go" class="Bool"("DisabledEnum"=T2."Disabled and Grayed Out" ("Disabled")) -> ()  [unwired: 2 in, 2 out]
          }
        }
      }
      event "Y Scan OK": Mouse Up {
        n912 = event-data() -> ()  [unwired: 1 in, 7 out]
        n913 = flat-sequence {
          tunnel: w1658 -> [w1668]
          tunnel: w1657 -> [w1667]
          tunnel: [w1664] -> w1655
          tunnel: [w1662] -> w1654
          tunnel: w1655 -> [w1681]
          tunnel: w1654 -> [w1680]
          tunnel: [w1681] -> w1652
          tunnel: [w1680] -> w1651
          tunnel: [w1683] -> w1656
          tunnel: [w1684] -> w1653
          tunnel: w1652 -> [w1684]
          tunnel: w1651 -> [w1683]
          frame #0 {
            # "VELOCITY"
            n914 = property on="Y Scan Velocity SP steps/sec" class="DigNum (strict)"() -> ("Value"=w1665:i32)  [unwired: 2 in, 2 out]
            n915 = Number To Decimal String(number=w1665) -> (decimal integer string=w1666:string)  [unwired: 1 in]
            n916 = call "mDrive Send Command.vi"("error in (no error)"=w1668, "Extra"=w1666, "Command"=T1."Max Velocity", "VISA resource name"=w1667) -> ("error out"=w1669:errorcluster, "VISA resource name out"=w1674:refnum<visa-resource-name>)  [unwired: 3 in, 1 out]
            n917 = call "Time Delay5"("error in (no error)"=w1669) -> ("error out"=w1672:errorcluster)  [unwired: 10 in]
            n918 = call "mDrive Send Command.vi"("error in (no error)"=w1672, "Extra"="VM", "Command"=T1."Print Parameter", "VISA resource name"=w1674) -> ("error out"=w1663:errorcluster, "read buffer"=w1670:string, "VISA resource name out"=w1664:refnum<visa-resource-name>)  [unwired: 3 in]
            n919 = Decimal String To Number(string=w1670, offset=0) -> (number=w1673:i32)  [unwired: 1 in, 1 out]
            n920 = call "Time Delay6"("error in (no error)"=w1663) -> ("error out"=w1662:errorcluster)  [unwired: 10 in]
            n921 = property on="Y velocity PV step/sec" class="DigNum (strict)"("Val(Sgnl)"=w1673) -> ()  [unwired: 2 in, 2 out]
          }
          frame #1 {
            n922 = property on="Y Scan" class="Bool (strict)"("Val(Sgnl)"=TRUE ("Slew Ready 2")) -> ()  [unwired: 2 in, 2 out]
            n923 = property on="Scan Cancel" class="Bool"("DisabledEnum"=T2."Enabled" ("Disabled")) -> ()  [unwired: 2 in, 2 out]
            n924 = property on="Scan Go" class="Bool"("DisabledEnum"=T2."Enabled" ("Disabled")) -> ()  [unwired: 2 in, 2 out]
            n925 = property on="Y Scan Length SP steps" class="DigNum (strict)"("DisabledEnum"=T2."Disabled and Grayed Out" ("Disabled")) -> ()  [unwired: 2 in, 2 out]
            n926 = property on="Y Scan Velocity SP steps/sec" class="DigNum (strict)"("DisabledEnum"=T2."Disabled and Grayed Out" ("Disabled")) -> ()  [unwired: 2 in, 2 out]
          }
          frame #2 {
            n927 = property on="Y Go" class="Bool"("DisabledEnum"=T2."Disabled and Grayed Out" ("Disabled")) -> ()  [unwired: 2 in, 2 out]
          }
        }
      }
      event "Z Scan OK": Mouse Up {
        n928 = event-data() -> ()  [unwired: 1 in, 7 out]
        n929 = flat-sequence {
          tunnel: [w1700] -> w1692
          tunnel: [w1698] -> w1691
          tunnel: w1688 -> [w1694]
          tunnel: w1687 -> [w1693]
          tunnel: w1692 -> [w1715]
          tunnel: w1691 -> [w1714]
          tunnel: [w1715] -> w1690
          tunnel: [w1714] -> w1689
          tunnel: [w1717] -> w1686
          tunnel: [w1718] -> w1685
          tunnel: w1690 -> [w1718]
          tunnel: w1689 -> [w1717]
          frame #0 {
            # "VELOCITY"
            n930 = property on="Z Scan Velocity SP steps/sec" class="DigNum (strict)"() -> ("Value"=w1701:i32)  [unwired: 2 in, 2 out]
            n931 = Number To Decimal String(number=w1701) -> (decimal integer string=w1702:string)  [unwired: 1 in]
            n932 = call "mDrive Send Command.vi"("error in (no error)"=w1693, "Extra"=w1702, "Command"=T1."Max Velocity", "VISA resource name"=w1694) -> ("error out"=w1703:errorcluster, "VISA resource name out"=w1708:refnum<visa-resource-name>)  [unwired: 3 in, 1 out]
            n933 = call "Time Delay24"("error in (no error)"=w1703) -> ("error out"=w1706:errorcluster)  [unwired: 10 in]
            n934 = call "mDrive Send Command.vi"("error in (no error)"=w1706, "Extra"="VM", "Command"=T1."Print Parameter", "VISA resource name"=w1708) -> ("error out"=w1699:errorcluster, "read buffer"=w1704:string, "VISA resource name out"=w1700:refnum<visa-resource-name>)  [unwired: 3 in]
            n935 = Decimal String To Number(string=w1704, offset=0) -> (number=w1707:i32)  [unwired: 1 in, 1 out]
            n936 = call "Time Delay25"("error in (no error)"=w1699) -> ("error out"=w1698:errorcluster)  [unwired: 10 in]
            n937 = property on="Z  velocity PV step/sec" class="DigNum (strict)"("Val(Sgnl)"=w1707) -> ()  [unwired: 2 in, 2 out]
          }
          frame #1 {
            n938 = property on="Z Scan" class="Bool (strict)"("Val(Sgnl)"=TRUE ("Slew Ready 2")) -> ()  [unwired: 2 in, 2 out]
            n939 = property on="Scan Cancel" class="Bool"("DisabledEnum"=T2."Enabled" ("Disabled")) -> ()  [unwired: 2 in, 2 out]
            n940 = property on="Scan Go" class="Bool"("DisabledEnum"=T2."Enabled" ("Disabled")) -> ()  [unwired: 2 in, 2 out]
            n941 = property on="Z Scan Length SP steps" class="DigNum (strict)"("DisabledEnum"=T2."Disabled and Grayed Out" ("Disabled")) -> ()  [unwired: 2 in, 2 out]
            n942 = property on="Z Scan Velocity SP steps/sec" class="DigNum (strict)"("DisabledEnum"=T2."Disabled and Grayed Out" ("Disabled")) -> ()  [unwired: 2 in, 2 out]
          }
          frame #2 {
            n943 = property on="Z Go" class="Bool"("DisabledEnum"=T2."Disabled and Grayed Out" ("Disabled")) -> ()  [unwired: 2 in, 2 out]
          }
        }
      }
      event "R Scan OK": Mouse Up {
        n944 = event-data() -> ()  [unwired: 1 in, 7 out]
        n945 = flat-sequence {
          tunnel: [w1734] -> w1726
          tunnel: [w1732] -> w1725
          tunnel: w1722 -> [w1728]
          tunnel: w1721 -> [w1727]
          tunnel: w1726 -> [w1749]
          tunnel: w1725 -> [w1748]
          tunnel: [w1749] -> w1724
          tunnel: [w1748] -> w1723
          tunnel: [w1751] -> w1719
          tunnel: [w1752] -> w1720
          tunnel: w1724 -> [w1752]
          tunnel: w1723 -> [w1751]
          frame #0 {
            # "VELOCITY"
            n946 = property on="R Scan Velocity SP steps/sec" class="DigNum (strict)"() -> ("Value"=w1735:i32)  [unwired: 2 in, 2 out]
            n947 = Number To Decimal String(number=w1735) -> (decimal integer string=w1736:string)  [unwired: 1 in]
            n948 = call "mDrive Send Command.vi"("error in (no error)"=w1727, "Extra"=w1736, "Command"=T1."Max Velocity", "VISA resource name"=w1728) -> ("error out"=w1737:errorcluster, "VISA resource name out"=w1742:refnum<visa-resource-name>)  [unwired: 3 in, 1 out]
            n949 = call "Time Delay26"("error in (no error)"=w1737) -> ("error out"=w1740:errorcluster)  [unwired: 10 in]
            n950 = call "mDrive Send Command.vi"("error in (no error)"=w1740, "Extra"="VM", "Command"=T1."Print Parameter", "VISA resource name"=w1742) -> ("error out"=w1733:errorcluster, "read buffer"=w1738:string, "VISA resource name out"=w1734:refnum<visa-resource-name>)  [unwired: 3 in]
            n951 = Decimal String To Number(string=w1738, offset=0) -> (number=w1741:i32)  [unwired: 1 in, 1 out]
            n952 = call "Time Delay27"("error in (no error)"=w1733) -> ("error out"=w1732:errorcluster)  [unwired: 10 in]
            n953 = property on="R velocity PV step/sec" class="DigNum (strict)"("Val(Sgnl)"=w1741) -> ()  [unwired: 2 in, 2 out]
          }
          frame #1 {
            n954 = property on="R Scan" class="Bool (strict)"("Val(Sgnl)"=TRUE ("Slew Ready 2")) -> ()  [unwired: 2 in, 2 out]
            n955 = property on="Scan Cancel" class="Bool"("DisabledEnum"=T2."Enabled" ("Disabled")) -> ()  [unwired: 2 in, 2 out]
            n956 = property on="Scan Go" class="Bool"("DisabledEnum"=T2."Enabled" ("Disabled")) -> ()  [unwired: 2 in, 2 out]
            n957 = property on="R Scan Length SP steps" class="DigNum (strict)"("DisabledEnum"=T2."Disabled and Grayed Out" ("Disabled")) -> ()  [unwired: 2 in, 2 out]
            n958 = property on="R Scan Velocity SP steps/sec" class="DigNum (strict)"("DisabledEnum"=T2."Disabled and Grayed Out" ("Disabled")) -> ()  [unwired: 2 in, 2 out]
          }
          frame #2 {
            n959 = property on="R Go" class="Bool"("DisabledEnum"=T2."Disabled and Grayed Out" ("Disabled")) -> ()  [unwired: 2 in, 2 out]
          }
        }
      }
      event Application Instance Close? {
        n960 = event-data() -> ()  [unwired: 1 in, 4 out]
        n961 = event-data() -> ()  [unwired: 3 in, 1 out]
      }
      event "Stop": Mouse Down {
        n962 = event-data() -> ()  [unwired: 1 in, 7 out]
        n963 = flat-sequence {
          tunnel: [w1784] -> w1766
          tunnel: [w1783] -> w1765
          tunnel: w1764 -> [w1782]
          tunnel: w1763 -> [w1781]
          frame #0 {
            n964 = call "mDrive Send Command.vi"("error in (no error)"=w1781, "Command"=T1."Stop", "VISA resource name"=w1782) -> ("error out"=w1783:errorcluster, "VISA resource name out"=w1784:refnum<visa-resource-name>)  [unwired: 4 in, 1 out]
          }
        }
        n965 = flat-sequence {
          tunnel: w1770 -> [w1790]
          tunnel: w1769 -> [w1789]
          tunnel: [w1788] -> w1768
          tunnel: [w1787] -> w1767
          frame #0 {
            n966 = call "mDrive Send Command.vi"("error in (no error)"=w1789, "Command"=T1."Stop", "VISA resource name"=w1790) -> ("error out"=w1787:errorcluster, "VISA resource name out"=w1788:refnum<visa-resource-name>)  [unwired: 4 in, 1 out]
          }
        }
        n967 = flat-sequence {
          tunnel: [w1779] -> w1760
          tunnel: [w1778] -> w1759
          tunnel: w1762 -> [w1777]
          tunnel: w1761 -> [w1776]
          frame #0 {
            n968 = call "mDrive Send Command.vi"("error in (no error)"=w1776, "Command"=T1."Stop", "VISA resource name"=w1777) -> ("error out"=w1778:errorcluster, "VISA resource name out"=w1779:refnum<visa-resource-name>)  [unwired: 4 in, 1 out]
          }
        }
        n969 = flat-sequence {
          tunnel: w1758 -> [w1775]
          tunnel: w1757 -> [w1774]
          tunnel: [w1773] -> w1756
          tunnel: [w1771] -> _
          tunnel: [w1771] -> w1755
          frame #0 {
            n970 = call "mDrive Send Command.vi"("error in (no error)"=w1774, "Command"=T1."Stop", "VISA resource name"=w1775) -> ("error out"=w1771:errorcluster, "VISA resource name out"=w1773:refnum<visa-resource-name>)  [unwired: 4 in, 1 out]
          }
        }
      }
      event "Scan Cancel": Mouse Down {
        n971 = event-data() -> ()  [unwired: 1 in, 7 out]
        n972 = flat-sequence {
          tunnel: w1806 -> [w1845]
          tunnel: w1805 -> [w1844]
          tunnel: [w1847] -> w1808
          tunnel: [w1846] -> w1807
          tunnel: [w1854] -> w1803
          tunnel: [w1855] -> w1804
          tunnel: w1808 -> [w1855]
          tunnel: w1807 -> [w1854]
          frame #0 {
            n973 = call "mDrive Send Command.vi"("error in (no error)"=w1844, "Command"=T1."Stop", "VISA resource name"=w1845) -> ("error out"=w1846:errorcluster, "VISA resource name out"=w1847:refnum<visa-resource-name>)  [unwired: 4 in, 1 out]
          }
          frame #1 {
            n974 = property on="X Scan" class="Bool (strict)"("Value"=FALSE ("Slew Ready")) -> ()  [unwired: 2 in, 2 out]
            n975 = property on="X Scan set" class="Bool"("DisabledEnum"=T2."Enabled" ("Disabled")) -> ()  [unwired: 2 in, 2 out]
            n976 = property on="X Scan Velocity SP steps/sec" class="DigNum (strict)"("DisabledEnum"=T2."Enabled" ("Disabled")) -> ()  [unwired: 2 in, 2 out]
            n977 = property on="X Scan Length SP steps" class="DigNum (strict)"("DisabledEnum"=T2."Enabled" ("Disabled")) -> ()  [unwired: 2 in, 2 out]
            n978 = property on="X Go" class="Bool"("DisabledEnum"=T2."Enabled" ("Disabled")) -> ()  [unwired: 2 in, 2 out]
            n979 = property on="X Scan OK" class="Bool"("DisabledEnum"=T2."Enabled" ("Disabled")) -> ()  [unwired: 2 in, 2 out]
          }
        }
        n980 = flat-sequence {
          tunnel: w1814 -> [w1858]
          tunnel: w1813 -> [w1857]
          tunnel: [w1860] -> w1810
          tunnel: [w1859] -> w1809
          tunnel: [w1867] -> w1815
          tunnel: [w1868] -> w1816
          tunnel: w1810 -> [w1868]
          tunnel: w1809 -> [w1867]
          frame #0 {
            n981 = call "mDrive Send Command.vi"("error in (no error)"=w1857, "Command"=T1."Stop", "VISA resource name"=w1858) -> ("error out"=w1859:errorcluster, "VISA resource name out"=w1860:refnum<visa-resource-name>)  [unwired: 4 in, 1 out]
          }
          frame #1 {
            n982 = property on="Y Scan" class="Bool (strict)"("Value"=FALSE ("Slew Ready")) -> ()  [unwired: 2 in, 2 out]
            n983 = property on="Y Go" class="Bool"("DisabledEnum"=T2."Enabled" ("Disabled")) -> ()  [unwired: 2 in, 2 out]
            n984 = property on="Y Scan Velocity SP steps/sec" class="DigNum (strict)"("DisabledEnum"=T2."Enabled" ("Disabled")) -> ()  [unwired: 2 in, 2 out]
            n985 = property on="Y Scan set" class="Bool"("DisabledEnum"=T2."Enabled" ("Disabled")) -> ()  [unwired: 2 in, 2 out]
            n986 = property on="Y Scan OK" class="Bool"("DisabledEnum"=T2."Enabled" ("Disabled")) -> ()  [unwired: 2 in, 2 out]
            n987 = property on="Y Scan Length SP steps" class="DigNum (strict)"("DisabledEnum"=T2."Enabled" ("Disabled")) -> ()  [unwired: 2 in, 2 out]
          }
        }
        n988 = flat-sequence {
          tunnel: [w1834] -> w1802
          tunnel: [w1833] -> w1801
          tunnel: w1800 -> [w1831]
          tunnel: w1799 -> [w1830]
          tunnel: [w1841] -> w1797
          tunnel: [w1842] -> w1798
          tunnel: w1802 -> [w1842]
          tunnel: w1801 -> [w1841]
          frame #0 {
            n989 = call "mDrive Send Command.vi"("error in (no error)"=w1830, "Command"=T1."Stop", "VISA resource name"=w1831) -> ("error out"=w1833:errorcluster, "VISA resource name out"=w1834:refnum<visa-resource-name>)  [unwired: 4 in, 1 out]
          }
          frame #1 {
            n990 = property on="Z Scan" class="Bool (strict)"("Value"=FALSE ("Slew Ready")) -> ()  [unwired: 2 in, 2 out]
            n991 = property on="Z Scan set" class="Bool"("DisabledEnum"=T2."Enabled" ("Disabled")) -> ()  [unwired: 2 in, 2 out]
            n992 = property on="Z Scan Velocity SP steps/sec" class="DigNum (strict)"("DisabledEnum"=T2."Enabled" ("Disabled")) -> ()  [unwired: 2 in, 2 out]
            n993 = property on="Z Scan Length SP steps" class="DigNum (strict)"("DisabledEnum"=T2."Enabled" ("Disabled")) -> ()  [unwired: 2 in, 2 out]
            n994 = property on="Z Go" class="Bool"("DisabledEnum"=T2."Enabled" ("Disabled")) -> ()  [unwired: 2 in, 2 out]
            n995 = property on="Z Scan OK" class="Bool"("DisabledEnum"=T2."Enabled" ("Disabled")) -> ()  [unwired: 2 in, 2 out]
          }
        }
        n996 = flat-sequence {
          tunnel: [w1821] -> w1796
          tunnel: [w1820] -> w1795
          tunnel: w1794 -> [w1818]
          tunnel: w1793 -> [w1817]
          tunnel: [w1828] -> w1791
          tunnel: [w1829] -> w1792
          tunnel: w1796 -> [w1829]
          tunnel: w1795 -> [w1828]
          frame #0 {
            n997 = call "mDrive Send Command.vi"("error in (no error)"=w1817, "Command"=T1."Stop", "VISA resource name"=w1818) -> ("error out"=w1820:errorcluster, "VISA resource name out"=w1821:refnum<visa-resource-name>)  [unwired: 4 in, 1 out]
          }
          frame #1 {
            n998 = property on="R Scan" class="Bool (strict)"("Value"=FALSE ("Slew Ready")) -> ()  [unwired: 2 in, 2 out]
            n999 = property on="R Scan Velocity SP steps/sec" class="DigNum (strict)"("DisabledEnum"=T2."Enabled" ("Disabled")) -> ()  [unwired: 2 in, 2 out]
            n1000 = property on="R Go" class="Bool"("DisabledEnum"=T2."Enabled" ("Disabled")) -> ()  [unwired: 2 in, 2 out]
            n1001 = property on="R Scan OK" class="Bool"("DisabledEnum"=T2."Enabled" ("Disabled")) -> ()  [unwired: 2 in, 2 out]
            n1002 = property on="R Scan Length SP steps" class="DigNum (strict)"("DisabledEnum"=T2."Enabled" ("Disabled")) -> ()  [unwired: 2 in, 2 out]
            n1003 = property on="R Scan set" class="Bool"("DisabledEnum"=T2."Enabled" ("Disabled")) -> ()  [unwired: 2 in, 2 out]
          }
        }
        n1004 = property on="Scan Go" class="Bool"("DisabledEnum"=T2."Disabled and Grayed Out" ("Disabled")) -> ()  [unwired: 2 in, 2 out]
        n1005 = property on="Scan Cancel" class="Bool"("DisabledEnum"=T2."Disabled and Grayed Out" ("Disabled")) -> ()  [unwired: 2 in, 2 out]
      }
      event "Scan Go": Mouse Up {
        n1006 = event-data() -> ()  [unwired: 1 in, 7 out]
        n1007 = flat-sequence {
          tunnel: [w1948] -> w1932
          tunnel: [w1946] -> w1925
          tunnel: [w1947] -> w1922
          tunnel: [w1941] -> w1921
          tunnel: [w1945] -> w1920
          tunnel: [w1944] -> w1919
          tunnel: [w1943] -> w1918
          tunnel: [w1942] -> w1917
          tunnel: w1896 -> [w1940]
          tunnel: [w1940] -> w1895
          tunnel: w1894 -> [w1939]
          tunnel: [w1939] -> w1893
          tunnel: w1892 -> [w1938]
          tunnel: [w1938] -> w1891
          tunnel: w1890 -> [w1937]
          tunnel: [w1937] -> w1889
          tunnel: w1888 -> [w1936]
          tunnel: [w1936] -> w1887
          tunnel: w1886 -> [w1935]
          tunnel: [w1935] -> w1885
          tunnel: [w1934] -> w1884
          tunnel: w1883 -> [w1934]
          tunnel: [w1933] -> w1882
          tunnel: w1881 -> [w1933]
          tunnel: [w2000] -> w1929
          tunnel: [w1999] -> w1927
          tunnel: w1932 -> [w1998]
          tunnel: w1925 -> [w1997]
          tunnel: [w1997] -> w1923
          tunnel: w1922 -> [w1996]
          tunnel: w1921 -> [w1985]
          tunnel: w1920 -> [w1995]
          tunnel: w1919 -> [w1991]
          tunnel: w1918 -> [w1988]
          tunnel: w1917 -> [w1994]
          tunnel: [w1993] -> w1915
          tunnel: [w1992] -> w1913
          tunnel: [w1991] -> w1910
          tunnel: [w1990] -> w1908
          tunnel: [w1989] -> w1906
          tunnel: [w1988] -> w1904
          tunnel: [w1987] -> w1902
          tunnel: [w1986] -> w1900
          tunnel: [w1985] -> w1899
          tunnel: w1895 -> [w1984]
          tunnel: w1893 -> [w1983]
          tunnel: w1891 -> [w1982]
          tunnel: w1889 -> [w1981]
          tunnel: w1887 -> [w1980]
          tunnel: w1885 -> [w1979]
          tunnel: w1884 -> [w1978]
          tunnel: w1882 -> [w1977]
          tunnel: w1929 -> [w2041]
          tunnel: [w2041] -> w1928
          tunnel: w1927 -> [w2040]
          tunnel: [w2040] -> w1926
          tunnel: [w2038] -> w1924
          tunnel: w1923 -> [w2038]
          tunnel: [w2037] -> w1916
          tunnel: w1915 -> [w2037]
          tunnel: [w2036] -> w1914
          tunnel: w1913 -> [w2036]
          tunnel: [w2035] -> w1912
          tunnel: [w2034] -> w1911
          tunnel: w1910 -> [w2034]
          tunnel: [w2033] -> w1909
          tunnel: w1908 -> [w2033]
          tunnel: [w2032] -> w1907
          tunnel: w1906 -> [w2032]
          tunnel: [w2031] -> w1905
          tunnel: w1904 -> [w2031]
          tunnel: [w2030] -> w1903
          tunnel: w1902 -> [w2030]
          tunnel: [w2029] -> w1901
          tunnel: w1900 -> [w2029]
          tunnel: w1899 -> [w2035]
          tunnel: w1928 -> [w2061]
          tunnel: [w2059] -> w1931
          tunnel: w1926 -> [w2060]
          tunnel: [w2058] -> w1930
          tunnel: w1924 -> [w2057]
          tunnel: w1916 -> [w2056]
          tunnel: w1914 -> [w2055]
          tunnel: w1912 -> [w2054]
          tunnel: w1911 -> [w2053]
          tunnel: w1909 -> [w2052]
          tunnel: w1907 -> [w2051]
          tunnel: w1905 -> [w2050]
          tunnel: w1903 -> [w2049]
          tunnel: w1901 -> [w2048]
          tunnel: [w2047] -> w1898
          tunnel: [w2046] -> w1897
          tunnel: [w2045] -> w1876
          tunnel: [w2044] -> w1873
          tunnel: [w2043] -> w1871
          tunnel: [w2042] -> w1869
          tunnel: w1931 -> [w2119]
          tunnel: w1930 -> [w2118]
          tunnel: [w2119] -> w1880
          tunnel: [w2118] -> w1879
          tunnel: [w2112] -> w1878
          tunnel: w1898 -> [w2112]
          tunnel: [w2111] -> w1877
          tunnel: w1897 -> [w2111]
          tunnel: w1876 -> [w2101]
          tunnel: [w2101] -> w1875
          tunnel: [w2100] -> w1874
          tunnel: w1873 -> [w2100]
          tunnel: [w2099] -> w1872
          tunnel: w1871 -> [w2099]
          tunnel: [w2098] -> w1870
          tunnel: w1869 -> [w2098]
          frame #0 {
            n1008 = property on="X Scan" class="Bool (strict)"() -> ("Value"=w1941:bool)  [unwired: 2 in, 2 out]
            n1009 = property on="Y Scan" class="Bool (strict)"() -> ("Value"=w1946:bool)  [unwired: 2 in, 2 out]
            n1010 = property on="Z Scan" class="Bool (strict)"() -> ("Value"=w1943:bool)  [unwired: 2 in, 2 out]
            n1011 = property on="R Scan" class="Bool (strict)"() -> ("Value"=w1944:bool)  [unwired: 2 in, 2 out]
            n1012 = case shown="True" w1941 {
              tunnel: ["" w1964] -> w1947
              frame False {
              }
              frame True {
                n1013 = property on="X Scan Length SP steps" class="DigNum (strict)"() -> ("Value"=w1969:i32)  [unwired: 2 in, 2 out]
                n1014 = Number To Decimal String(number=w1969) -> (decimal integer string=w1966:string)  [unwired: 1 in]
                n1015 = call <vilib>:"Space Constant.vi"() -> ("String"=w1967:string)
                n1016 = Concatenate Strings("MR", w1967, w1966, "\r") -> (w1964:string)
              }
            }
            n1017 = case shown="True" w1946 {
              tunnel: ["" w1971] -> w1948
              frame False {
              }
              frame True {
                n1018 = property on="Y Scan Length SP steps" class="DigNum (strict)"() -> ("Value"=w1976:i32)  [unwired: 2 in, 2 out]
                n1019 = Number To Decimal String(number=w1976) -> (decimal integer string=w1973:string)  [unwired: 1 in]
                n1020 = call <vilib>:"Space Constant.vi"() -> ("String"=w1974:string)
                n1021 = Concatenate Strings("MR", w1974, w1973, "\r") -> (w1971:string)
              }
            }
            n1022 = case shown="True" w1943 {
              tunnel: ["" w1957] -> w1945
              frame False {
              }
              frame True {
                n1023 = property on="Z Scan Length SP steps" class="DigNum (strict)"() -> ("Value"=w1962:i32)  [unwired: 2 in, 2 out]
                n1024 = Number To Decimal String(number=w1962) -> (decimal integer string=w1959:string)  [unwired: 1 in]
                n1025 = call <vilib>:"Space Constant.vi"() -> ("String"=w1960:string)
                n1026 = Concatenate Strings("MR", w1960, w1959, "\r") -> (w1957:string)
              }
            }
            n1027 = case shown="True" w1944 {
              tunnel: ["" w1950] -> w1942
              frame False {
              }
              frame True {
                n1028 = property on="R Scan Length SP steps" class="DigNum (strict)"() -> ("Value"=w1955:i32)  [unwired: 2 in, 2 out]
                n1029 = Number To Decimal String(number=w1955) -> (decimal integer string=w1952:string)  [unwired: 1 in]
                n1030 = call <vilib>:"Space Constant.vi"() -> ("String"=w1953:string)
                n1031 = Concatenate Strings("MR", w1953, w1952, "\r") -> (w1950:string)
              }
            }
          }
          frame #1 {
            n1032 = case shown="False" w1985 {
              tunnel: [w2016 w2021] -> w1993
              tunnel: [w2015 w2020] -> w1992
              tunnel: w1996 -> [_ w2019]
              tunnel: w1984 -> [w2016 w2018]
              tunnel: w1983 -> [w2015 w2017]
              frame False {
              }
              frame True {
                n1033 = VISA Write(VISA resource name=w2018, write buffer=w2019, error in (no error)=w2017) -> (VISA resource name out=w2021:refnum<visa-resource-name>, error out=w2020:errorcluster)  [unwired: 1 out]
              }
            }
            n1034 = case shown="False" w1997 {
              tunnel: [w2023 w2028] -> w2000
              tunnel: [w2022 w2027] -> w1999
              tunnel: w1998 -> [_ w2026]
              tunnel: w1982 -> [w2023 w2025]
              tunnel: w1981 -> [w2022 w2024]
              frame False {
              }
              frame True {
                n1035 = VISA Write(VISA resource name=w2025, write buffer=w2026, error in (no error)=w2024) -> (VISA resource name out=w2028:refnum<visa-resource-name>, error out=w2027:errorcluster)  [unwired: 1 out]
              }
            }
            n1036 = case shown="False" w1988 {
              tunnel: [w2009 w2014] -> w1987
              tunnel: [w2008 w2013] -> w1986
              tunnel: w1995 -> [_ w2012]
              tunnel: w1980 -> [w2009 w2011]
              tunnel: w1979 -> [w2008 w2010]
              frame False {
              }
              frame True {
                n1037 = VISA Write(VISA resource name=w2011, write buffer=w2012, error in (no error)=w2010) -> (VISA resource name out=w2014:refnum<visa-resource-name>, error out=w2013:errorcluster)  [unwired: 1 out]
              }
            }
            n1038 = case shown="False" w1991 {
              tunnel: [w2002 w2007] -> w1990
              tunnel: [w2001 w2006] -> w1989
              tunnel: w1994 -> [_ w2005]
              tunnel: w1978 -> [w2002 w2004]
              tunnel: w1977 -> [w2001 w2003]
              frame False {
              }
              frame True {
                n1039 = VISA Write(VISA resource name=w2004, write buffer=w2005, error in (no error)=w2003) -> (VISA resource name out=w2007:refnum<visa-resource-name>, error out=w2006:errorcluster)  [unwired: 1 out]
              }
            }
          }
          frame #2 {
            n1040 = call "Time Delay7"("Delay Time (s)"=0.1) -> ()  [unwired: 10 in, 1 out]
          }
          frame #3 {
            n1041 = case shown="True" w2054 {
              tunnel: w2056 -> [w2081 w2085]
              tunnel: w2055 -> [w2080 w2084]
              tunnel: [w2081 w2083] -> w2043
              tunnel: [w2080 w2082] -> w2042
              frame False {
              }
              frame True {
                n1042 = property class="Instr"(reference=w2085, error in=w2084) -> (reference out=w2087:refnum<visa-resource-name>, error out=w2086:errorcluster, "Serial Settings:Number of Bytes at Serial Port"=w2088:u32)
                n1043 = VISA Read(VISA resource name=w2087, byte count=w2088, error in (no error)=w2086) -> (VISA resource name out=w2083:refnum<visa-resource-name>, error out=w2082:errorcluster)  [unwired: 2 out]
              }
            }
            n1044 = case shown="True" w2057 {
              tunnel: w2061 -> [w2090 w2094]
              tunnel: w2060 -> [w2089 w2093]
              tunnel: [w2090 w2092] -> w2059
              tunnel: [w2089 w2091] -> w2058
              frame False {
              }
              frame True {
                n1045 = property class="Instr"(reference=w2094, error in=w2093) -> (reference out=w2096:refnum<visa-resource-name>, error out=w2095:errorcluster, "Serial Settings:Number of Bytes at Serial Port"=w2097:u32)
                n1046 = VISA Read(VISA resource name=w2096, byte count=w2097, error in (no error)=w2095) -> (VISA resource name out=w2092:refnum<visa-resource-name>, error out=w2091:errorcluster)  [unwired: 2 out]
              }
            }
            n1047 = case shown="True" w2050 {
              tunnel: w2049 -> [w2063 w2067]
              tunnel: w2048 -> [w2062 w2066]
              tunnel: [w2063 w2065] -> w2047
              tunnel: [w2062 w2064] -> w2046
              frame False {
              }
              frame True {
                n1048 = property class="Instr"(reference=w2067, error in=w2066) -> (reference out=w2069:refnum<visa-resource-name>, error out=w2068:errorcluster, "Serial Settings:Number of Bytes at Serial Port"=w2070:u32)
                n1049 = VISA Read(VISA resource name=w2069, byte count=w2070, error in (no error)=w2068) -> (VISA resource name out=w2065:refnum<visa-resource-name>, error out=w2064:errorcluster)  [unwired: 2 out]
              }
            }
            n1050 = case shown="True" w2053 {
              tunnel: w2052 -> [w2072 w2076]
              tunnel: w2051 -> [w2071 w2075]
              tunnel: [w2072 w2074] -> w2045
              tunnel: [w2071 w2073] -> w2044
              frame False {
              }
              frame True {
                n1051 = property class="Instr"(reference=w2076, error in=w2075) -> (reference out=w2078:refnum<visa-resource-name>, error out=w2077:errorcluster, "Serial Settings:Number of Bytes at Serial Port"=w2079:u32)
                n1052 = VISA Read(VISA resource name=w2078, byte count=w2079, error in (no error)=w2077) -> (VISA resource name out=w2074:refnum<visa-resource-name>, error out=w2073:errorcluster)  [unwired: 2 out]
              }
            }
          }
          frame #4 {
            n1053 = property on="R Scan" class="Bool (strict)"("Val(Sgnl)"=FALSE ("Slew Ready 2")) -> ()  [unwired: 2 in, 2 out]
            n1054 = property on="Z Scan" class="Bool (strict)"("Val(Sgnl)"=FALSE ("Slew Ready 2")) -> ()  [unwired: 2 in, 2 out]
            n1055 = property on="X Scan" class="Bool (strict)"("Val(Sgnl)"=FALSE ("Slew Ready 2")) -> ()  [unwired: 2 in, 2 out]
            n1056 = property on="Y Scan" class="Bool (strict)"("Val(Sgnl)"=FALSE ("Slew Ready 2")) -> ()  [unwired: 2 in, 2 out]
            n1057 = property on="Z Scan Velocity SP steps/sec" class="DigNum (strict)"("DisabledEnum"=T2."Enabled" ("Disabled")) -> ()  [unwired: 2 in, 2 out]
            n1058 = property on="X Scan Length SP steps" class="DigNum (strict)"("DisabledEnum"=T2."Enabled" ("Disabled")) -> ()  [unwired: 2 in, 2 out]
            n1059 = property on="Y Scan Selocity SP steps/sec" class="DigNum (strict)"("DisabledEnum"=T2."Enabled" ("Disabled")) -> ()  [unwired: 2 in, 2 out]
            n1060 = property on="Z Scan Length SP steps" class="DigNum (strict)"("DisabledEnum"=T2."Enabled" ("Disabled")) -> ()  [unwired: 2 in, 2 out]
            n1061 = property on="Y Scan Length SP steps" class="DigNum (strict)"("DisabledEnum"=T2."Enabled" ("Disabled")) -> ()  [unwired: 2 in, 2 out]
            n1062 = property on="X Scan Velocity SP steps/sec" class="DigNum (strict)"("DisabledEnum"=T2."Enabled" ("Disabled")) -> ()  [unwired: 2 in, 2 out]
            n1063 = property on="R Scan Velocity SP steps/sec" class="DigNum (strict)"("DisabledEnum"=T2."Enabled" ("Disabled")) -> ()  [unwired: 2 in, 2 out]
            n1064 = property on="R Scan Length SP steps" class="DigNum (strict)"("DisabledEnum"=T2."Enabled" ("Disabled")) -> ()  [unwired: 2 in, 2 out]
            n1065 = property on="Scan Go" class="Bool"("DisabledEnum"=T2."Disabled and Grayed Out" ("Disabled")) -> ()  [unwired: 2 in, 2 out]
            n1066 = property on="Scan Cancel" class="Bool"("DisabledEnum"=T2."Disabled and Grayed Out" ("Disabled")) -> ()  [unwired: 2 in, 2 out]
          }
        }
      }
      event "Reset": Mouse Down {
        n1067 = event-data() -> ()  [unwired: 1 in, 7 out]
        n1068 = flat-sequence {
          tunnel: [w2150] -> w2129
          tunnel: w2130 -> [w2153]
          tunnel: [w2152] -> w2128
          tunnel: w2131 -> [w2151]
          frame #0 {
            n1069 = property on="Reset X Motor Steps" class="DigNum (strict)"() -> ("Value"=w2154:i32)  [unwired: 2 in, 2 out]
            n1070 = Number To Decimal String(number=w2154) -> (decimal integer string=w2155:string)  [unwired: 1 in]
            n1071 = call "mDrive Send Command.vi"("error in (no error)"=w2153, "Extra"=w2155, "Command"=T1."Set Current Position", "VISA resource name"=w2151) -> ("error out"=w2152:errorcluster, "VISA resource name out"=w2150:refnum<visa-resource-name>)  [unwired: 3 in, 1 out]
          }
        }
        n1072 = flat-sequence {
          tunnel: w2135 -> [w2160]
          tunnel: w2134 -> [w2159]
          tunnel: [w2158] -> w2133
          tunnel: [w2157] -> w2132
          frame #0 {
            n1073 = property on="Reset Y Motor Steps" class="DigNum (strict)"() -> ("Value"=w2161:i32)  [unwired: 2 in, 2 out]
            n1074 = Number To Decimal String(number=w2161) -> (decimal integer string=w2162:string)  [unwired: 1 in]
            n1075 = call "mDrive Send Command.vi"("error in (no error)"=w2159, "Extra"=w2162, "Command"=T1."Set Current Position", "VISA resource name"=w2160) -> ("error out"=w2157:errorcluster, "VISA resource name out"=w2158:refnum<visa-resource-name>)  [unwired: 3 in, 1 out]
          }
        }
        n1076 = flat-sequence {
          tunnel: [w2137] -> w2123
          tunnel: [w2139] -> w2122
          tunnel: w2125 -> [w2138]
          tunnel: w2124 -> [w2136]
          frame #0 {
            n1077 = property on="Reset R Motor Steps" class="DigNum (strict)"() -> ("Value"=w2140:i32)  [unwired: 2 in, 2 out]
            n1078 = Number To Decimal String(number=w2140) -> (decimal integer string=w2141:string)  [unwired: 1 in]
            n1079 = call "mDrive Send Command.vi"("error in (no error)"=w2136, "Extra"=w2141, "Command"=T1."Set Current Position", "VISA resource name"=w2138) -> ("error out"=w2139:errorcluster, "VISA resource name out"=w2137:refnum<visa-resource-name>)  [unwired: 3 in, 1 out]
          }
        }
        n1080 = flat-sequence {
          tunnel: [w2146] -> w2121
          tunnel: [w2145] -> w2120
          tunnel: w2127 -> [w2144]
          tunnel: w2126 -> [w2143]
          frame #0 {
            n1081 = property on="Reset Z Motor Steps" class="DigNum (strict)"() -> ("Value"=w2147:i32)  [unwired: 2 in, 2 out]
            n1082 = Number To Decimal String(number=w2147) -> (decimal integer string=w2148:string)  [unwired: 1 in]
            n1083 = call "mDrive Send Command.vi"("error in (no error)"=w2143, "Extra"=w2148, "Command"=T1."Set Current Position", "VISA resource name"=w2144) -> ("error out"=w2145:errorcluster, "VISA resource name out"=w2146:refnum<visa-resource-name>)  [unwired: 3 in, 1 out]
          }
        }
      }
    }
    n1084 = case shown="True" "Set Button" {
      tunnel: "Preset positions" -> [_ w490]
      frame False {
      }
      frame True {
        n1085 = property on="Presets" class="Arr (strict)"() -> ("Value"=w487:i32[][])  [unwired: 2 in, 2 out]
        n1086 = Index Array(array=w487, index (row)=w490) -> (element=w489:i32[])  [unwired: 1 in]
        n1087 = Array To Cluster(array=w489) -> (cluster=w488:T4)
        n1088 = Unbundle(w488) -> ("Value[0]"=w486:i32, "Value[1]"=w485:i32, "Value[2]"=w484:i32, "Value[3]"=w483:i32)  [unwired: 5 out]
        n1089 = property on="X Step SP" class="DigNum (strict)"("Val(Sgnl)"=w486) -> ()  [unwired: 2 in, 2 out]
        n1090 = property on="Y Step SP" class="DigNum (strict)"("Val(Sgnl)"=w485) -> ()  [unwired: 2 in, 2 out]
        n1091 = property on="Z Step SP" class="DigNum (strict)"("Val(Sgnl)"=w484) -> ()  [unwired: 2 in, 2 out]
        n1092 = property on="R Step SP" class="DigNum (strict)"("Val(Sgnl)"=w483) -> ()  [unwired: 2 in, 2 out]
      }
    }
    n1093 = case shown="True" "Add Button" {
      tunnel: w447 -> [_ w482]
      frame False {
      }
      frame True {
        n1094 = property on="X Step PV" class="DigNum (strict)"() -> ("Value"=w477:i32)  [unwired: 2 in, 2 out]
        n1095 = property on="Y Step PV" class="DigNum (strict)"() -> ("Value"=w476:i32)  [unwired: 2 in, 2 out]
        n1096 = property on="Z Step PV" class="DigNum (strict)"() -> ("Value"=w475:i32)  [unwired: 2 in, 2 out]
        n1097 = property on="R Step PV" class="DigNum (strict)"() -> ("Value"=w474:i32)  [unwired: 2 in, 2 out]
        n1098 = Build Array(w477, w476, w475, w474) -> (w480:i32[])
        n1099 = Build Array (concatenate)(w482, "String") -> (w481:string[])
        n1100 = property on="Preset positions" class="Ring (strict)"("Strings []"=w481) -> ()  [unwired: 2 in, 2 out]
        n1101 = property on="Presets" class="Arr (strict)"() -> ("Value"=w479:i32[][])  [unwired: 2 in, 2 out]
        n1102 = Build Array (concatenate)(w479, w480) -> (w473:i32[][])
        n1103 = property on="Presets" class="Arr (strict)"("Val(Sgnl)"=w473) -> ()  [unwired: 2 in, 2 out]
      }
    }
    n1104 = case shown="True" "Delete Button" {
      tunnel: w447 -> [_ w472]
      frame False {
      }
      frame True {
        n1105 = property on="Preset positions" class="Ring (strict)"() -> ("Value"=w470:i32)  [unwired: 2 in, 2 out]
        n1106 = Delete From Array(array=w472, index=w470) -> (array with subset deleted=w471:string[])  [unwired: 1 in, 1 out]
        n1107 = property on="Presets" class="Arr (strict)"() -> ("Value"=w469:i32[][])  [unwired: 2 in, 2 out]
        n1108 = Delete From Array(array=w469, index (row)=w470) -> (array with subset deleted=w468:i32[][])  [unwired: 2 in, 1 out]
        n1109 = property on="Preset positions" class="Ring (strict)"("Strings []"=w471) -> ()  [unwired: 2 in, 2 out]
        n1110 = property on="Presets" class="Arr (strict)"("Val(Sgnl)"=w468) -> ()  [unwired: 2 in, 2 out]
      }
    }
  }
  n1111 = flat-sequence {
    tunnel: w87 -> [w2169]
    tunnel: w86 -> [w2167]
    tunnel: [w2164] -> w23
    frame #0 {
      n1112 = call "mDrive Send Command.vi"("error in (no error)"=w2167, "Extra"="P", "Command"=T1."Print Parameter", "VISA resource name"=w2169) -> ("error out"=w2166:errorcluster, "read buffer"=w2173:string, "VISA resource name out"=w2168:refnum<visa-resource-name>)  [unwired: 3 in]
      n1113 = call "mDrive Send Command.vi"("error in (no error)"=w2166, "Command"=T1."Stop", "VISA resource name"=w2168) -> ("error out"=w2175:errorcluster, "VISA resource name out"=w2176:refnum<visa-resource-name>)  [unwired: 4 in, 1 out]
      n1114 = Decimal String To Number(string=w2173, offset=0) -> (number=w2165:i32)  [unwired: 1 in, 1 out]
      n1115 = To Long Integer(number=w2165) -> (32bit integer=w2164:i32)
      n1116 = VISA Close(VISA resource name=w2176, error in (no error)=w2175) -> ()  [unwired: 1 out]
    }
  }
  n1117 = flat-sequence {
    tunnel: w27 -> [w2182]
    tunnel: w26 -> [w2180]
    tunnel: [w2177] -> w22
    frame #0 {
      n1118 = call "mDrive Send Command.vi"("error in (no error)"=w2180, "Extra"="P", "Command"=T1."Print Parameter", "VISA resource name"=w2182) -> ("error out"=w2179:errorcluster, "read buffer"=w2186:string, "VISA resource name out"=w2181:refnum<visa-resource-name>)  [unwired: 3 in]
      n1119 = call "mDrive Send Command.vi"("error in (no error)"=w2179, "Command"=T1."Stop", "VISA resource name"=w2181) -> ("error out"=w2188:errorcluster, "VISA resource name out"=w2189:refnum<visa-resource-name>)  [unwired: 4 in, 1 out]
      n1120 = Decimal String To Number(string=w2186, offset=0) -> (number=w2178:i32)  [unwired: 1 in, 1 out]
      n1121 = To Long Integer(number=w2178) -> (32bit integer=w2177:i32)
      n1122 = VISA Close(VISA resource name=w2189, error in (no error)=w2188) -> ()  [unwired: 1 out]
    }
  }
  n1123 = flat-sequence {
    tunnel: w29 -> [w2195]
    tunnel: w28 -> [w2193]
    tunnel: [w2190] -> w21
    frame #0 {
      n1124 = call "mDrive Send Command.vi"("error in (no error)"=w2193, "Extra"="P", "Command"=T1."Print Parameter", "VISA resource name"=w2195) -> ("error out"=w2192:errorcluster, "read buffer"=w2199:string, "VISA resource name out"=w2194:refnum<visa-resource-name>)  [unwired: 3 in]
      n1125 = call "mDrive Send Command.vi"("error in (no error)"=w2192, "Command"=T1."Stop", "VISA resource name"=w2194) -> ("error out"=w2201:errorcluster, "VISA resource name out"=w2202:refnum<visa-resource-name>)  [unwired: 4 in, 1 out]
      n1126 = Decimal String To Number(string=w2199, offset=0) -> (number=w2191:i32)  [unwired: 1 in, 1 out]
      n1127 = To Long Integer(number=w2191) -> (32bit integer=w2190:i32)
      n1128 = VISA Close(VISA resource name=w2202, error in (no error)=w2201) -> ()  [unwired: 1 out]
    }
  }
  n1129 = flat-sequence {
    tunnel: w25 -> [w2208]
    tunnel: w24 -> [w2206]
    tunnel: [w2203] -> w20
    frame #0 {
      n1130 = call "mDrive Send Command.vi"("error in (no error)"=w2206, "Extra"="P", "Command"=T1."Print Parameter", "VISA resource name"=w2208) -> ("error out"=w2205:errorcluster, "read buffer"=w2212:string, "VISA resource name out"=w2207:refnum<visa-resource-name>)  [unwired: 3 in]
      n1131 = call "mDrive Send Command.vi"("error in (no error)"=w2205, "Command"=T1."Stop", "VISA resource name"=w2207) -> ("error out"=w2214:errorcluster, "VISA resource name out"=w2215:refnum<visa-resource-name>)  [unwired: 4 in, 1 out]
      n1132 = Decimal String To Number(string=w2212, offset=0) -> (number=w2204:i32)  [unwired: 1 in, 1 out]
      n1133 = To Long Integer(number=w2204) -> (32bit integer=w2203:i32)
      n1134 = VISA Close(VISA resource name=w2215, error in (no error)=w2214) -> ()  [unwired: 1 out]
    }
  }
  n1135 = flat-sequence {
    tunnel: w23 -> [w2221]
    tunnel: w22 -> [w2220]
    tunnel: w21 -> [w2219]
    tunnel: w20 -> [w2218]
    frame #0 {
      n1136 = Build Array(w2221, w2220, w2219, w2218) -> (w2216:i32[])
      n1137 = call-poly <vilib>:"Write To Spreadsheet File.vi"("1D data"=w2216, "file path (dialog if empty)"=path "C:/Documents and Settings/b_ogasawara/Desktop/lv1/LV codes/IMS/POS.TXT") -> ()  [unwired: 6 in, 1 out]
    }
    frame #1 {
      n1138 = property on="Presets" class="Arr (strict)"() -> ("Value"=w2228:i32[][])  [unwired: 2 in, 2 out]
      n1139 = property on="Preset positions" class="Ring (strict)"() -> ("Strings []"=w2224:string[])  [unwired: 2 in, 2 out]
      n1140 = Number To Decimal String(number=w2228) -> (decimal integer string=w2222:string[][])  [unwired: 1 in]
      n1141 = Transpose 2D Array(2D array=w2222) -> (transposed array=w2223:string[][])
      n1142 = Build Array (concatenate)(w2224, w2223) -> (w2225:string[][])
      n1143 = Transpose 2D Array(2D array=w2225) -> (transposed array=w2226:string[][])
      n1144 = call-poly <vilib>:"Write To Spreadsheet File.vi"("2D data"=w2226, "file path (dialog if empty)"=path "C:/Documents and Settings/b_ogasawara/Desktop/lv1/LV codes/IMS/PRESET.TXT") -> ()  [unwired: 6 in, 1 out]
    }
  }
